vi "Data Monitor.vi"() -> ()   [LabVIEW 2018]
uses:
  Controls/Power Analyser Enum.ctl
  Controls/DUBAS FGV STATES.ctl
  Controls/DUBAS DTALOG FGV STATES.ctl
  SubVI/Hoiki/Conotrls/States.ctl
  Controls/READ CAN DATA.ctl
  Controls/Calculated Limits.ctl
  Controls/Main Tab.ctl
  <vilib>/FPGAPlugInAG/NI 9148/niLvFpga_Open_NI 9148.vi
  <vilib>/rvi/interface/common/dynamic/niFpgaDynamicAddResources.vi
  <vilib>/FPGAPlugInAG/Dynamic/niLvFpga_Reset_Dynamic.vi
  <vilib>/Utility/xml.llb/Read From XML File(string).vi
  Global/Throttle.vi
  <vilib>/Utility/file.llb/Write Delimited Spreadsheet (string).vi
  <vilib>/rvi/errors/niLvFpgaAdjustHostInterfaceError.vi
  <vilib>/FPGAPlugInAG/Dynamic/niLvFpga_Run_Dynamic.vi
  <vilib>/rvi/interface/common/niFpgaWaitOnOcc.vi
  <vilib>/Utility/file.llb/Read Delimited Spreadsheet (string).vi
  <vilib>/FPGAPlugInAG/Dynamic/niLvFpga_Close_Dynamic.vi
  <vilib>/rvi/interface/nirviOpenFPGA/nirviOpenFPGA.xnode
  FPGA Bitfiles/MAIN MEASUREMENT.lvbitx
  <vilib>/rvi/interface/nirviMethod/nirviMethod.xnode
  <vilib>/rvi/interface/nirviReadWriteControl/nirviReadWriteControl.xnode
  <vilib>/rvi/interface/nirviCloseFPGA/nirviCloseFPGA.xnode
  <vilib>/rvi/interface/Simulation/niFpgaSimulationCallBeginRW.vi
  <vilib>/rvi/errors/niLvFpgaMergeErrorWithErrorCode.vi
  <vilib>/FPGAPlugInAG/Dynamic/niLvFpga_ReadFifo_Dynamic.vi
  NiFpgaLv.dll
  <vilib>/FPGAPlugInAG/Dynamic/niLvFpga_ConfigureFifo_Dynamic.vi
  <vilib>/FPGAPlugInAG/Dynamic/niLvFpga_StopFifo_Dynamic.vi
  <vilib>/FPGAPlugInAG/Dynamic/niLvFpga_StartFifo_Dynamic.vi
  <vilib>/Utility/file.llb/Read Delimited Spreadsheet (I64).vi
panel:
  out "deleted portion 2":dbl[](array[numeric])
  out "deleted portion":dbl[](array[numeric])
  out "error out 2":errorcluster
  out "x*y":u32
  out "Array":string[](array[string])
  out "Thermocouple Spare":cluster{"String":string, "Scalar":sgl}[](array[cluster])
  out "Thermocouple":cluster{"String":string, "Scalar":sgl}[](array[cluster])
  out "9220 AI Volt Spare":cluster{"String":string, "Scalar":sgl}[](array[cluster])
  out "9208 AI Current":cluster{"String":string, "Scalar":sgl}[](array[cluster])
  out "9220 AI  Volt  Pressure":cluster{"String":string, "Scalar":sgl}[](array[cluster])
  in  "Data log":enum16{"1 Hz", "10 Hz"}(ring)
  in  "Settings Button":bool
  in  "Tab Control":T1(tab)
  out "Speed Torque":cluster{"Numeric":dbl, "Numeric":dbl}(graph)
  out "P DC(W)":dbl format="%_3g"
  out "P123(W)":dbl format="%_3g"
  out "P3(W)":dbl format="%_3g"
  out "P2(W)":dbl format="%_3g"
  out "P1(W)":dbl format="%_3g"
  out "VOLTAGE":string
  out "CURRENT":string
  out "POWER":string
  out "CONTROL SELECTION":string
  out "HVHC SELECTION":string
  out "PA Data":dbl[](array[numeric])
  in  "precision":i16
  out "Torque":string
  in  "precision":i16
  out "Power":string
  out "Intercooler_Out_T":sgl(slide) caption="T_intercooler_Out" scale=0.0..1000.0
  out "Intercooler_In_T":sgl(slide) caption="T_Oil Gallery" scale=0.0..1000.0
  out "Exhaust_T":sgl(slide) caption="T_Intercooler _In" scale=0.0..1000.0
  out "Oil_T":sgl(slide) caption="T_Coolant _OUT" scale=0.0..1000.0
  out "Coolant_Outlet_T":sgl(slide) caption="T_Coolant _IN" scale=0.0..1000.0
  out "Coolant_Inlet_T":sgl(slide) caption="T_intercooler_out" scale=0.0..1000.0
  out "Basement_T":sgl(slide) caption="T_Exhaust_Tail pipe" scale=0.0..1000.0
  out "Thermocouple Spare":string[](array[string])
  out "Thermocouple Spare":sgl[](array[numeric])
  out "Thermocouple":string[](array[string])
  out "Thermocouple":sgl[](array[numeric])
  out "9220 AI Volt Spare":string[](array[string])
  out "9220 AI Volt Spare":sgl[](array[numeric])
  out "9208 AI Current":string[](array[string])
  out "9208 AI Current":sgl[](array[numeric])
  out "9220 AI  Volt  Pressure":string[](array[string])
  out "9220 AI  Volt  \nPressure":sgl[](array[numeric])
  out "Universal AI":string[](array[string])
  out "9219 Universal AI":sgl[](array[numeric])
  in  "Column Header":string[](array[string])=["Time", "Throttle % ", "Speed Summary", "Torque Summary", "Power", "Gear Ratio", "Engine Speed", "Engine Torque", "L Speed", "R Speed", "H Speed", "L Torque ", "R Torque ", "H Torque ", "Intercooler_In_T", "Intercooler_Out_T", "Exhaust_T", "Oil_T", "Coolant_Inlet_T", "Coolant_Outlet_T", "Basement_T", "T Spare 1", "T Spare 2", "T Spare 3", "T Spare 4", "T Spare 5", "T Spare 6", "T Spare 7", "T Spare 8", "Coolant-In_P", "Coolant-Out_P", "Exhaust_P", "Oil_P", "Intercooler-In_P", "Intercooler-Out_P", "Misc_P ", "P Spare 1", "P Spare 2", "P Spare 3", "P Spare 4", "Engine RPM "]
  out "STOP BOTH APP":bool
  out "P Spare 4":sgl
  out "P Spare 3":sgl
  out "P Spare 2":sgl
  out "P Spare 1":sgl
  out "T Spare 8":sgl
  out "T Spare 7":sgl
  out "T Spare 6":sgl
  out "T Spare 5":sgl
  out "T Spare 4":sgl
  out "T Spare 3":sgl
  out "T Spare 2":sgl
  out "T Spare 1":sgl
  in  "Gear Ratio":dbl=1.0
  out "Torque":i32
  out "Speed":i32
  in  "File Tag":string
  out "speed torque power":dbl[](array[numeric])
  out "H Speed":dbl(knob) scale=0.0..7500.0
  out "Speed Summary":dbl(knob) scale=0.0..8000.0
  out "Torque Summary":dbl(knob) scale=-500.0..1000.0
  out "Power":dbl(knob) scale=0.0..300.0
  in  "Safety Limits":bool
  in  "Alarms & warning":string(combo)
  out "RAW Mean TC":sgl[](array[numeric]) format="%#.2g"
  out "RAW Mean":sgl[](array[numeric])
  out "Mean tc":sgl[](array[numeric]) format="%#.2g"
  out "Timeout Counter":u64
  out "error out":errorcluster
  out "Engine RPM":sgl caption="Gauge"
  out "Stop All":bool
  out "Mean":sgl[](array[numeric]) format="%#.2g"
  out "AI0":sgl
  out "AI1":sgl
  out "AI2":sgl
  out "Mod1/CH0":sgl
  out "Mod1/CH1":sgl
  out "Mod1/CH2":sgl
  out "Mod1/CH3":sgl
  out "Intercooler-Out_P":sgl(slide) caption="P_Exhaust_TailPipe" scale=0.0..10.0 scale format="%#1_6g"
  out "Misc_P":sgl(slide) caption="P_Before cat" scale=0.0..10.0 scale format="%#1_6g"
  out "Oil_P":sgl(slide) caption="P_Intercooler_In" scale=0.0..10.0 scale format="%#1.1g"
  out "Exhaust_P":sgl(slide) caption="P_Coolant_OUT" scale=0.0..5.0 scale format="%#1_6g"
  out "Coolant-Out_P":sgl(slide) caption="P_Oil Gallery" scale=0.0..5.0
  out "Intercooler-In_P":sgl(slide) caption="P_Intercooler_out" scale=0.0..10.0 scale format="%2d"
  out "Coolant-In_P":sgl(slide) caption="P_Coolant_IN" scale=0.0..5.0
  in  "Data_Log":bool
  out "Saftey_Lim_error":bool
  in  "Stop":bool
  # "NVH TEST DATA MONITOR"
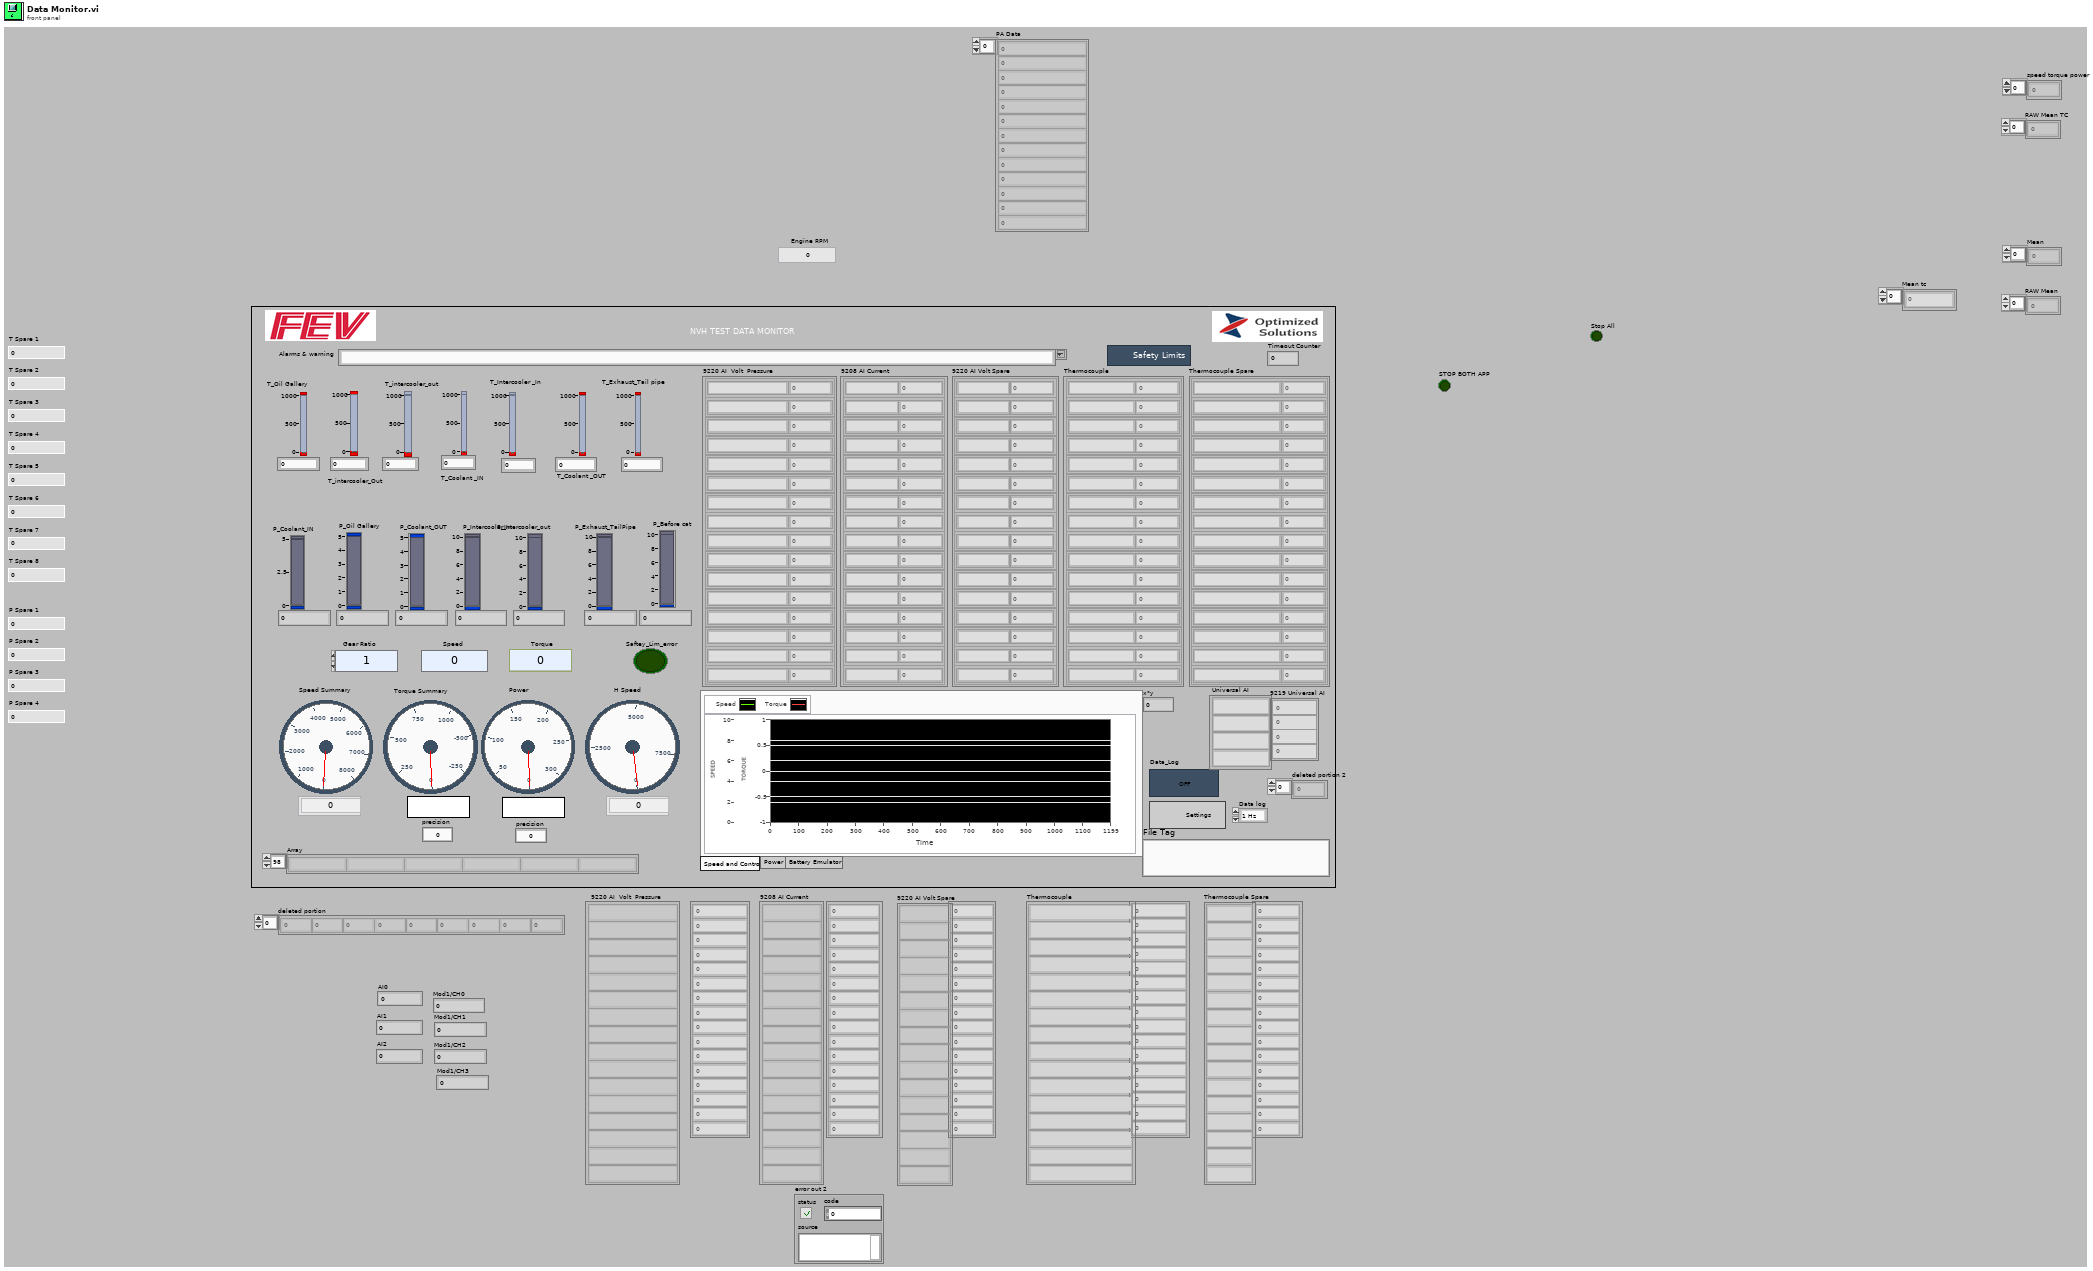
[diagram p1: front panel]
types:
  T1 = enum32{"Speed and Control", "Power", "Battery Emulator"}
  T2 = typedef "DUBAS FGV STATES.ctl" = enum16{"OPEN REF", "READ DATA", "CLOSE"}
  T3 = cluster{"Item":enum16{"Urms", "Umn", "Uac", "Udc", "Ufnd", "Upk+", "Upk-", "Uthd", "Urf", "Uunb", "Irms", "Imn", "Iac", "Idc", "Ifnd", "Ipk+", "Ipk-", "Ithd", "Irf", "Iunb", "P", "S", "Q", "PF", "DEG U", "DEG I", "DEG P", "f", "EFFI", "LOSS", "IH+", "IH-", "IH", "WP+", "WP-", "WP", "CH A", "CH B", "Pm", "Slip", "Laptime", "Laptime(ms)"}, "Ch(0:Ch1)":enum16{"1", "2", "3", "4", "12", "34", "123"}}[]
  T4 = typedef "Power Analyser Enum.ctl" = enum16{"READ", "WRITE"}
  T5 = typedef "States.ctl" = enum16{"Open Com", "Read Data", "Close Comm"}
  T6 = enum16{"Initialise", "Read Data", "Write Data", "Close"}
  T7 = enum32{"Invalid", "Standard", "Closed", "Hidden", "Minimized", "Maximized"}
  T8 = enum32{"invalid app kind", "Development System", "Run Time System", "Student Edition", "Embedded LabVIEW", "Evaluation", "Custom"}
  T9 = typedef "Calculated Limits.ctl" = cluster{"1LF":dbl, "1HW select":bool, "1LW select":bool, "1LF select":bool, "1HW":dbl, "1LW":dbl, "1HF":dbl, "1HF select":bool, "CH1":string, "1_LF_EVENT":string, "1_HF_EVENT":string}
  T10 = typedef "Limit Paths.ctl" = cluster{"Limit 1 Config Path":path, "Limit 2 Config Path ":path, "Limit 3 Config Path ":path, "Limit 4 Config Path ":path, "Limit 5 Config Path ":path, "Limit 6 Config Path ":path, "CallimitPath ":path}
  T11 = cluster{"appended path":path, "Core":cluster{"Current VI Reference":refnum<vi>, "Close Panel on Exit?":bool}, "AILimitConfig":cluster{"1LF":dbl, "1HW select":bool, "1LW select":bool, "1LF select":bool, "1HW":dbl, "1LW":dbl, "1HF":dbl, "1HF select":bool, "CH1":string, "1_LF_EVENT":string, "1_HF_EVENT":string}[], "GenHF ":string[], "GenLF ":string[], "Cal Limits":T9[], "Cal Limit Input":dbl[], "Channel Name":string[], "HF Actions":string[], "Lower Warning":string[], "Lower Fault":string[], "Higher Warning":string[], "Higher Fault":string[], "Input Values":sgl[], "Limit Path":T10, "Calculated value":sgl[], "Calculated LW ":string[], "Calculated HW ":string[], "Calculated LF ":string[], "Calculated GEN LF Events":string[], "Calculated HF ":string[], "Calculated GEN HF Events":string[], "Reset":bool}
  T12 = cluster{"1LF":dbl, "1HW select":bool, "1LW select":bool, "1LF select":bool, "1HW":dbl, "1LW":dbl, "1HF":dbl, "1HF select":bool, "CH1":string, "1_LF_EVENT":string, "1_HF_EVENT":string}[]
  T13 = cluster{"Current VI Reference":refnum<vi>, "Close Panel on Exit?":bool}
  T14 = typedef "Main Tab.ctl" = enum32{"H", "L", "R", "L-R", "H-L-R", "System"}
  T15 = typedef "DUBAS DTALOG FGV STATES.ctl" = enum16{"OPEN REF", "READ DATA", "WRITE DATA", "CLOSE"}
  T16 = enum8{"Enabled", "Disabled", "Disabled and Grayed Out"}
  T17 = typedef "READ CAN DATA.ctl" = enum16{"SET", "GET"}
  T18 = cluster{"Core":cluster{"Current VI Reference":refnum<vi>, "Close Panel on Exit?":bool}, "Intercooler_In_T":refnum<vi>, "Coolant_Inlet_T":refnum<vi>, "Coolant_Outlet_T":refnum<vi>, "Basement_T":refnum<vi>, "Exhaust_T":refnum<vi>, "Oil_T":refnum<vi>, "Intercooler_Out_T":refnum<vi>, "ExpansionChassFPGA":refnum<k20>, "Data Log":bool, "LogFile Refnum":refnum<file>, "Log Active":bool[][], "location":path}
  T19 = typedef "READ CAN CLUSTER.ctl" = cluster{"FUNCTION":string, "DATA":string}
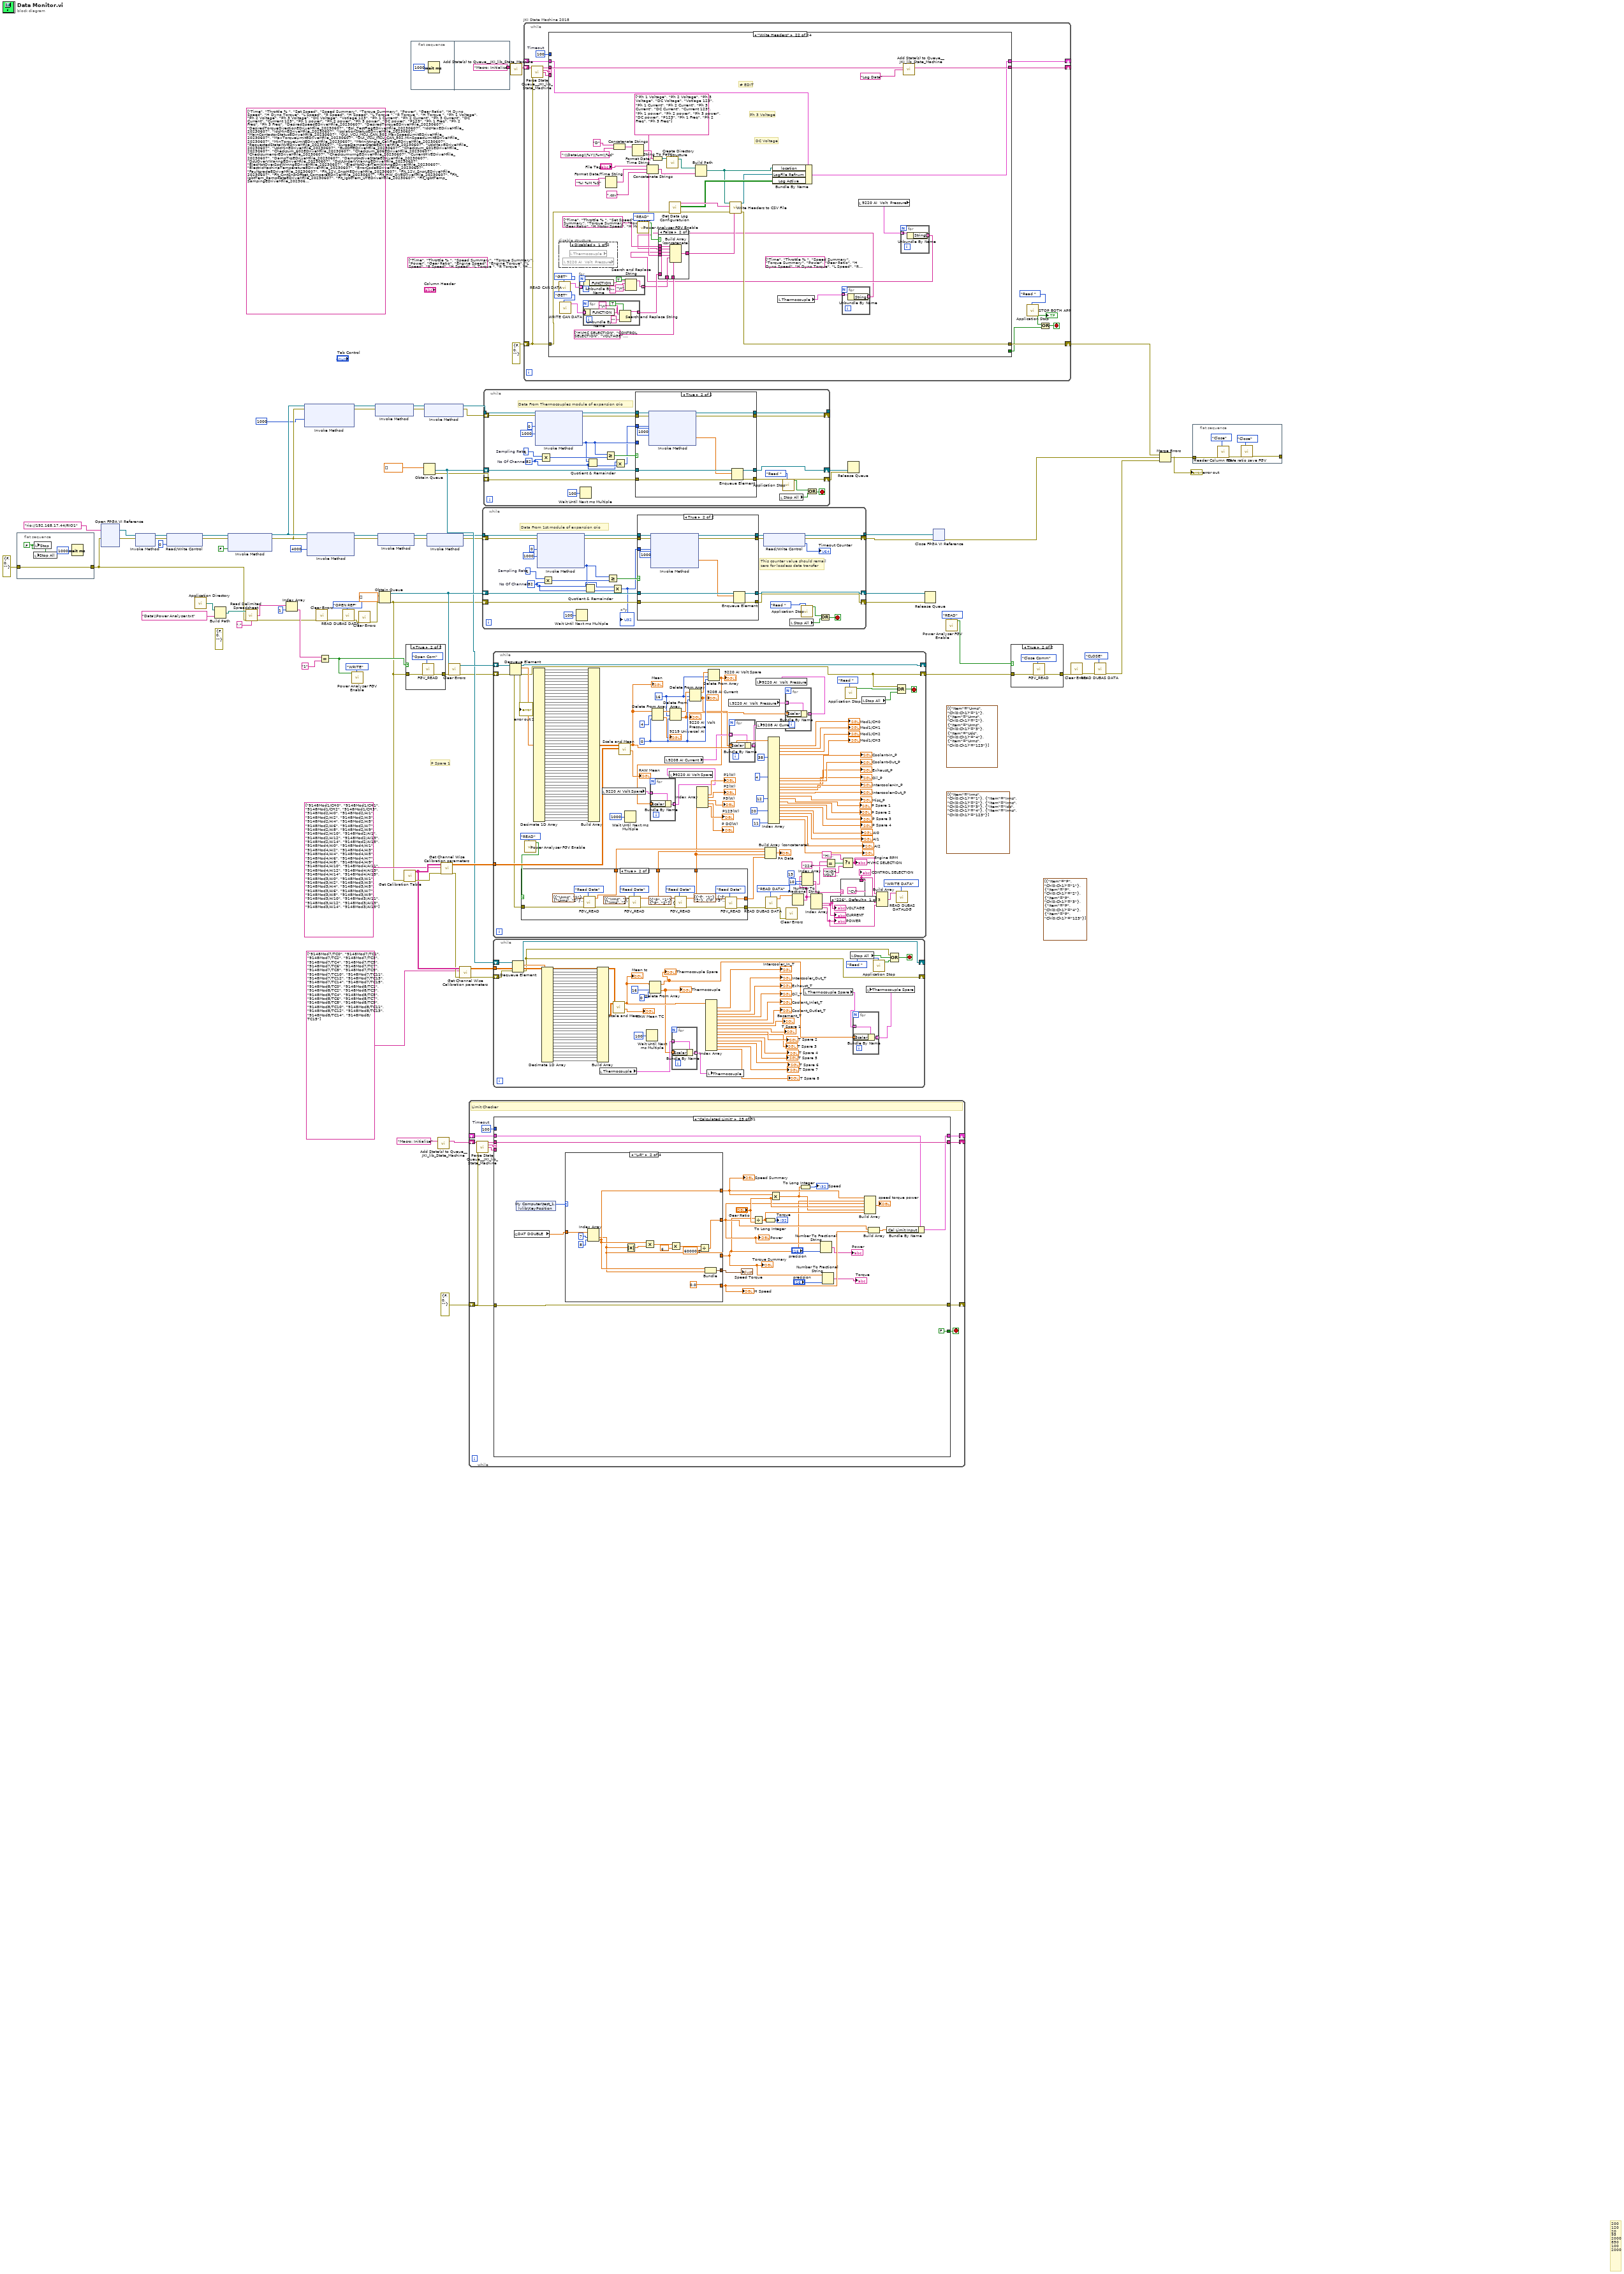
[diagram p0: block diagram]
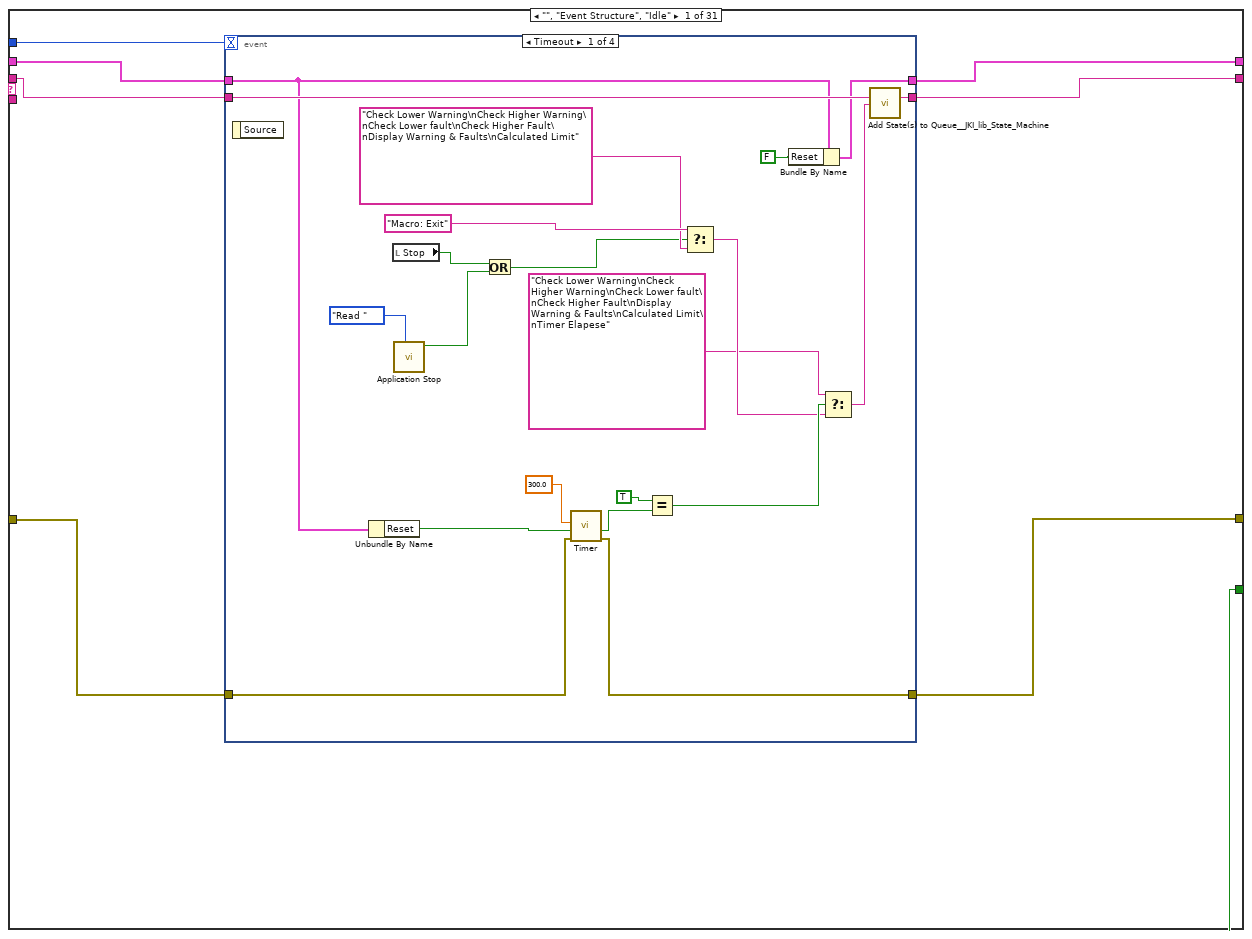
[diagram p2: hidden frame]
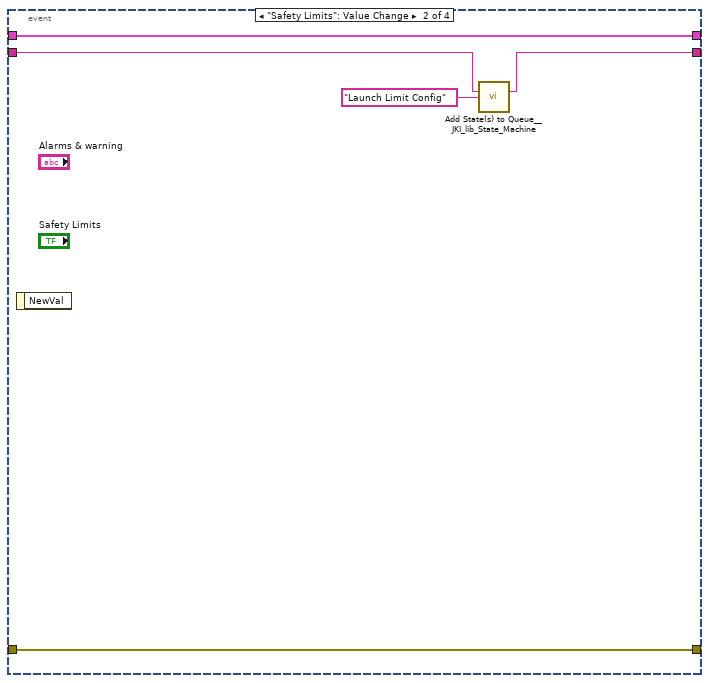
[diagram p3: hidden frame]
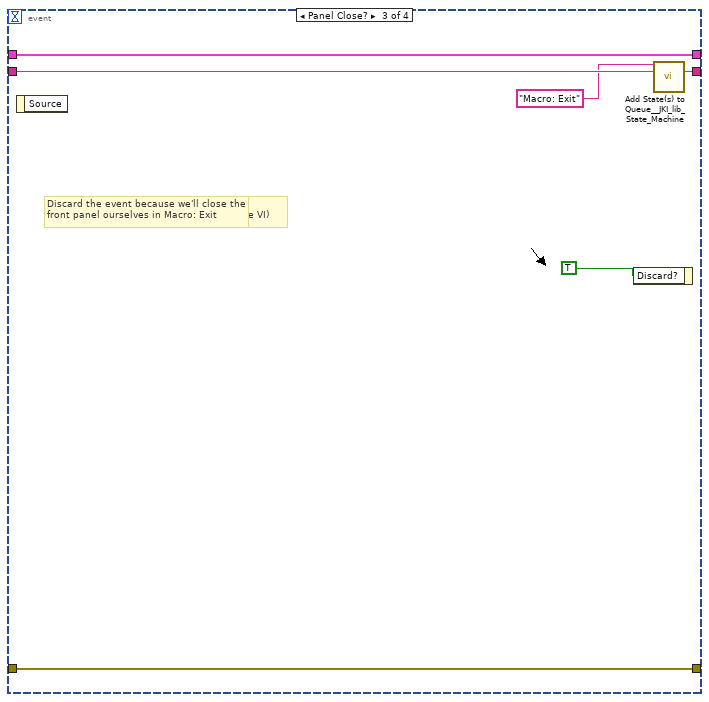
[diagram p4: hidden frame]
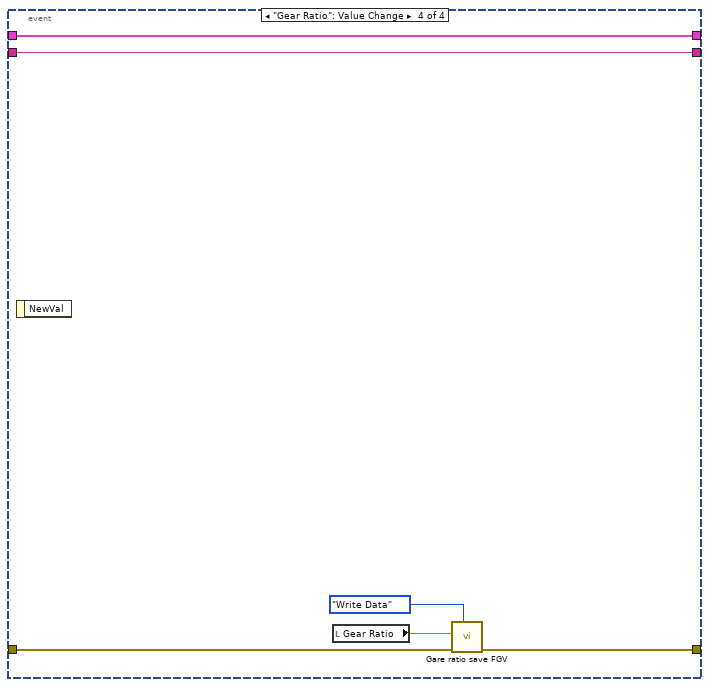
[diagram p5: hidden frame]
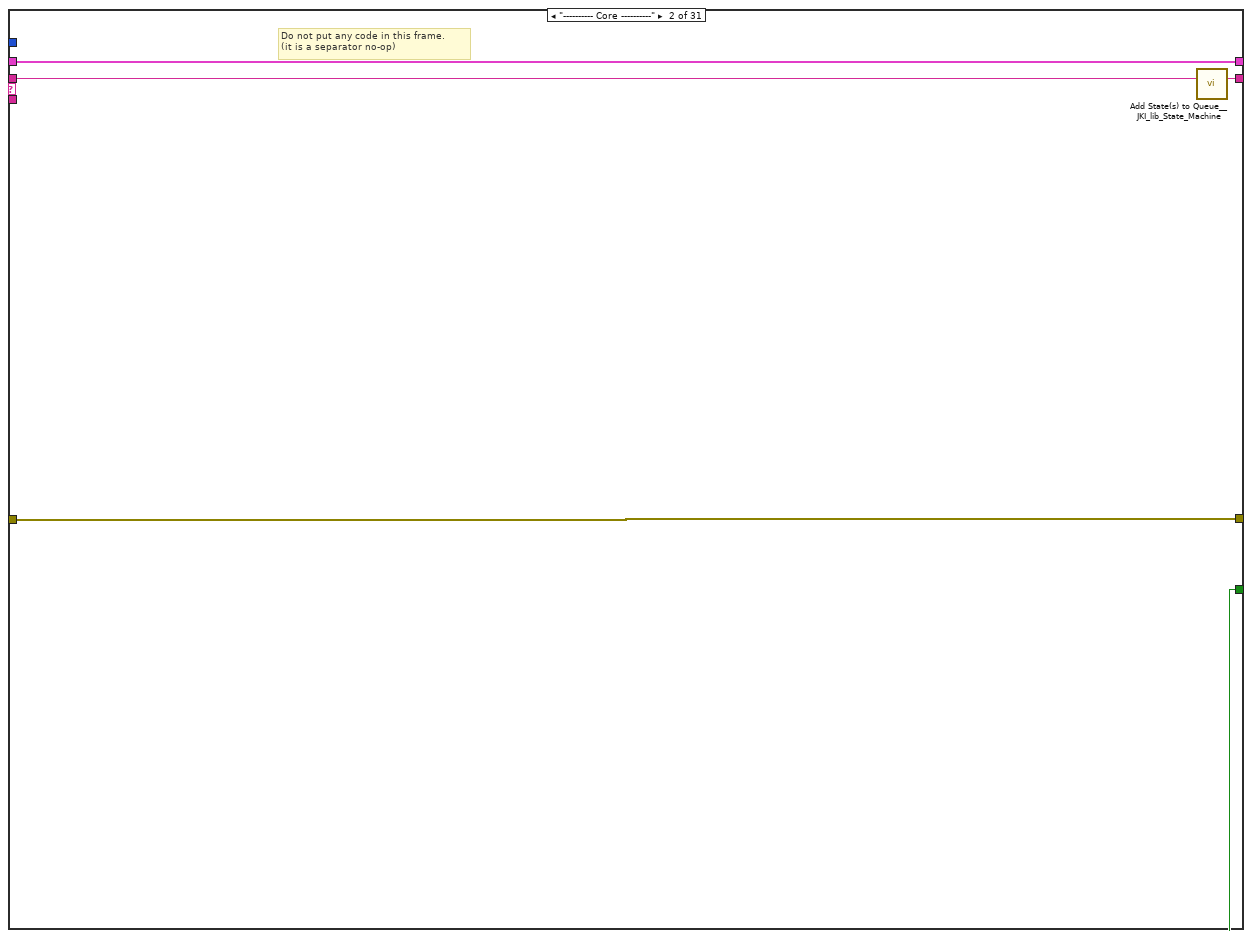
[diagram p6: hidden frame]
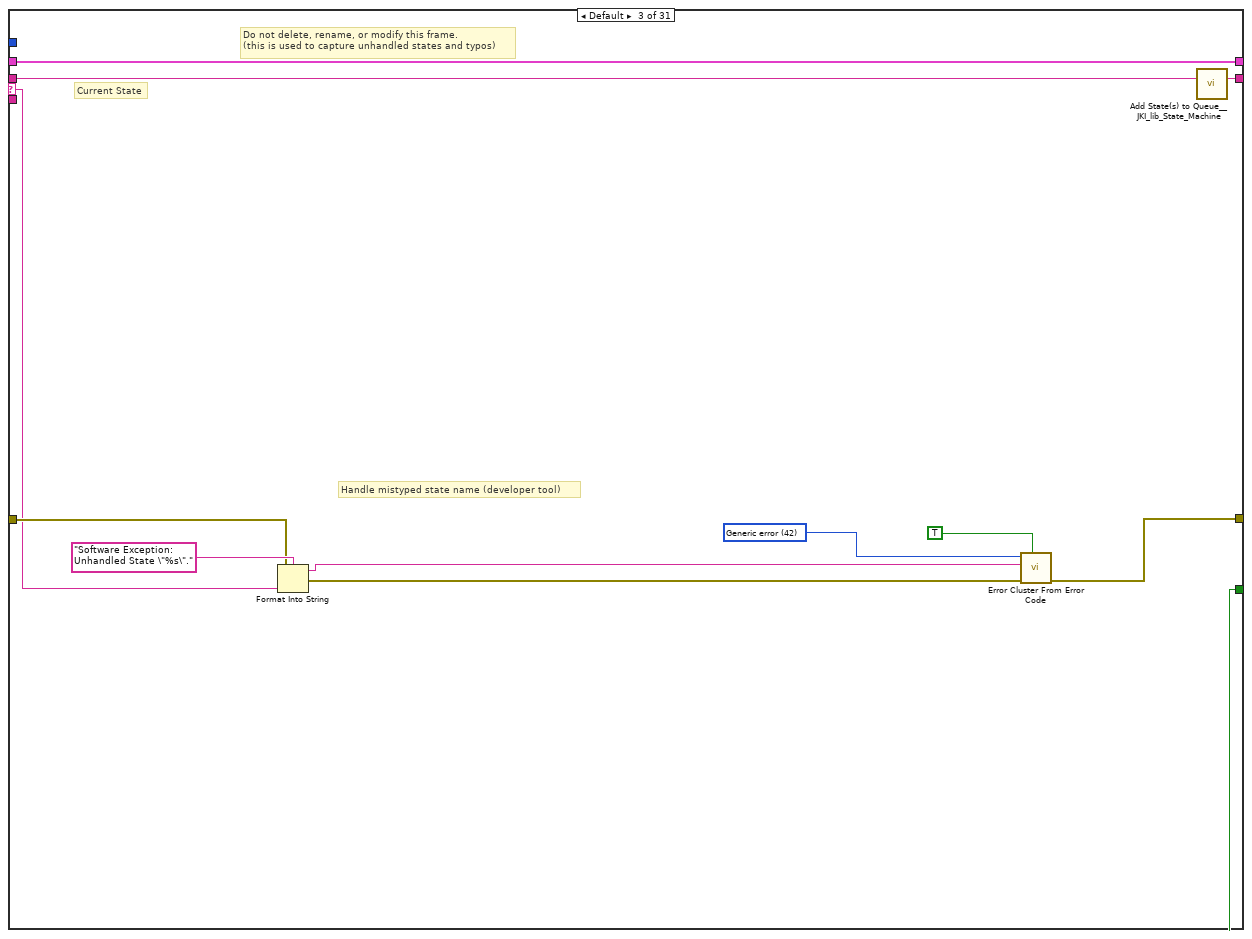
[diagram p7: hidden frame]
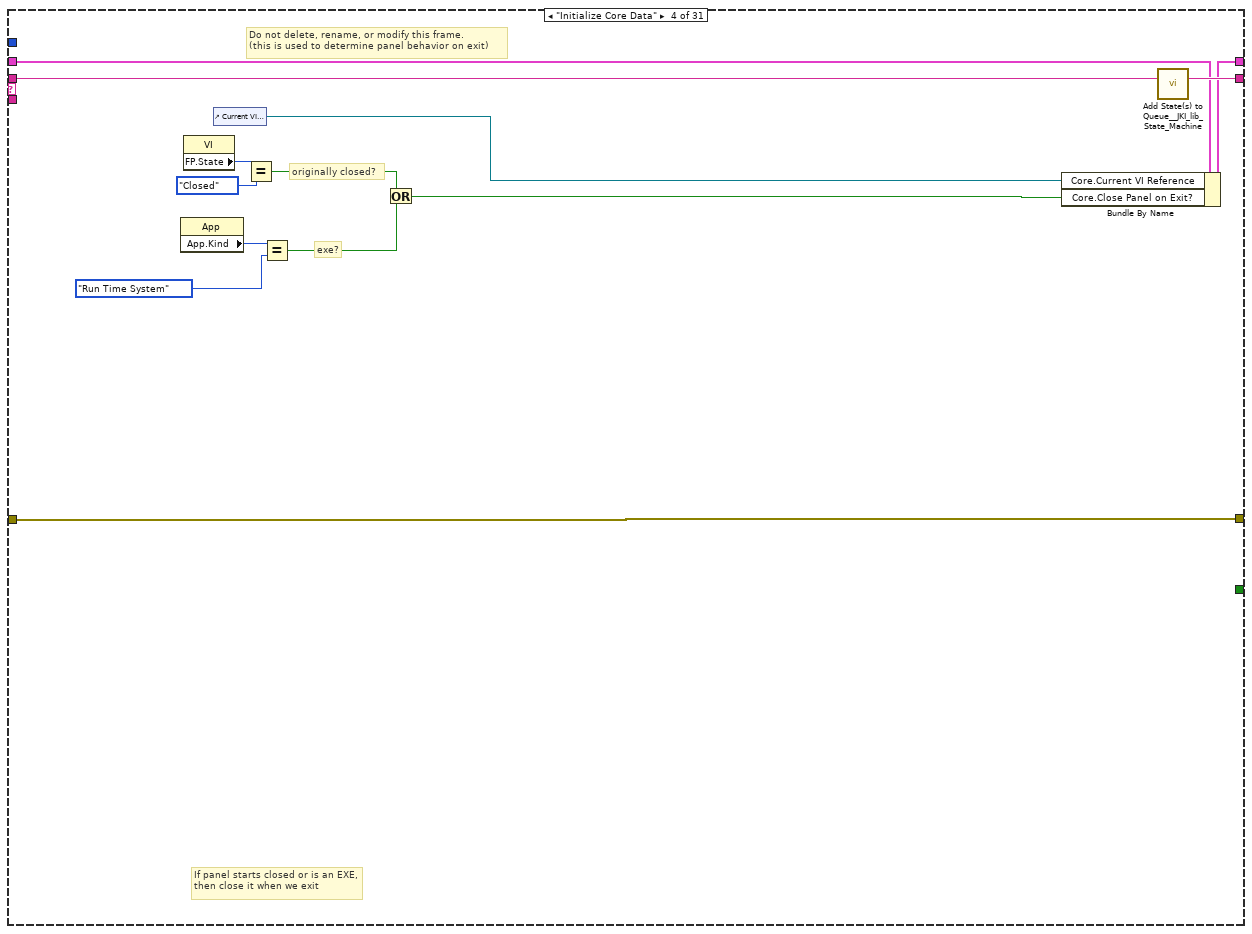
[diagram p8: hidden frame]
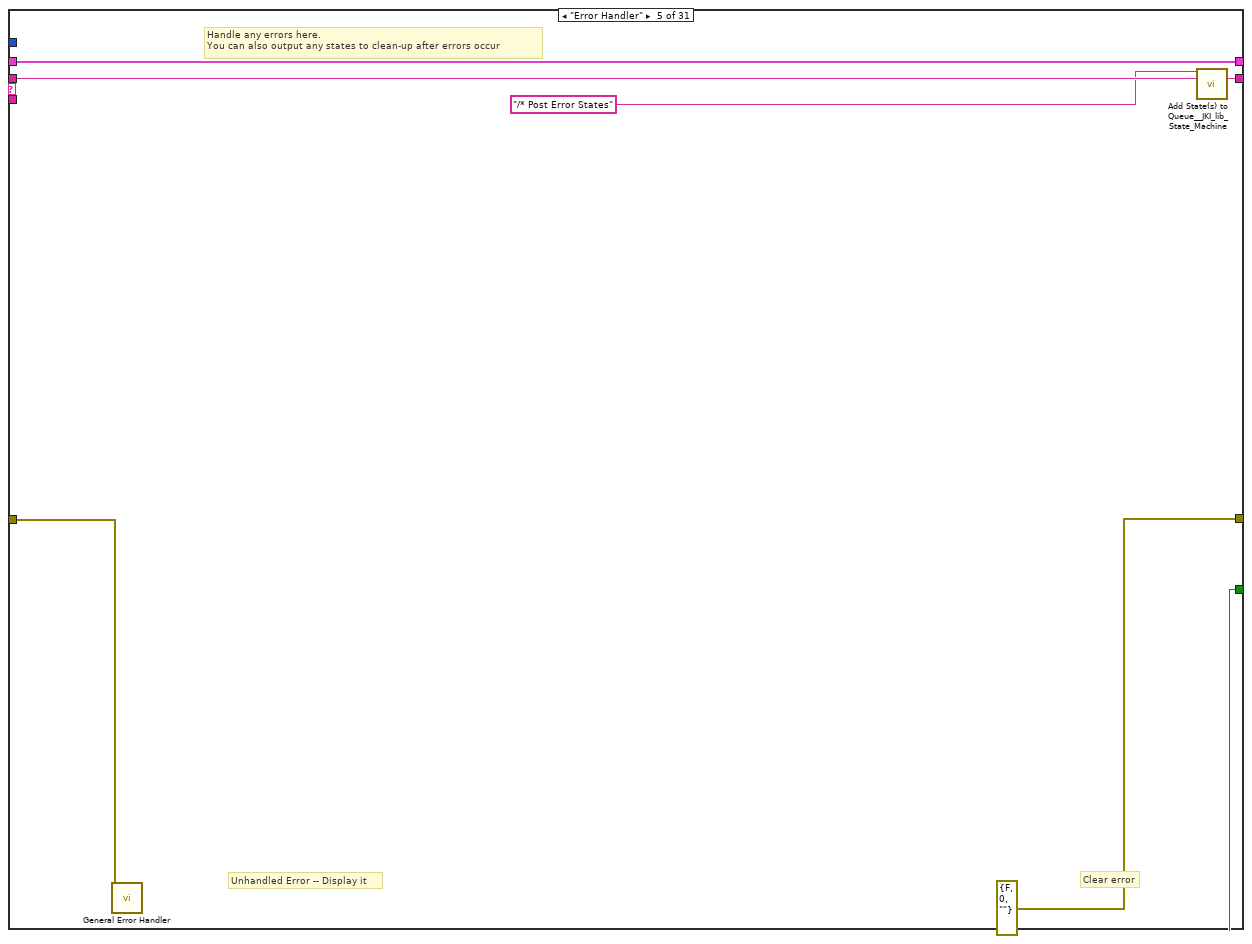
[diagram p9: hidden frame]
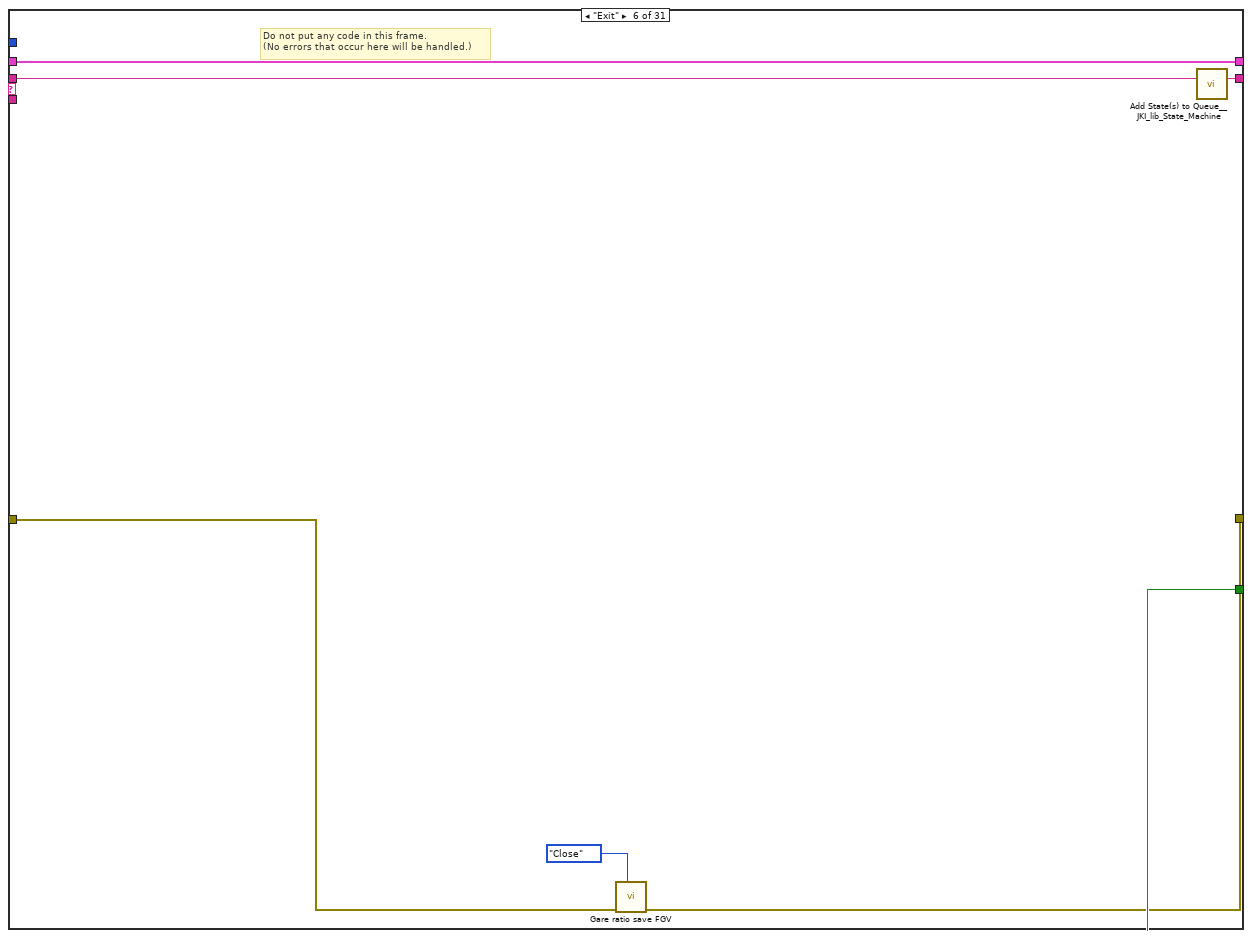
[diagram p10: hidden frame]
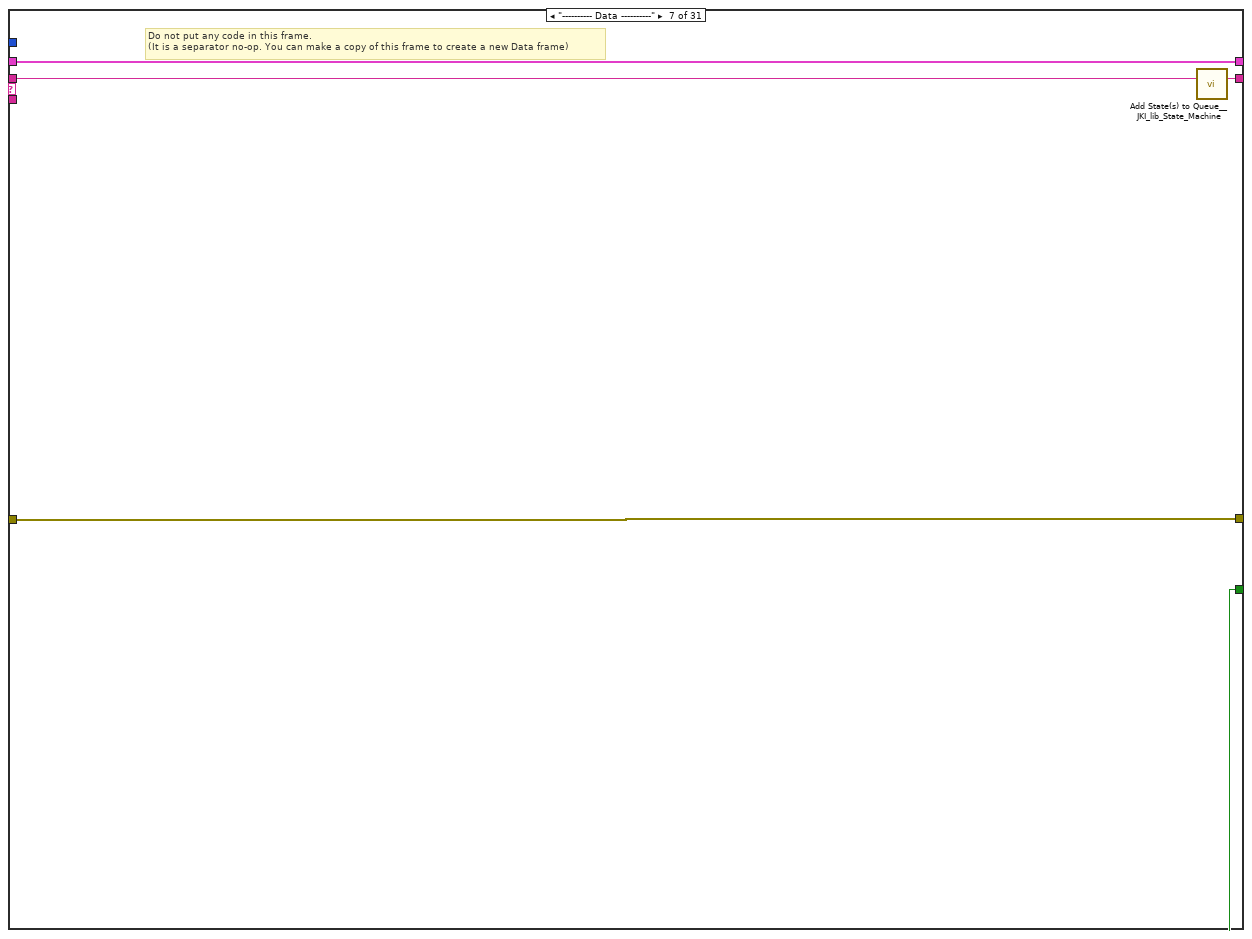
[diagram p11: hidden frame]
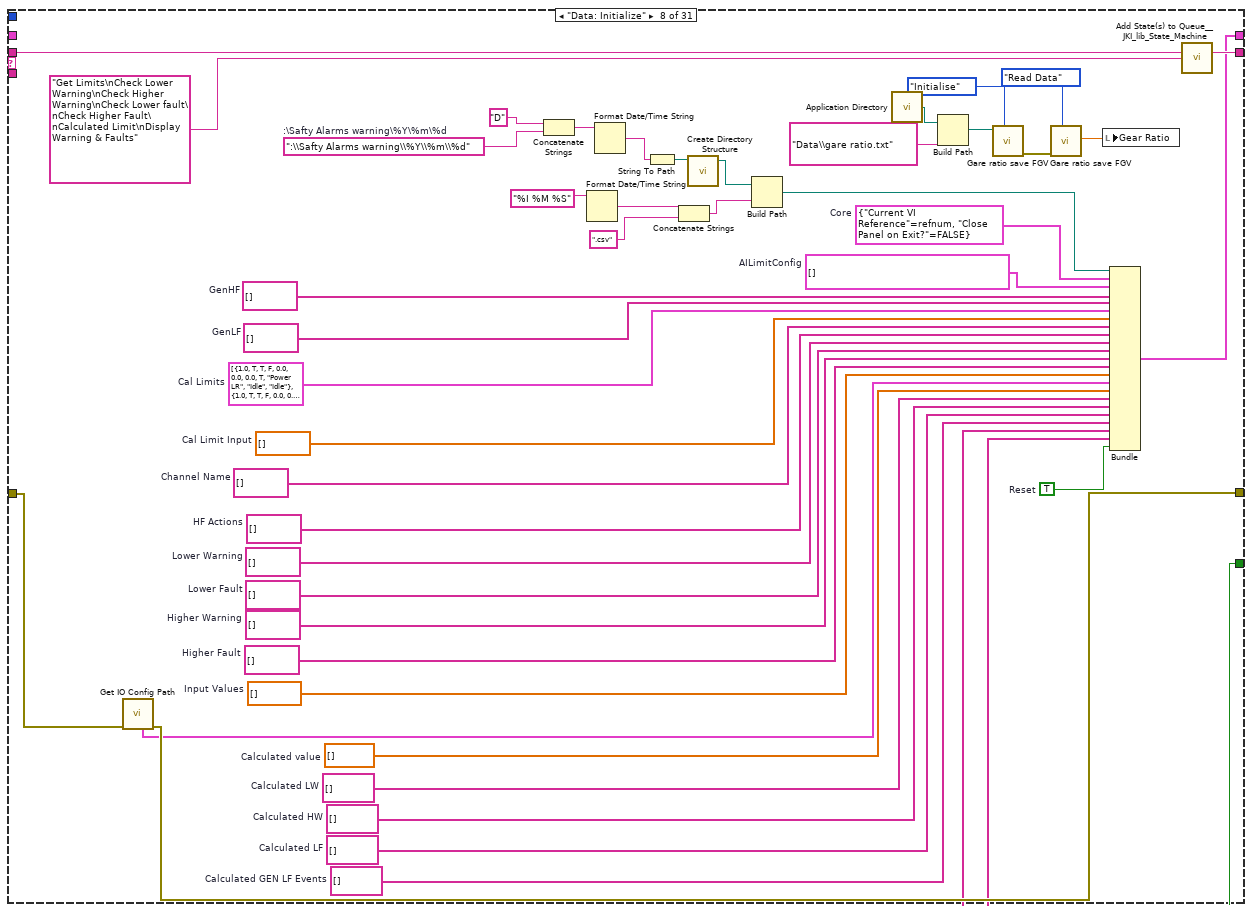
[diagram p12: hidden frame]
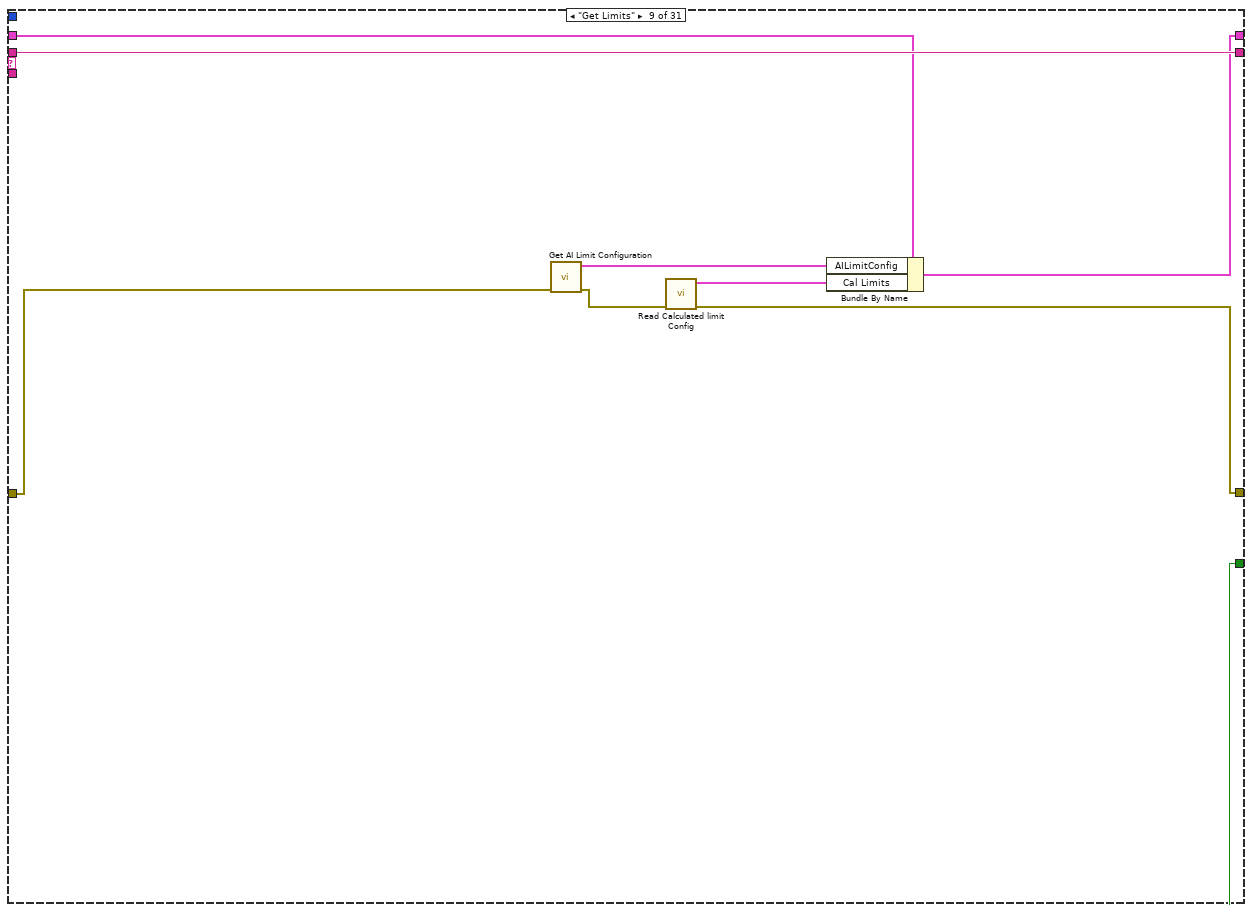
[diagram p13: hidden frame]
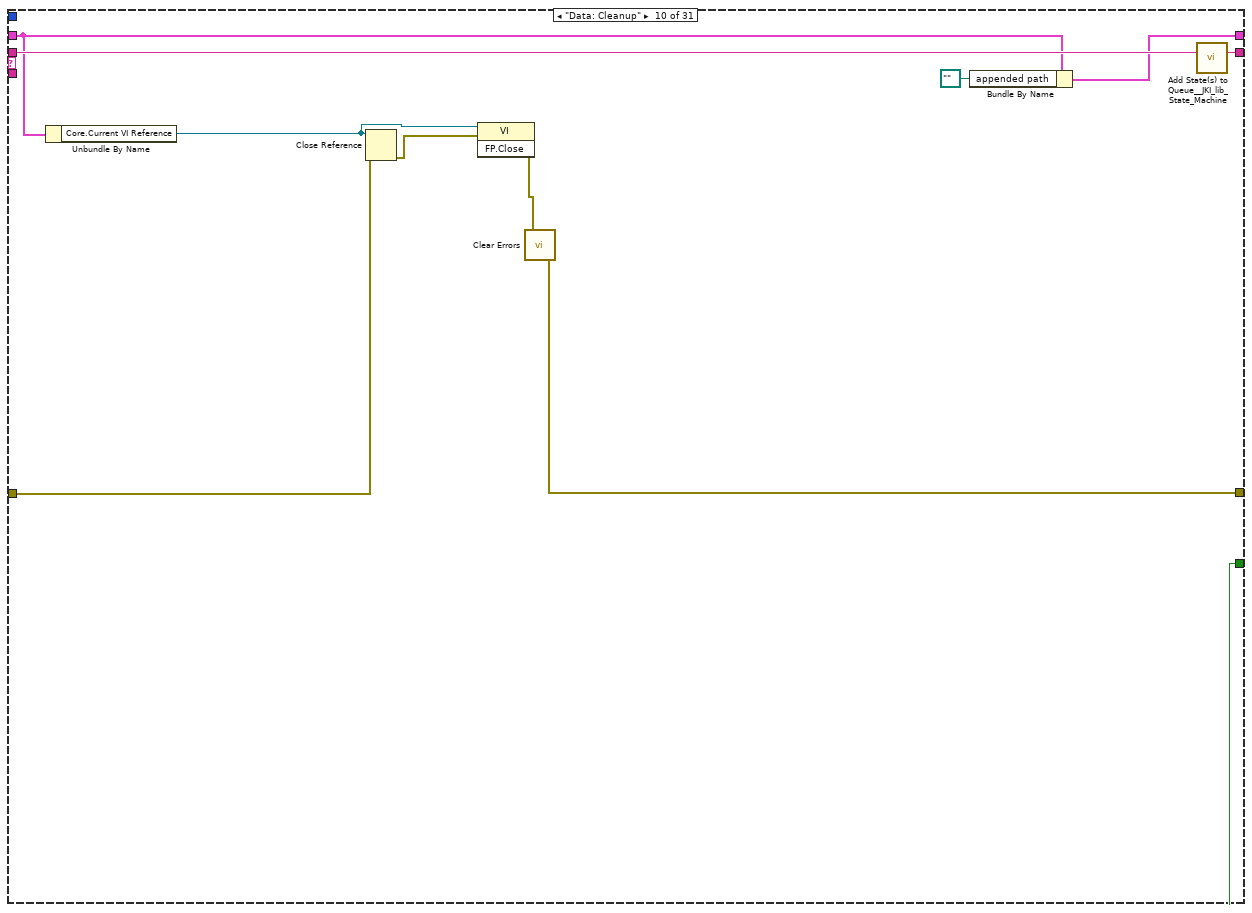
[diagram p14: hidden frame]
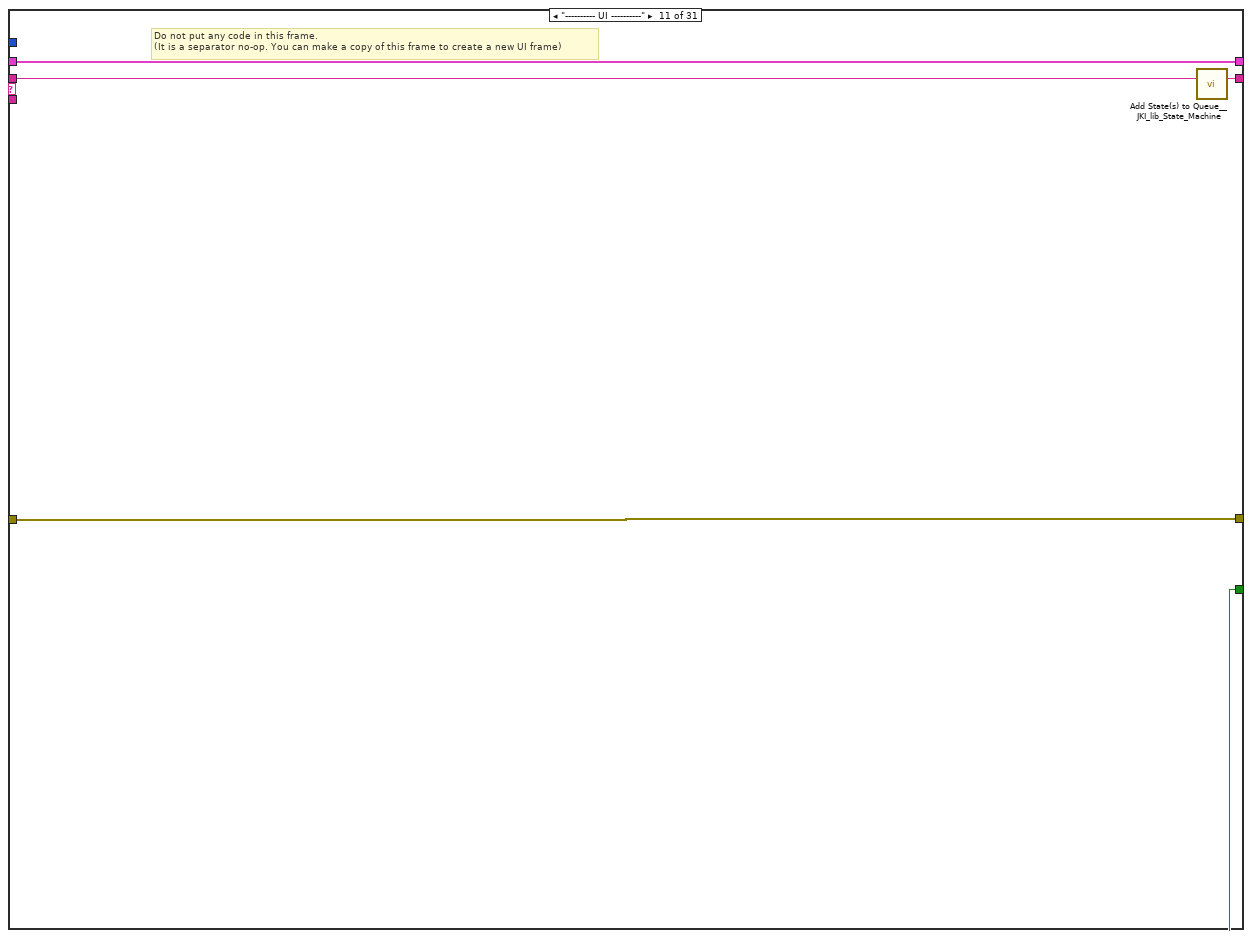
[diagram p15: hidden frame]
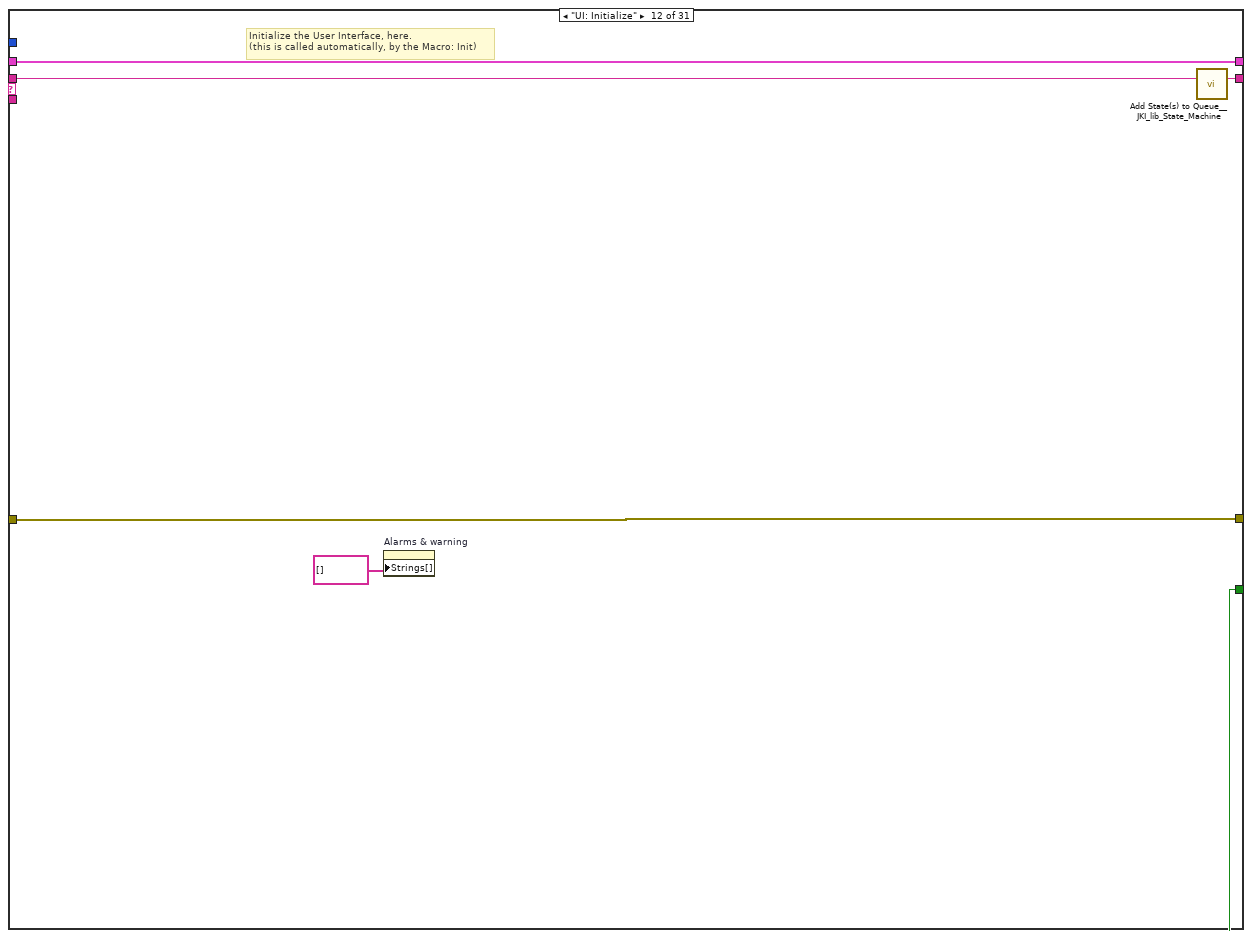
[diagram p16: hidden frame]
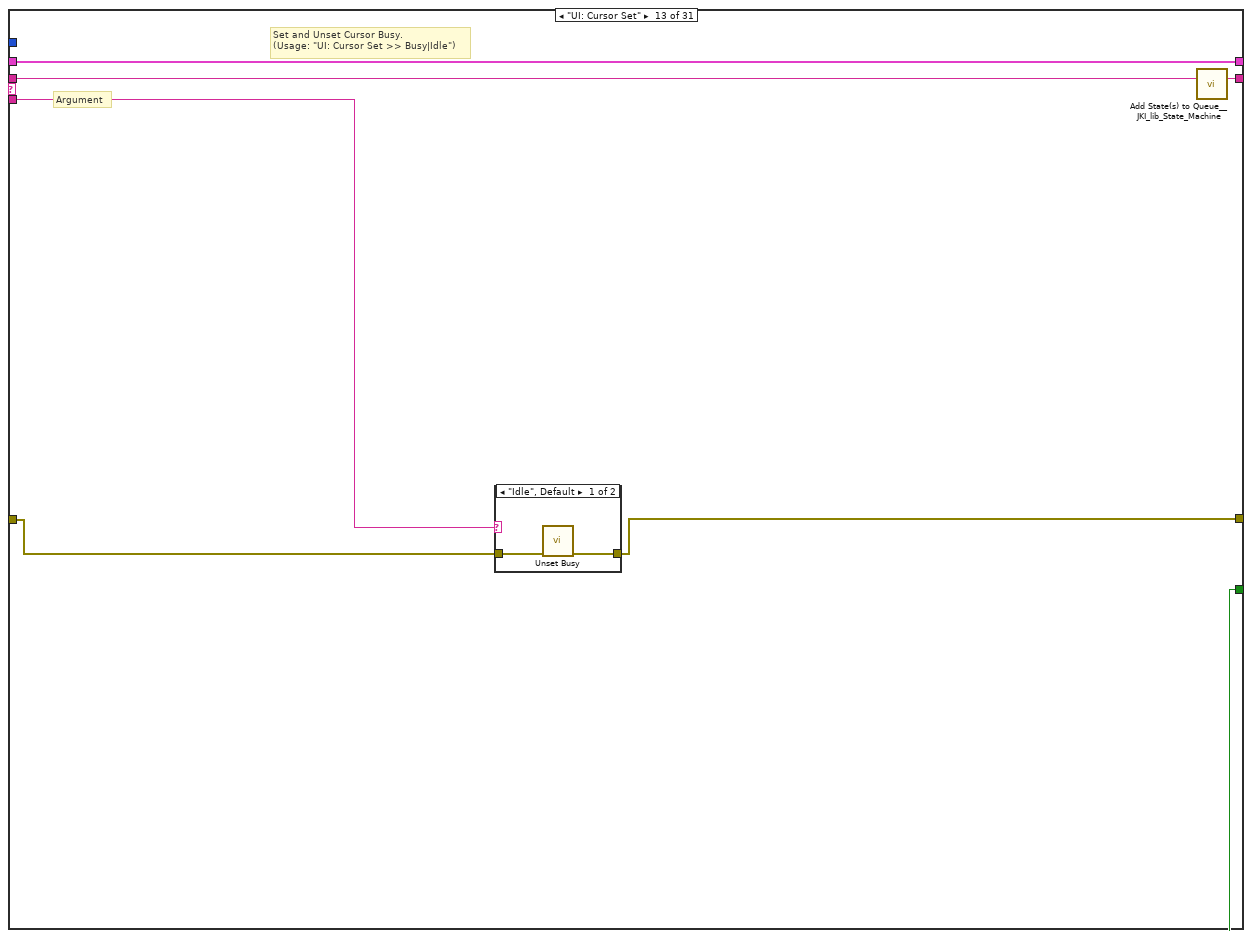
[diagram p17: hidden frame]
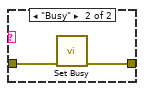
[diagram p18: hidden frame]
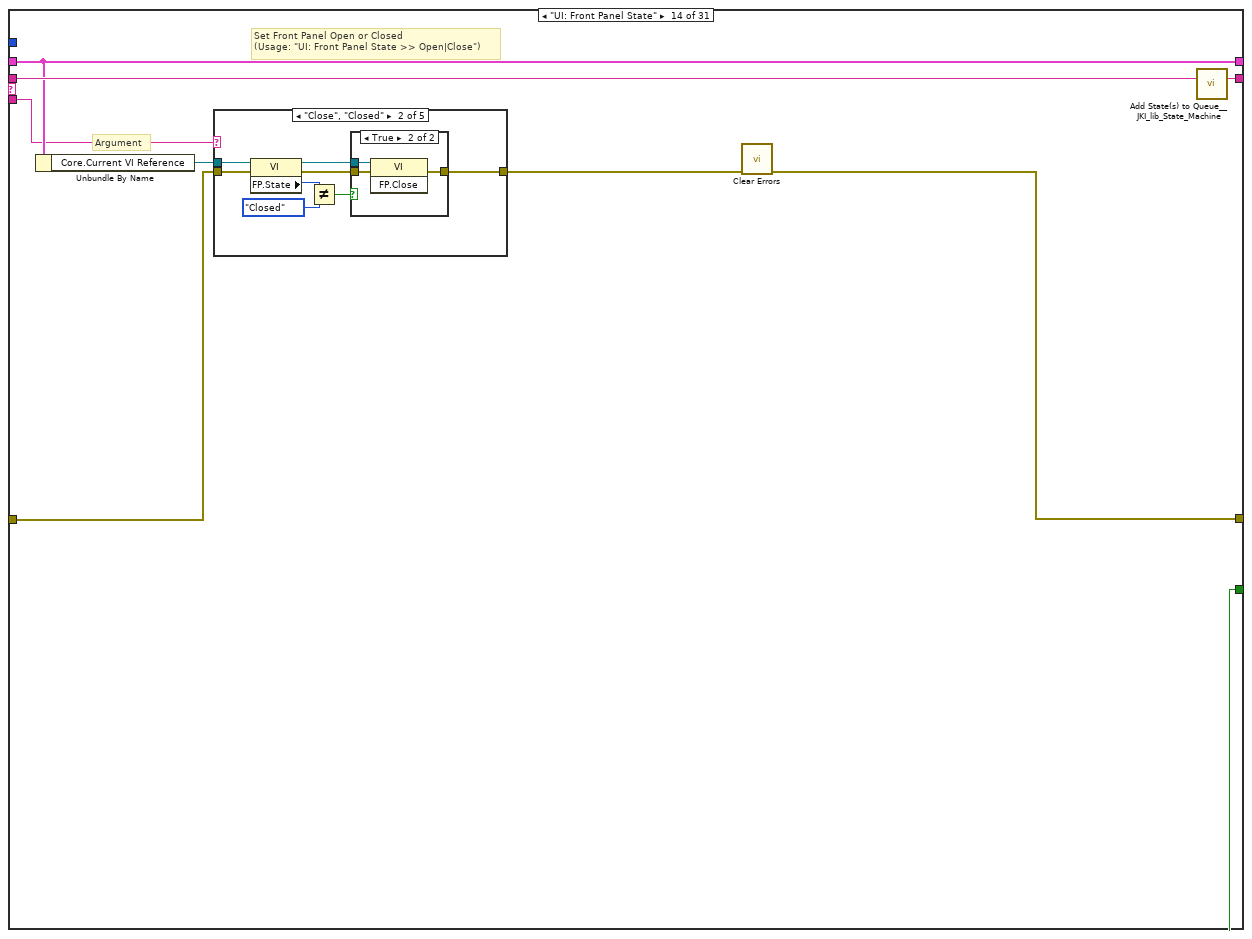
[diagram p19: hidden frame]
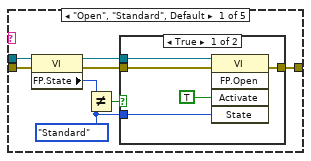
[diagram p20: hidden frame]
diagram:
  (unwired) T3 [{"Item"=enum."Urms", "Ch(0:Ch1)"=enum."1"}, {"Item"=enum."Urms", "Ch(0:Ch1)"=enum."2"}, {"Item"=enum."Urms", "Ch(0:Ch1)"=enum."3"}, {"Item"=enum."Udc", "Ch(0:Ch1)"=enum."4"}, {"Item"=enum."Urms", "Ch(0:Ch1)"=enum."123"}] ("Voltage")
  (unwired) T3 [{"Item"=enum."Irms", "Ch(0:Ch1)"=enum."1"}, {"Item"=enum."Irms", "Ch(0:Ch1)"=enum."2"}, {"Item"=enum."Irms", "Ch(0:Ch1)"=enum."3"}, {"Item"=enum."Idc", "Ch(0:Ch1)"=enum."4"}, {"Item"=enum."Irms", "Ch(0:Ch1)"=enum."123"}] ("Current")
  (unwired) errorcluster {"status"=FALSE, "code"=0, "source"=""} ("error in (no error)")
  (unwired) string[] ["Time", "Throttle % ", "Set Speed", "Speed Summary", "Torque Summary", "Power", "Gear Ratio", "H Dyno Speed", "H Dyno Torque", "L Speed", "R Speed", "H Speed", "L Torque ", "R Torque ", "H Torque ", "Ph 1 Voltage", "Ph 2 Voltage", "Ph 3 Voltage", "DC Voltage", "Votlage 123", "Ph 1 Current", "Ph 2 Current", "Ph 3 Current", "DC Current", "Currrent 123", "Ph 1 power", "Ph 2 power", "Ph 3 power", "DC power", "P123", "Ph 1 Freq", "Ph 2 Freq", "Ph 3 Freq", "DesiredSpeedEDriveMfile_20230607", "DesiredTorqueEDriveMfile_20230607", "DesiredTorqueDirectionEDriveMfile_20230607", "Eol_TestFlagEDriveMfile_20230607", "IdcMaxEDriveMfile_20230607", "IdcMinEDriveMfile_20230607", "IsolationStatusEDriveMfile_20230607", "MainContactorStatusEDriveMfile_20230607", "OUI_VCU_MCU_CAN_502.MaxSpeedLimitEDriveMfile_20230607", "MaxTorqueLimitEDriveMfile_20230607", "OUI_VCU_MCU_CAN_502.MinSpeedLimitEDriveMfile_20230607", "MinTorqueLimitEDriveMfile_20230607", "MtrInitAngle_CaliFlagEDriveMfile_20230607", "RequestedStateINVEDriveMfile_20230607", "SurgeDamperStateEDriveMfile_20230607", "UdcMaxEDriveMfile_20230607", "UdcMinEDriveMfile_20230607", "BusOffEDriveMfile_20230607", "Checksum_601EDriveMfile_20230607", "Checksum_602EDriveMfile_20230607", "Checksum_606EDriveMfile_20230607", "ChecksumerrorEDriveMfile_20230607", "ChecksumwrngEDriveMfile_20230607", "CurrentHVEDriveMfile_20230607", "DampTrqEDriveMfile_20230607", "DamptActiveStateEDriveMfile_20230607", "DcUOverVWanngEDriveMfile_20230607", "DcUUnderVWanngEDriveMfile_20230607", "ElecMotOverSpdWrnngEDriveMfile_20230607", "ElecMotOverTemWrnngEDriveMfile_20230607", "ElectricMachineTemperatureEDriveMfile_20230607", "ErrorCodeEDriveMfile_20230607", "FaultgradeEDriveMfile_20230607", "Flt_12V_SnsrHEDriveMfile_20230607", "Flt_12V_SnsrLEDriveMfile_20230607", "Flt_CrntSnsrOffset_CompareEDriveMfile_20230607", "Flt_HW_OVEDriveMfile_20230607", "Flt_IgbtTem_RampRateEDriveMfile_20230607", "Flt_IgbtTem_UTEDriveMfile_20230607", "Flt_IgbtTemp_SampingEDriveMfile_20230607", "Flt_MessageCounterEDriveMfile_20230607", "Flt_PhaseCrnt_SumEDriveMfile_20230607", "Flt_V1p3V_HEDriveMfile_20230607", "Flt_V1p3V_LEDriveMfile_20230607", "FluxWeak_FactorEDriveMfile_20230607", "IGBTOverTemWrnngEDriveMfile_20230607", "IGBTTemSnsrFltEDriveMfile_20230607", "INV12VSuppyLVEDriveMfile_20230607", "INV12VSuppyOVEDriveMfile_20230607", "INV15VSuppyLVEDriveMfile_20230607", "INV15VSuppyOVEDriveMfile_20230607", "INV5VSuppyLVEDriveMfile_20230607", "INV5VSuppyOVEDriveMfile_20230607", "INVDschrgFltEDriveMfile_20230607", "INVOverVolFltEDriveMfile_20230607", "INVPwrModuFltEDriveMfile_20230607", "INVVolSnsrFltEDriveMfile_20230607", "Id_FBEDriveMfile_20230607", "Id_RefEDriveMfile_20230607", "InitAngleOffsetEDriveMfile_20230607", "InverterTemperatureEDriveMfile_20230607", "Iq_FBEDriveMfile_20230607", "Iq_RefEDriveMfile_20230607", "LostCommWithVCUEDriveMfile_20230607", "MCU_InitialErrEDriveMfile_20230607", "MaxTorqueEDriveMfile_20230607", "MessageCounter_606EDriveMfile_20230607", "MinTorqueEDriveMfile_20230607", "MotOverCrntFltEDriveMfile_20230607", "MotOverCrntFltHardEDriveMfile_20230607", "MotOverSpdFltEDriveMfile_20230607", "MotOverTemFltEDriveMfile_20230607", "MotRotBlockFltEDriveMfile_20230607", "MotRsovrFltEDriveMfile_20230607", "MotTemSnsrFltEDriveMfile_20230607", "MtrSpdFilt_NoFiltEDriveMfile_20230607", "OutputSpeedEDriveMfile_20230607", "OutputTorqueEDriveMfile_20230607", "PhaseACrntSnsrFltEDriveMfile_20230607", "PhaseBCrntSnsrFltEDriveMfile_20230607", "PhaseCCrntSnsrFltEDriveMfile_20230607", "PowerEDriveMfile_20230607", "SW_EditionEDriveMfile_20230607", "StateEDriveMfile_20230607", "TrqRefFnlEDriveMfile_20230607", "Ud_RefEDriveMfile_20230607", "Uq_RefEDriveMfile_20230607", "VoltUsageEDriveMfile_20230607", "VoltageHVEDriveMfile_20230607", "War_IgbtTem_UTEDriveMfile_20230607", "War_MtrTem_UTEDriveMfile_20230607", "War_PhaseOverCrntEDriveMfile_20230607", "phaseA_currentEDriveMfile_20230607", "phaseB_currentEDriveMfile_20230607", "phaseC_currentEDriveMfile_20230607"] ("Headers 2")
  (unwired) T3 [{"Item"=enum."P", "Ch(0:Ch1)"=enum."1"}, {"Item"=enum."P", "Ch(0:Ch1)"=enum."2"}, {"Item"=enum."P", "Ch(0:Ch1)"=enum."3"}, {"Item"=enum."P", "Ch(0:Ch1)"=enum."4"}, {"Item"=enum."P", "Ch(0:Ch1)"=enum."123"}] ("Power")
  (unwired) string[] ["Time", "Throttle % ", "Speed Summary", "Torque Summary", "Power", "Gear Ratio", "Engine Speed", "Engine Torque", "L Speed", "R Speed", "H Speed", "L Torque ", "R Torque ", "H Torque ", "Intercooler_In_T", "Intercooler_Out_T", "Exhaust_T", "Oil_T", "Coolant_Inlet_T", "Coolant_Outlet_T", "Basement_T", "T Spare 1", "T Spare 2", "T Spare 3", "T Spare 4", "T Spare 5", "T Spare 6", "T Spare 7", "T Spare 8", "Coolant-In_P", "Coolant-Out_P", "Exhaust_P", "Oil_P", "Intercooler-In_P", "Intercooler-Out_P", "Misc_P ", "P Spare 1", "P Spare 2", "P Spare 3", "P Spare 4", "Engine RPM "] ("Column Header 2")
  # "P Spare 1"
  # "200\n120\n20\n95\n2000\n850\n100\n2000"
  n1 = flat-sequence {
    tunnel: [w81] -> w2
    tunnel: errorcluster {"status"=FALSE, "code"=0, "source"=""} ("error constant") -> [w81]
    frame #0 {
      w82 = FALSE ("Stop")
      n2 = local write "Stop All"(w82) -> ()
      n3 = local write "Stop"(w82) -> ()
      n4 = Wait (ms)(milliseconds to wait=u32 1000) -> ()  [unwired: 1 out]
    }
  }
  n5 = xnode "Open FPGA VI Reference"("error in"=w2, "resource name"=tag "rio://192.168.17.44/RIO1") -> ("FPGA VI Reference Out"=w47:refnum<k20>, "error out"=w44:errorcluster)
  n6 = xnode "Invoke Method"("FPGA VI Reference In"=w47, "error in"=w44) -> ("FPGA VI Reference Out"=w46:refnum<k20>, "error out"=w4:errorcluster)
  n7 = xnode "Read/Write Control"("FPGA VI Reference In"=w46, "Loop Rate (uS)"=u32 0) -> ("FPGA VI Reference Out"=w29:refnum<k20>)  [unwired: 1 in, 1 out]
  n8 = call <vilib>:"Application Directory.vi"() -> ("Application Directory"=w23:path)
  n9 = Build Path(base path=w23, name or relative path="Data\\Power Analyser.txt") -> (appended path=w22:path)
  n10 = xnode "Invoke Method"("FPGA VI Reference In"=w29, "error in"=w4, "Wait Until Done (F)"=FALSE) -> ("FPGA VI Reference Out"=w40:refnum<k20>, "error out"=w39:errorcluster)
  n11 = call-poly <vilib>:"Read Delimited Spreadsheet.vi"("file path (dialog if empty)"=w22, "error in (no error)"=w2, "delimiter (\\t)"="," ("delimiter (\\t)")) -> ("first row"=w20:string[], "error out"=w18:errorcluster)  [unwired: 7 in, 4 out]
  n12 = Index Array(array=w20, index=1) -> (element=w59:string)
  n13 = xnode "Invoke Method"("FPGA VI Reference In"=w40, "error in"=w39, "Requested Depth"=u32 1000) -> ("FPGA VI Reference Out"=w35:refnum<k20>, "error out"=w34:errorcluster)  [unwired: 1 out]
  n14 = xnode "Invoke Method"("FPGA VI Reference In"=w40, "error in"=w39, "Requested Depth"=u32 4000) -> ("FPGA VI Reference Out"=w51:refnum<k20>, "error out"=w50:errorcluster)  [unwired: 1 out]
  n15 = call <vilib>:"Clear Errors.vi"("error in (no error)"=w18) -> ("error out"=w10:errorcluster)  [unwired: 5 in, 1 out]
  n16 = Equal?(x=w59, y="1") -> (x = y?=w56:bool)
  n17 = call "READ DUBAS DATA.vi"("STATES"=DUBAS_FGV_STATES."OPEN REF", "error in (no error)"=w10) -> ("error out"=w9:errorcluster)  [unwired: 8 in, 1 out]
  n18 = call "Power Analyser FGV Enable.vi"("Enum"=Power_Analyser_Enum."WRITE", "Enable"=w56) -> ()  [unwired: 9 in, 1 out]
  n19 = call <vilib>:"Clear Errors.vi"("error in (no error)"=w9) -> ("error out"=w8:errorcluster)  [unwired: 5 in, 1 out]
  n20 = xnode "Invoke Method"("FPGA VI Reference In"=w35, "error in"=w34) -> ("FPGA VI Reference Out"=w36:refnum<k20>, "error out"=w37:errorcluster)
  n21 = xnode "Invoke Method"("FPGA VI Reference In"=w51, "error in"=w50) -> ("FPGA VI Reference Out"=w49:refnum<k20>, "error out"=w48:errorcluster)
  n22 = Obtain Queue(element data type=sgl[] [], error in (no error)=w8) -> (queue out=w75:refnum<queue>, error out=w3:errorcluster)  [unwired: 3 in, 1 out]
  n23 = call "Get Calibration Table.vi"("error in (no error)"=w3) -> ("error out"=w73:errorcluster, "AI Calibration Table"=w72:string[][])  [unwired: 8 in, 1 out]
  n24 = case shown="True" w56 {
    tunnel: w3 -> [w83 w85]
    tunnel: [w83 w84] -> w65
    frame False {
    }
    frame True {
      n25 = call "FGV_READ.vi"("States"=States."Open Com", "error in"=w85) -> ("error out"=w84:errorcluster)  [unwired: 8 in, 1 out]
    }
  }
  n26 = flat-sequence {
    tunnel: ["Macro: Initialize"] -> w77
    frame #0 {
      n27 = Wait (ms)(milliseconds to wait=u32 1000) -> ()  [unwired: 1 out]
    }
    frame #1 {
    }
  }
  n28 = Obtain Queue(element data type=sgl[] []) -> (queue out=w70:refnum<queue>, error out=w27:errorcluster)  [unwired: 4 in, 1 out]
  n29 = xnode "Invoke Method"("FPGA VI Reference In"=w36, "error in"=w37) -> ("FPGA VI Reference Out"=w32:refnum<k20>, "error out"=w33:errorcluster)
  n30 = xnode "Invoke Method"("FPGA VI Reference In"=w49, "error in"=w48) -> ("FPGA VI Reference Out"=w43:refnum<k20>, "error out"=w42:errorcluster)
  n31 = call <vilib>:"Add State(s) to Queue__JKI_lib_State_Machine.vi"("State(s) in (\"\")"="Macro: Initialize") -> ("States Out"=w6:string)  [unwired: 14 in]
  n32 = call "Get Channel Wise Calibration parameters.vi"("error in (no error)"=w73, "Physical Cgannel"=string[] ["9148Mod1/CH0", "9148Mod1/CH1", "9148Mod1/CH2", "9148Mod1/CH3", "9148Mod2/AI0", "9148Mod2/AI1", "9148Mod2/AI2", "9148Mod2/AI3", "9148Mod2/AI4", "9148Mod2/AI5", "9148Mod2/AI6", "9148Mod2/AI7", "9148Mod2/AI8", "9148Mod2/AI9", "9148Mod2/AI10", "9148Mod2/AI1", "9148Mod2/AI12", "9148Mod2/AI13", "9148Mod2/AI14", "9148Mod2/AI15", "9148Mod4/AI0", "9148Mod4/AI1", "9148Mod4/AI2", "9148Mod4/AI3", "9148Mod4/AI4", "9148Mod4/AI5", "9148Mod4/AI6", "9148Mod4/AI7", "9148Mod4/AI8", "9148Mod4/AI9", "9148Mod4/AI10", "9148Mod4/AI11", "9148Mod4/AI12", "9148Mod4/AI13", "9148Mod4/AI14", "9148Mod4/AI15", "9148Mod3/AI0", "9148Mod3/AI1", "9148Mod3/AI2", "9148Mod3/AI3", "9148Mod3/AI4", "9148Mod3/AI5", "9148Mod3/AI6", "9148Mod3/AI7", "9148Mod3/AI8", "9148Mod3/AI9", "9148Mod3/AI10", "9148Mod3/AI11", "9148Mod3/AI12", "9148Mod3/AI13", "9148Mod3/AI14", "9148Mod3/AI15"] ("Array"), "Calibration Table"=w72) -> ("error out"=w71:errorcluster, "Slop & Offset"=w74:sgl[][])  [unwired: 6 in, 1 out]
  n33 = call <vilib>:"Clear Errors.vi"("error in (no error)"=w65) -> ("error out"=w1:errorcluster)  [unwired: 5 in, 1 out]
  n34 = call "Get Channel Wise Calibration parameters.vi"("error in (no error)"=w71, "Physical Cgannel"=string[] ["9148Mod7/TC0", "9148Mod7/TC1", "9148Mod7/TC2", "9148Mod7/TC3", "9148Mod7/TC4", "9148Mod7/TC5", "9148Mod7/TC6", "9148Mod7/TC7", "9148Mod7/TC8", "9148Mod7/TC9", "9148Mod7/TC10", "9148Mod7/TC11", "9148Mod7/TC12", "9148Mod7/TC13", "9148Mod7/TC14", "9148Mod7/TC15", "9148Mod8/TC0", "9148Mod8/TC1", "9148Mod8/TC2", "9148Mod8/TC3", "9148Mod8/TC4", "9148Mod8/TC5", "9148Mod8/TC6", "9148Mod8/TC7", "9148Mod8/TC8", "9148Mod8/TC9", "9148Mod8/TC10", "9148Mod8/TC11", "9148Mod8/TC12", "9148Mod8/TC13", "9148Mod8/TC14", "9148Mod8/TC15"] ("Array"), "Calibration Table"=w72) -> ("error out"=w17:errorcluster, "Slop & Offset"=w16:sgl[][])  [unwired: 6 in, 1 out]
  n35 = while "JKI State Machine 2018" {
    shift-right: [w92] -> _
    shift-left: _ -> [w91]
    shift-right: [w95] -> _
    shift-left: errorcluster {"status"=FALSE, "code"=0, "source"=""} ("error IO") -> [w89]
    shift-right: [w94] -> _
    shift-left: w6 -> [w96]
    stop <- w93 stop-if-true
    w90 = 100  # Timeout
    # "Limit Checker"
    n36 = call <vilib>:"Parse State Queue__JKI_lib_State_Machine.vi"("State Queue"=w96, "Error In (no error)"=w89) -> ("Remaining States"=w98:string, "Current State"=w99:string, "Arguments"=w97:string)  [unwired: 11 in]
    n37 = case shown="\"Calculated Limit\"" w99 {
      selector: w99 -> [_ _ w152 _ _ _ _ _ _ _ _ _ _ _ _ _ _ _ _ _ _ _ _ _ _ _ _ _ _ _ _]
      tunnel: w98 -> [w107 w150 w156 w175 w182 w189 w194 w241 w250 w261 w266 w272 w279 w292 w362 w416 w457 w462 w485 w499 w515 w531 w557 w598 w624 w678 w692 w703 w714 w717 w725]
      tunnel: w97 -> [_ _ _ _ _ _ _ _ _ _ _ _ w274 w286 _ _ _ _ _ _ _ _ _ _ _ _ _ _ _ _ _]
      tunnel: w91 -> [w105 w147 w154 w168 w179 w187 w191 _ w249 w255 w263 w270 w277 w288 w359 w414 w454 w459 w478 w497 w513 w529 w536 w601 w621 w669 w683 w696 w707 w718 w724]
      tunnel: [w104 w148 w158 w172 errorcluster {"status"=FALSE, "code"=0, "source"=""} ("error out") w184 w192 w236 w245 w251 w264 w269 w275 w284 w360 w381 w455 w460 w483 w488 w505 w517 w538 w599 w613 w675 w689 w700 w711 w716 w720] -> w95
      tunnel: w89 -> [w103 w148 w157 w172 w178 w185 w192 w237 w244 w259 w264 w269 w276 w290 w360 w373 w455 w460 w483 w492 w507 w523 w568 w600 w613 w676 w690 w701 w712 w716 w721]
      tunnel: [w106 w149 w155 w174 w181 w188 w193 w240 w250 w260 w265 w271 w278 w291 w361 w415 w456 w461 w484 w498 w514 w530 w557 w597 w624 w678 w692 w703 w714 w717 w725] -> w94
      tunnel: [FALSE FALSE FALSE _ FALSE TRUE FALSE FALSE FALSE FALSE FALSE FALSE FALSE FALSE FALSE FALSE FALSE FALSE FALSE FALSE FALSE FALSE FALSE FALSE FALSE _ FALSE FALSE FALSE FALSE FALSE] -> w93
      tunnel: [w102 w147 w154 w173 w179 w187 w191 w239 w248 w253 w263 w270 w277 w288 w359 w414 w454 w459 w477 w496 w512 w528 w534 w601 w619 w666 w680 w694 w705 w718 w722] -> w92
      tunnel: w90 -> [w101 _ _ _ _ _ _ _ _ _ _ _ _ _ _ _ _ _ _ _ _ _ _ _ _ _ _ _ _ _ _]
      frame "", "Event Structure", "Idle" {
        n38 = event shown="[0] Timeout" {
          selector: _ -> [_ _ _ _]
          dyn-events: _ -> [_ _ _ _]
          timeout: w101 -> [_ _ _ _]
          tunnel: w107 -> [w128 w131 w139 w140]
          tunnel: [w127 w130 w138 w140] -> w106
          tunnel: w105 -> [w114 w132 w136 w141]
          tunnel: [w123 w133 w137 w142] -> w104
          tunnel: w103 -> [w124 w133 w137 w143]
          tunnel: [w112 w132 w136 w141] -> w102
          event Timeout {
            n39 = event-data() -> ()  [unwired: 1 in, 1 out]
            n40 = Unbundle By Name(w114) -> ("Reset"=w121:bool)
            n41 = local read "Stop"() -> (w111:bool)
            n42 = call "Application Stop.vi"("Command"=enum16{"Read ", "Write "}."Read ") -> ("STOP"=w109:bool)  [unwired: 9 in, 1 out]
            n43 = Or(x=w111, y=w109) -> (x .or. y?=w110:bool)
            n44 = call "Timer.vi"("error in (no error)"=w124, "Reset"=w121, "Target Time"=300.0) -> ("error out"=w123:errorcluster, "Elapsed?"=w120:bool)  [unwired: 6 in, 1 out]
            n45 = Equal?(x=TRUE, y=w120) -> (x = y?=w118:bool)
            n46 = Select(t="Macro: Exit", s=w110, f="Check Lower Warning\nCheck Higher Warning\nCheck Lower fault\nCheck Higher Fault\nDisplay Warning & Faults\nCalculated Limit" ("State(s) at Back (\"\")")) -> (s? t:f=w117:string)
            n47 = Bundle By Name(cluster=w114, "Reset"=FALSE) -> (w112:T11)
            n48 = Select(t="Check Lower Warning\nCheck Higher Warning\nCheck Lower fault\nCheck Higher Fault\nDisplay Warning & Faults\nCalculated Limit\nTimer Elapese" ("State(s) at Back (\"\")"), s=w118, f=w117) -> (s? t:f=w115:string)
            n49 = call <vilib>:"Add State(s) to Queue__JKI_lib_State_Machine.vi"("State(s) in (\"\")"=w128, "State(s) at Back (\"\")"=w115) -> ("States Out"=w127:string)  [unwired: 13 in]
          }
          event "Safety Limits": Value Change {
            n50 = event-data() -> ()  [unwired: 1 in, 1 out]
            n51 = call <vilib>:"Add State(s) to Queue__JKI_lib_State_Machine.vi"("State(s) in (\"\")"=w131, "State(s) at Back (\"\")"="Launch Limit Config" ("State(s) at Back (\"\")")) -> ("States Out"=w130:string)  [unwired: 13 in]
          }
          event Panel Close? {
            # "Discard the event because we'll close the front panel ourselves in Macro: Exit"
            # "Close Panel button (pressed) Event\n(this executes Macro: Exit to terminate the VI)"
            n52 = event-data() -> ()  [unwired: 1 in, 1 out]
            n53 = event-data("Discard?"=TRUE) -> ()  [unwired: 1 in, 1 out]
            n54 = call <vilib>:"Add State(s) to Queue__JKI_lib_State_Machine.vi"("State(s) in Front (\"\")"="Macro: Exit", "State(s) in (\"\")"=w139) -> ("States Out"=w138:string)  [unwired: 13 in]
          }
          event "Gear Ratio": Value Change {
            n55 = event-data() -> ()  [unwired: 1 in, 1 out]
            n56 = local read "Gear Ratio"() -> (w144:dbl)
            n57 = call "Gare ratio save FGV.vi"("Command"=T6."Write Data", "error in (no error)"=w143, "Gear Ratio"=w144) -> ("error out"=w142:errorcluster)  [unwired: 7 in, 1 out]
          }
        }
      }
      frame "---------- Core ----------" {
        # "Do not put any code in this frame.\n(it is a separator no-op)"
        n58 = call <vilib>:"Add State(s) to Queue__JKI_lib_State_Machine.vi"("State(s) in (\"\")"=w150) -> ("States Out"=w149:string)  [unwired: 14 in]
      }
      frame Default {
        w161 = 42 items=["No error", "Argument error", "Memory is full", "Out of zone", "End of file", "File already open", "Generic file I/O error", "File not found", "File permission error", "Disk is full", "Duplicate path", "Too many files open", "System feature not enabled", "Resource file not found", "Cannot add resource", "Resource not found", "Image not found", "Image memory error", "Pen does not exist", "Config type invalid", "Config token not found", "Config parse error", "Config memory error", "Bad external code format", "Bad external code offset", "External code not present", "Null window", "Destroy window error", "Null menu", "Print aborted", "Bad print record", "Print driver error", "Windows error during printing", "Memory error during printing", "Print dialog error", "Generic print error", "Invalid device refnum", "Device not found", "Device parameter error", "Device unit error", "Cannot open device", "Device call aborted", "Generic error", "Cancelled by user", "Object ID too low", "Object ID too high", "Object not in heap", "Unknown heap", "Unknown object (invalid DefProc)", "Unknown object (DefProc not in table)", "Message out of range", "Invalid (null) method", "Unknown message", "Manager call not supported", "Bad address", "Network operation in progress", "Network operation timed out", "Connection is busy", "Network attribute not supported", "Network error", "Address in use", "System out of memory", "Connection aborted", "Connection refused", "Not connected", "Already connected", "Connection closed", "Initialization error (interapplication manager)", "Bad occurrence", "Wait on unbound occurrence handler", "Occurrence queue overflow", "Datalog type conflict", "Unused", "Unrecognized type (interapplication manager)", "Memory corrupt", "Failed to make temporary DLL", "Old CIN version", "Drag socket not found", "Failed to load drop-object", "Failed to register OLE object", "Failed to release OLE object", "Format specifier type mismatch", "Unknown format specifier", "Too few format specifiers", "Too many format specifiers", "Scan failed", "Newer CIN version", "Error converting to variant", "Runtime menu error", "Password tampered", "Variant attribute not found", "Incompatible variant data type", "Event data is not available", "Event Store is not present", "Occurrence is not found", "Event Queue is not created", "Event info is not available", "Refnum passed is NULL", "Error retrieving Class GUID", "Error retrieving CoClass GUID", "Error retrieving TypeLib GUID.", "Bad built application magic bytes.", "Specific driver is different from the specific driver associated with the Logical Name.", "There is no session opened to the class driver.", "Max Error", "MAX - Error with config objects", "MAX - Error loading configuration", "MAX - Group not supported"]
        # "Current State"
        # "Do not delete, rename, or modify this frame.\n(this is used to capture unhandled states and typos)"
        # "Handle mistyped state name (developer tool)"
        n59 = Format Into String(format string="Software Exception: Unhandled State \"%s\"." ("message"), error in=w157, w152) -> (resulting string=w160:string, error out=w159:errorcluster)  [unwired: 1 in]
        n60 = call <vilib>:"Error Cluster From Error Code.vi"("show call chain? (False)"=TRUE, "error in (no error)"=w159, "error message (\"\")"=w160, "error code (0)"=w161) -> ("error out"=w158:errorcluster)  [unwired: 5 in]
        n61 = call <vilib>:"Add State(s) to Queue__JKI_lib_State_Machine.vi"("State(s) in (\"\")"=w156) -> ("States Out"=w155:string)  [unwired: 14 in]
      }
      frame "Initialize Core Data" {
        # "Do not delete, rename, or modify this frame.\n(this is used to determine panel behavior on exit)"
        # "originally closed?"
        # "exe?"
        # "If panel starts closed or is an EXE, then close it when we exit"
        n62 = property class="App"() -> ("App.Kind"=w171:T8)  [unwired: 2 in, 2 out]
        n63 = property class="VI"() -> ("FP.State"=w165:T7)  [unwired: 2 in, 2 out]
        n64 = control-ref of="Current VI Reference"() -> (w166:refnum<vi>)
        n65 = Equal?(x=w165, y=T7."Closed" ("Front Panel Window:State")) -> (x = y?=w163:bool)
        n66 = Equal?(x=w171, y=T8."Run Time System" ("Application:Kind")) -> (x = y?=w169:bool)
        n67 = Or(x=w163, y=w169) -> (x .or. y?=w167:bool)
        n68 = Bundle By Name(cluster=w168, "Core.Current VI Reference"=w166, "Core.Close Panel on Exit?"=w167) -> (w173:T11)
        n69 = call <vilib>:"Add State(s) to Queue__JKI_lib_State_Machine.vi"("State(s) in (\"\")"=w175) -> ("States Out"=w174:string)  [unwired: 14 in]
      }
      frame "Error Handler" {
        # "Unhandled Error -- Display it"
        # "Handle any errors here.\nYou can also output any states to clean-up after errors occur"
        # "Clear error"
        n70 = call <vilib>:"General Error Handler.vi"("error in (no error)"=w178) -> ()  [unwired: 10 in, 5 out]
        n71 = call <vilib>:"Add State(s) to Queue__JKI_lib_State_Machine.vi"("State(s) in Front (\"\")"="/* Post Error States", "State(s) in (\"\")"=w182) -> ("States Out"=w181:string)  [unwired: 13 in]
      }
      frame "Exit" {
        # "Do not put any code in this frame.\n(No errors that occur here will be handled.)"
        n72 = call "Gare ratio save FGV.vi"("Command"=T6."Close", "error in (no error)"=w185) -> ("error out"=w184:errorcluster)  [unwired: 8 in, 1 out]
        n73 = call <vilib>:"Add State(s) to Queue__JKI_lib_State_Machine.vi"("State(s) in (\"\")"=w189) -> ("States Out"=w188:string)  [unwired: 14 in]
      }
      frame "---------- Data ----------" {
        # "Do not put any code in this frame.\n(It is a separator no-op. You can make a copy of this frame to create a new Data frame)"
        n74 = call <vilib>:"Add State(s) to Queue__JKI_lib_State_Machine.vi"("State(s) in (\"\")"=w194) -> ("States Out"=w193:string)  [unwired: 14 in]
      }
      frame "Data: Initialize" {
        w195 = TRUE  # Reset
        w212 = ":\\Safty Alarms warning\\%Y\\%m\\%d"  # :\Safty Alarms warning\%Y\%m\%d
        w216 = string[] []  # Calculated HF
        w215 = string[] []  # Calculated GEN HF Events
        w218 = string[] []  # Calculated LF
        w217 = string[] []  # Calculated GEN LF Events
        w219 = string[] []  # Calculated HW
        w220 = string[] []  # Calculated LW
        w221 = sgl[] []  # Calculated value
        w223 = dbl[] []  # Cal Limit Input
        w224 = T9[] [{"1LF"=1.0, "1HW select"=TRUE, "1LW select"=TRUE, "1LF select"=FALSE, "1HW"=0.0, "1LW"=0.0, "1HF"=0.0, "1HF select"=TRUE, "CH1"="Power LR", "1_LF_EVENT"="Idle", "1_HF_EVENT"="Idle"}, {"1LF"=1.0, "1HW select"=TRUE, "1LW select"=TRUE, "1LF select"=FALSE, "1HW"=0.0, "1LW"=0.0, "1HF"=0.0, "1HF select"=TRUE, "CH1"="Power H", "1_LF_EVENT"="Idle", "1_HF_EVENT"="Idle"}]  # Cal Limits
        w225 = T12 []  # AILimitConfig
        w226 = string[] []  # GenHF
        w227 = string[] []  # GenLF
        w228 = sgl[] []  # Input Values
        w230 = string[] []  # Higher Warning
        w229 = string[] []  # Higher Fault
        w231 = string[] []  # Lower Fault
        w232 = string[] []  # Lower Warning
        w233 = string[] []  # HF Actions
        w234 = string[] []  # Channel Name
        w238 = T13 {"Current VI Reference"=refnum, "Close Panel on Exit?"=FALSE}  # Core
        n75 = call "Get IO Config Path.vi"("error in (no error)"=w237) -> ("error out"=w236:errorcluster, "Limit Path"=w235:T10)  [unwired: 5 in, 4 out]
        n76 = Concatenate Strings("D", w212) -> (w211:string)
        n77 = Format Date/Time String(time format string (%c)="%I %M %S") -> (date/time string=w204:string)  [unwired: 2 in]
        n78 = Format Date/Time String(time format string (%c)=w211) -> (date/time string=w210:string)  [unwired: 2 in]
        n79 = String To Path(string=w210) -> (path=w207:path)
        n80 = Concatenate Strings(w204, ".csv" ("string")) -> (w208:string)
        n81 = call "Create Directory Structure.vi"("Dir Path In"=w207) -> ("Dir Path Out"=w206:path)  [unwired: 3 in, 1 out]
        n82 = Build Path(base path=w206, name or relative path=w208) -> (appended path=w203:path)
        n83 = call <vilib>:"Application Directory.vi"() -> ("Application Directory"=w201:path)
        n84 = Build Path(base path=w201, name or relative path="Data\\gare ratio.txt") -> (appended path=w199:path)
        n85 = call "Gare ratio save FGV.vi"("Command"=T6."Initialise", "File Path"=w199) -> ("error out"=w196:errorcluster)  [unwired: 8 in, 1 out]
        n86 = call "Gare ratio save FGV.vi"("Command"=T6."Read Data", "error in (no error)"=w196) -> ("Gear Ratio"=w200:dbl)  [unwired: 8 in, 1 out]
        n87 = local write "Gear Ratio"(w200) -> ()
        n88 = Bundle("appended path"=w203, "Core"=w238, "AILimitConfig"=w225, "GenHF"=w226, "GenLF"=w227, "Cal Limits"=w224, "Cal Limit Input"=w223, "Channel Name"=w234, "HF Actions"=w233, "Lower Warning"=w232, "Lower Fault"=w231, "Higher Warning"=w230, "Higher Fault"=w229, "Input Values"=w228, "Limit Path"=w235, "Calculated value"=w221, "Calculated LW"=w220, "Calculated HW"=w219, "Calculated LF"=w218, "Calculated GEN LF Events"=w217, "Calculated HF"=w216, "Calculated GEN HF Events"=w215, "Reset"=w195) -> (w239:T11)  [unwired: 1 in]
        n89 = call <vilib>:"Add State(s) to Queue__JKI_lib_State_Machine.vi"("State(s) in (\"\")"=w241, "State(s) at Back (\"\")"="Get Limits\nCheck Lower Warning\nCheck Higher Warning\nCheck Lower fault\nCheck Higher Fault\nCalculated Limit\nDisplay Warning & Faults" ("State(s) at Back (\"\")")) -> ("States Out"=w240:string)  [unwired: 13 in]
      }
      frame "Get Limits" {
        n90 = call "Get AI Limit Configuration.vi"("error in (no error)"=w244) -> ("error out"=w243:errorcluster, "AI LIMIT out"=w247:T12)  [unwired: 9 in]
        n91 = call "Read Calculated limit Config.vi"("error in (no error)"=w243) -> ("error out"=w245:errorcluster, "Cal Limits"=w246:T9[])  [unwired: 9 in]
        n92 = Bundle By Name(cluster=w249, "AILimitConfig"=w247, "Cal Limits"=w246) -> (w248:T11)
      }
      frame "Data: Cleanup" {
        n93 = Unbundle By Name(w255) -> ("Core.Current VI Reference"=w257:refnum<vi>)
        n94 = Close Reference(reference=w257, error in (no error)=w259) -> (error out=w258:errorcluster)
        n95 = invoke class="VI" method="FP.Close"(reference=w257, error in=w258) -> (error out=w252:errorcluster)  [unwired: 1 in, 2 out]
        n96 = call <vilib>:"Clear Errors.vi"("error in (no error)"=w252) -> ("error out"=w251:errorcluster)  [unwired: 5 in, 1 out]
        n97 = Bundle By Name(cluster=w255, "appended path"=path "") -> (w253:T11)
        n98 = call <vilib>:"Add State(s) to Queue__JKI_lib_State_Machine.vi"("State(s) in (\"\")"=w261) -> ("States Out"=w260:string)  [unwired: 14 in]
      }
      frame "---------- UI ----------" {
        # "Do not put any code in this frame.\n(It is a separator no-op. You can make a copy of this frame to create a new UI frame)"
        n99 = call <vilib>:"Add State(s) to Queue__JKI_lib_State_Machine.vi"("State(s) in (\"\")"=w266) -> ("States Out"=w265:string)  [unwired: 14 in]
      }
      frame "UI: Initialize" {
        # "Initialize the User Interface, here.\n(this is called automatically, by the Macro: Init)"
        n100 = property on="Alarms & warning" class="CmbBox"("Strings[]"=string[] [] ("Strings []")) -> ()  [unwired: 2 in, 2 out]
        n101 = call <vilib>:"Add State(s) to Queue__JKI_lib_State_Machine.vi"("State(s) in (\"\")"=w272) -> ("States Out"=w271:string)  [unwired: 14 in]
      }
      frame "UI: Cursor Set" {
        # "Argument"
        # "Set and Unset Cursor Busy.\n(Usage: \"UI: Cursor Set >> Busy|Idle\")"
        n102 = case shown="\"Idle\", Default" w274 {
          tunnel: w276 -> [w281 w283]
          tunnel: [w280 w282] -> w275
          frame "Idle", Default {
            n103 = call <vilib>:"Unset Busy.vi"("error in (no error)"=w281) -> ("error out"=w280:errorcluster)  [unwired: 10 in]
          }
          frame "Busy" {
            n104 = call <vilib>:"Set Busy.vi"("error in (no error)"=w283) -> ("error out"=w282:errorcluster)  [unwired: 9 in, 1 out]
          }
        }
        n105 = call <vilib>:"Add State(s) to Queue__JKI_lib_State_Machine.vi"("State(s) in (\"\")"=w279) -> ("States Out"=w278:string)  [unwired: 14 in]
      }
      frame "UI: Front Panel State" {
        # "Argument"
        # "Set Front Panel Open or Closed\n(Usage: \"UI: Front Panel State >> Open|Close\")"
        n106 = Unbundle By Name(w288) -> ("Core.Current VI Reference"=w287:refnum<vi>)
        n107 = case shown="\"Close\", \"Closed\"" w286 {
          tunnel: w290 -> [w298 w313 w324 w337 w350]
          tunnel: [w300 w314 w326 w339 w352] -> w289
          tunnel: w287 -> [w299 w311 w325 w338 w351]
          frame "Open", "Standard", Default {
            w293 = T7."Standard" ("State")
            n108 = property class="VI"(reference=w299, error in=w298) -> (reference out=w296:refnum<vi>, error out=w297:errorcluster, "FP.State"=w295:T7)
            n109 = Not Equal?(x=w295, y=w293) -> (x != y?=w294:bool)
            n110 = case shown="True" w294 {
              tunnel: [w304 w306] -> w300
              tunnel: w297 -> [w303 w306]
              tunnel: w296 -> [w302 _]
              tunnel: w293 -> [w301 _]
              frame True {
                n111 = invoke class="VI" method="FP.Open"(reference=w302, error in=w303, "Activate"=TRUE, "State"=w301) -> (error out=w304:errorcluster)  [unwired: 1 in, 4 out]
              }
              frame False {
              }
            }
          }
          frame "Close", "Closed" {
            n112 = property class="VI"(reference=w311, error in=w313) -> (reference out=w310:refnum<vi>, error out=w312:errorcluster, "FP.State"=w308:T7)
            n113 = Not Equal?(x=w308, y=T7."Closed" ("Front Panel Window:State")) -> (x != y?=w307:bool)
            n114 = case shown="True" w307 {
              tunnel: [w315 w318] -> w314
              tunnel: w312 -> [w315 w317]
              tunnel: w310 -> [_ w316]
              frame False {
              }
              frame True {
                n115 = invoke class="VI" method="FP.Close"(reference=w316, error in=w317) -> (error out=w318:errorcluster)  [unwired: 1 in, 2 out]
              }
            }
          }
          frame "Hidden", "Hide" {
            w319 = T7."Hidden" ("State")
            n116 = property class="VI"(reference=w325, error in=w324) -> (reference out=w322:refnum<vi>, error out=w323:errorcluster, "FP.State"=w321:T7)
            n117 = Not Equal?(x=w321, y=w319) -> (x != y?=w320:bool)
            n118 = case shown="True" w320 {
              tunnel: [w330 w331] -> w326
              tunnel: w323 -> [w329 w331]
              tunnel: w322 -> [w328 _]
              tunnel: w319 -> [w327 _]
              frame True {
                n119 = invoke class="VI" method="FP.Open"(reference=w328, error in=w329, "State"=w327) -> (error out=w330:errorcluster)  [unwired: 2 in, 4 out]
              }
              frame False {
              }
            }
          }
          frame "Minimize", "Minimized" {
            w332 = T7."Minimized" ("State")
            n120 = property class="VI"(reference=w338, error in=w337) -> (reference out=w335:refnum<vi>, error out=w336:errorcluster, "FP.State"=w334:T7)
            n121 = Not Equal?(x=w334, y=w332) -> (x != y?=w333:bool)
            n122 = case shown="True" w333 {
              tunnel: [w343 w344] -> w339
              tunnel: w336 -> [w342 w344]
              tunnel: w335 -> [w341 _]
              tunnel: w332 -> [w340 _]
              frame True {
                n123 = invoke class="VI" method="FP.Open"(reference=w341, error in=w342, "State"=w340) -> (error out=w343:errorcluster)  [unwired: 2 in, 4 out]
              }
              frame False {
              }
            }
          }
          frame "Maximize", "Maximized" {
            w345 = T7."Maximized" ("State")
            n124 = property class="VI"(reference=w351, error in=w350) -> (reference out=w348:refnum<vi>, error out=w349:errorcluster, "FP.State"=w347:T7)
            n125 = Not Equal?(x=w347, y=w345) -> (x != y?=w346:bool)
            n126 = case shown="True" w346 {
              tunnel: [w356 w357] -> w352
              tunnel: w349 -> [w355 w357]
              tunnel: w348 -> [w354 _]
              tunnel: w345 -> [w353 _]
              frame True {
                n127 = invoke class="VI" method="FP.Open"(reference=w354, error in=w355, "State"=w353) -> (error out=w356:errorcluster)  [unwired: 2 in, 4 out]
              }
              frame False {
              }
            }
          }
        }
        n128 = call <vilib>:"Clear Errors.vi"("error in (no error)"=w289) -> ("error out"=w284:errorcluster)  [unwired: 5 in, 1 out]
        n129 = call <vilib>:"Add State(s) to Queue__JKI_lib_State_Machine.vi"("State(s) in (\"\")"=w292) -> ("States Out"=w291:string)  [unwired: 14 in]
      }
      frame "---------- Macro ----------" {
        # "Do not put any code in this frame.\n(It is a separator no-op. You can make a copy of this frame to create a new Macro frame)"
        n130 = call <vilib>:"Add State(s) to Queue__JKI_lib_State_Machine.vi"("State(s) in (\"\")"=w362) -> ("States Out"=w361:string)  [unwired: 14 in]
      }
      frame "Macro: Initialize" {
        w400 = 16 ("length")
        w399 = 0 ("index")
        w413 = "Data: Initialize\nInitialize Core Data\nUI: Initialize\nUI: Front Panel State >> Open"  # Data: Initialize Initialize Core Data UI: Initialize UI: Front Panel State >> Open
        n131 = call <vilib>:"Application Directory.vi"() -> ("Application Directory"=w377:path)
        n132 = Build Path(base path=w377, name or relative path="Data") -> (appended path=w375:path)
        n133 = Build Path(base path=w375, name or relative path="AI Config.xml") -> (appended path=w374:path)
        n134 = call-poly <vilib>:"Read From XML File.vi"("error in (no error)"=w373, "XML File Path"=w374) -> ("error out"=w410:errorcluster, "XML Elements"=w411:string)  [unwired: 7 in, 1 out]
        n135 = Unflatten From XML(xml string=w411, type=string[][] [], error in (no error)=w410) -> (value=w408:string[][], error out=w383:errorcluster)
        n136 = for {
          tunnel: w408 -> [w445] mode=indexing
          tunnel: [w444] -> w404 mode=indexing
          n137 = Index Array(array=w445, index=2) -> (element=w444:string)
        }
        "Array" <- w404
        n138 = Delete From Array(array=w404, length=4, index=w399) -> (deleted portion=→"Universal AI":string[], array with subset deleted=w406:string[])
        n139 = Delete From Array(array=w406, length=w400, index=w399) -> (deleted portion=w372:string[], array with subset deleted=w405:string[])
        n140 = Delete From Array(array=w405, length=w400, index=w399) -> (deleted portion=w370:string[], array with subset deleted=w402:string[])
        n141 = for {
          tunnel: w370 -> [w427] mode=indexing
          tunnel: [w426] -> w369 mode=indexing
          n142 = Bundle By Name(cluster=cluster{"String":string, "Scalar":sgl} {"String"="P_Oil Gallery", "Scalar"=-107.2287} ("Cluster 3"), "String"=w427) -> (w426:cluster{"String":string, "Scalar":sgl})
        }
        "9208 AI Current" <- w369
        n143 = Delete From Array(array=w402, length=w400, index=w399) -> (deleted portion=w368:string[], array with subset deleted=w401:string[])
        n144 = control-ref of="Coolant-Out_P"() -> (w384:refnum<vi>)
        n145 = control-ref of="Coolant-In_P"() -> (w385:refnum<vi>)
        n146 = control-ref of="Exhaust_P"() -> (w386:refnum<vi>)
        n147 = control-ref of="Oil_P"() -> (w387:refnum<vi>)
        n148 = control-ref of="Intercooler-In_P"() -> (w388:refnum<vi>)
        n149 = control-ref of="Intercooler-Out_P"() -> (w389:refnum<vi>)
        n150 = control-ref of="Misc_P"() -> (w390:refnum<vi>)
        n151 = for {
          tunnel: w372 -> [w430] mode=indexing
          tunnel: [w429] -> w371 mode=indexing
          n152 = Bundle By Name(cluster=cluster{"String":string, "Scalar":sgl} {"String"="P_Oil Gallery", "Scalar"=-107.2287} ("Cluster 3"), "String"=w430) -> (w429:cluster{"String":string, "Scalar":sgl})
        }
        "9220 AI  Volt  Pressure" <- w371
        n153 = Delete From Array(array=w401, length=w400, index=w399) -> (deleted portion=w366:string[], array with subset deleted=w398:string[])
        n154 = Delete From Array(array=w398, length=w400, index=w399) -> (array with subset deleted=w364:string[])  [unwired: 1 out]
        n155 = for {
          tunnel: w364 -> [w418] mode=indexing
          tunnel: [w417] -> w363 mode=indexing
          n156 = Bundle By Name(cluster=cluster{"String":string, "Scalar":sgl} {"String"="P_Oil Gallery", "Scalar"=-107.2287} ("Cluster 3"), "String"=w418) -> (w417:cluster{"String":string, "Scalar":sgl})
        }
        "Thermocouple Spare" <- w363
        n157 = Build Array(w384, w385, w386, w387, w388, w389, w390) -> (w380:refnum<vi>[])
        n158 = for {
          tunnel: w368 -> [w424] mode=indexing
          tunnel: [w423] -> w367 mode=indexing
          n159 = Bundle By Name(cluster=cluster{"String":string, "Scalar":sgl} {"String"="P_Oil Gallery", "Scalar"=-107.2287} ("Cluster 3"), "String"=w424) -> (w423:cluster{"String":string, "Scalar":sgl})
        }
        "9220 AI Volt Spare" <- w367
        n160 = for {
          tunnel: w366 -> [w421] mode=indexing
          tunnel: [w420] -> w365 mode=indexing
          n161 = Bundle By Name(cluster=cluster{"String":string, "Scalar":sgl} {"String"="P_Oil Gallery", "Scalar"=-107.2287} ("Cluster 3"), "String"=w421) -> (w420:cluster{"String":string, "Scalar":sgl})
        }
        "Thermocouple" <- w365
        n162 = for {
          tunnel: w380 -> [w441] mode=indexing
          tunnel: w372 -> [w440] mode=indexing
          tunnel: w383 -> [w439]
          tunnel: [w438] -> w382
          n163 = property class="Slide (strict)"(reference=w441, error in=w439, "Caption.Text"=w440, "Caption.Visible"=TRUE, "Label.Visible"=FALSE) -> (error out=w438:errorcluster)  [unwired: 1 out]
        }
        n164 = control-ref of="Intercooler_In_T"() -> (w391:refnum<vi>)
        n165 = control-ref of="Intercooler_Out_T"() -> (w392:refnum<vi>)
        n166 = control-ref of="Exhaust_T"() -> (w393:refnum<vi>)
        n167 = control-ref of="Oil_T"() -> (w394:refnum<vi>)
        n168 = control-ref of="Coolant_Inlet_T"() -> (w395:refnum<vi>)
        n169 = control-ref of="Coolant_Outlet_T"() -> (w396:refnum<vi>)
        n170 = control-ref of="Basement_T"() -> (w397:refnum<vi>)
        n171 = Build Array(w391, w392, w393, w394, w395, w396, w397) -> (w379:refnum<vi>[])
        n172 = for {
          tunnel: w379 -> [w435] mode=indexing
          tunnel: w366 -> [w434] mode=indexing
          tunnel: w382 -> [w432]
          tunnel: [w433] -> w381
          n173 = property class="Slide (strict)"(reference=w435, error in=w432, "Caption.Text"=w434, "Caption.Visible"=TRUE, "Label.Visible"=FALSE) -> (error out=w433:errorcluster)  [unwired: 1 out]
        }
        n174 = call <vilib>:"Add State(s) to Queue__JKI_lib_State_Machine.vi"("State(s) in Front (\"\")"=w413, "State(s) in (\"\")"=w416) -> ("States Out"=w415:string)  [unwired: 13 in]
      }
      frame "Macro: Exit" {
        # "Exit Macro\n(This is called once, when the VI exits)"
        n175 = Unbundle By Name(w454) -> ("Core.Close Panel on Exit?"=w453:bool)
        n176 = Select(t="UI: Front Panel State >> Close", s=w453, f="") -> (s? t:f=w450:string)
        n177 = call <vilib>:"Add State(s) to Queue__JKI_lib_State_Machine.vi"("State(s) in (\"\")"=w450, "State(s) at Back (\"\")"="Data: Cleanup\nExit") -> ("States Out"=w448:string)  [unwired: 13 in]
        n178 = call <vilib>:"Add State(s) to Queue__JKI_lib_State_Machine.vi"("State(s) in Front (\"\")"=w448, "State(s) in (\"\")"=w457) -> ("States Out"=w456:string)  [unwired: 13 in]
      }
      frame "---------- Main ----------" {
        # "Template Separator\n(You can make a copy of, or modify, this frame)"
        n179 = call <vilib>:"Add State(s) to Queue__JKI_lib_State_Machine.vi"("State(s) in (\"\")"=w462) -> ("States Out"=w461:string)  [unwired: 14 in]
      }
      frame "Check Lower Warning" {
        # "Calculated value"
        n180 = Unbundle By Name(w478) -> ("AILimitConfig"=w476:T12, "Cal Limits"=w471:T9[])
        n181 = local read "speed torque power"() -> (w470:dbl[])
        n182 = local read "Mean"() -> (w473:sgl[])
        n183 = local read "Mean tc"() -> (w472:sgl[])
        n184 = Index Array(array=w470) -> (element #1=w469:dbl, element #2=w468:dbl, element #4=w467:dbl, element #5=w466:dbl)  [unwired: 5 in, 1 out]
        n185 = Build Array(w469, w468, w467, w466) -> (w465:dbl[])
        n186 = Array Subset(array=w472, index=0, length=7) -> ()  [unwired: 1 out]
        n187 = Array Subset(array=w473, index=4, length=7) -> ()  [unwired: 1 out]
        n188 = Build Array (concatenate)(w473, w472) -> (w475:sgl[])
        n189 = call "Check Lower Warning.vi"("Input Values"=w475, "AILimitConfig"=w476) -> ("LW Channel"=w474:string[])  [unwired: 8 in, 1 out]
        n190 = call "calculated Lower Warning.vi"("Input Values"=w465, "Cal LimitConfig"=w471) -> ("LW Channel"=w464:string[])  [unwired: 8 in, 1 out]
        n191 = Bundle By Name(cluster=w478, "Lower Warning"=w474, "Input Values"=w475, "Calculated LW"=w464, "Calculated value"=w465) -> (w477:T11)
        n192 = call <vilib>:"Add State(s) to Queue__JKI_lib_State_Machine.vi"("State(s) in (\"\")"=w485) -> ("States Out"=w484:string)  [unwired: 14 in]
      }
      frame "Check Higher Warning" {
        n193 = Unbundle By Name(w497) -> ("AILimitConfig"=w495:T12, "Input Values"=w493:sgl[], "Cal Limits"=w489:T9[], "Calculated value"=w490:sgl[])
        n194 = call "Check Higher Warning.vi"("error in (no error)"=w492, "Input Values"=w493, "AILimitConfig"=w495) -> ("error out"=w491:errorcluster, "HW Channel"=w494:string[])  [unwired: 7 in]
        n195 = call "calculated Higher Warning.vi"("error in (no error)"=w491, "Input Values"=w490, "Calc LimitConfig"=w489) -> ("error out"=w488:errorcluster, "HW Channel"=w487:string[])  [unwired: 7 in]
        n196 = Bundle By Name(cluster=w497, "Higher Warning"=w494, "Calculated HW"=w487) -> (w496:T11)
        n197 = call <vilib>:"Add State(s) to Queue__JKI_lib_State_Machine.vi"("State(s) in (\"\")"=w499) -> ("States Out"=w498:string)  [unwired: 14 in]
      }
      frame "Check Lower fault" {
        n198 = Unbundle By Name(w513) -> ("AILimitConfig"=w511:T12, "Input Values"=w508:sgl[], "Cal Limits"=w503:T9[], "Calculated value"=w504:sgl[])
        n199 = call "Check Lower Fault.vi"("error in (no error)"=w507, "Input Values"=w508, "AILimitConfig"=w511) -> ("error out"=w506:errorcluster, "LF Events"=w509:string[], "LF Channel"=w510:string[])  [unwired: 6 in]
        n200 = call "calculated Lower Fault.vi"("error in (no error)"=w506, "Input Values"=w504, "AILimitConfig"=w503) -> ("error out"=w505:errorcluster, "LF Events"=w501:string[], "LF Channel"=w502:string[])  [unwired: 6 in]
        n201 = Bundle By Name(cluster=w513, "Lower Fault"=w510, "GenLF"=w509, "Calculated LF"=w502, "Calculated GEN LF Events"=w501) -> (w512:T11)
        n202 = call <vilib>:"Add State(s) to Queue__JKI_lib_State_Machine.vi"("State(s) in (\"\")"=w515) -> ("States Out"=w514:string)  [unwired: 14 in]
      }
      frame "Check Higher Fault" {
        n203 = Unbundle By Name(w529) -> ("AILimitConfig"=w526:T12, "Input Values"=w525:sgl[], "Cal Limits"=w521:T9[], "Calculated value"=w520:sgl[])
        n204 = call "Check Higher Fault.vi"("error in (no error)"=w523, "Input Values"=w525, "AILimitConfig"=w526) -> ("error out"=w522:errorcluster, "HF Events"=w524:string[], "HF Channel"=w527:string[])  [unwired: 6 in]
        n205 = call "Calculated Higher Fault.vi"("error in (no error)"=w522, "Input Values"=w520, "Cal LimitConfig"=w521) -> ("error out"=w517:errorcluster, "HF Events"=w518:string[], "HF Channel"=w519:string[])  [unwired: 6 in]
        n206 = Bundle By Name(cluster=w529, "Higher Fault"=w527, "GenHF"=w524, "Calculated HF"=w519, "Calculated GEN HF Events"=w518) -> (w528:T11)
        n207 = call <vilib>:"Add State(s) to Queue__JKI_lib_State_Machine.vi"("State(s) in (\"\")"=w531) -> ("States Out"=w530:string)  [unwired: 14 in]
      }
      frame "Display Warning & Faults" {
        n208 = Unbundle By Name(w536) -> ("Lower Warning"=w570:string[], "Lower Fault"=w567:string[], "Higher Warning"=w569:string[], "Higher Fault"=w566:string[], "Calculated LW"=w543:string[], "Calculated LF"=w542:string[], "Calculated HW"=w541:string[], "Calculated HF"=w540:string[], "GenHF"=w560:string[], "GenLF"=w559:string[], "Calculated GEN HF Events"=w552:string[], "Calculated GEN LF Events"=w551:string[])
        n209 = Build Array (concatenate)(w560, w559, w552, w551) -> (w558:string[])
        n210 = Build Array (concatenate)(w570, w567, w569, w566, w543, w542, w541, w540) -> (w533:string[])
        n211 = for {
          tunnel: string[] ["Fast Stop", "Engine Stop", "Idle", "Warning"] ("1_HF_EVENT") -> [w590] mode=indexing
          tunnel: w558 -> [w592]
          tunnel: [w590] -> w556
          tunnel: [w589] -> w555
          stop <- w589 stop-if-true
          n212 = Search 1D Array(1D array=w592, element=w590) -> (index of element=w591:i32)  [unwired: 1 in]
          n213 = Greater Or Equal To 0?(x=w591) -> (x >= 0?=w589:bool)
        }
        n214 = Empty Array?(array=w566) -> (empty?=w564:bool)
        n215 = Empty Array?(array=w567) -> (empty?=w565:bool)
        n216 = Empty Array?(array=w542) -> (empty?=w550:bool)
        n217 = Empty Array?(array=w540) -> (empty?=w546:bool)
        n218 = Index Array(array=w533) -> (element=w553:string)  [unwired: 1 in]
        n219 = Not(x=w564) -> (.not. x?=w548:bool)
        n220 = Not(x=w550) -> (.not. x?=w547:bool)
        n221 = Not(x=w546) -> (.not. x?=w545:bool)
        n222 = Not(x=w565) -> (.not. x?=w549:bool)
        n223 = Empty Array?(array=w533) -> (empty?=w562:bool)
        n224 = property on="Alarms & warning" class="CmbBox"(error in=w568, "Strings[]"=w533, "Value"=w553) -> (error out=w563:errorcluster)  [unwired: 1 in, 1 out]
        n225 = Compound Arithmetic op=OR(w549, w548, w547, w545) -> (w544:bool)
        "Saftey_Lim_error" <- w544
        n226 = Not(x=w562) -> (.not. x?=w537:bool)
        n227 = Build Array(w544) -> (w532:bool[])
        n228 = global write "Throttle.vi" "dATA_BOOL"(w532) -> ()
        n229 = case shown="False" w555 {
          tunnel: w556 -> [_ w588]
          tunnel: ["No Alarm" ("1_HF_EVENT") w588] -> w554
          frame False {
          }
          frame True {
          }
        }
        n230 = property on="Alarms & warning" class="CmbBox"(error in=w563, "Blinking"=w537) -> (error out=w535:errorcluster)  [unwired: 1 in, 1 out]
        n231 = case shown="True" w537 {
          tunnel: [w573 w582] -> w538
          tunnel: w536 -> [w574 w580]
          tunnel: w535 -> [w573 w583]
          tunnel: [w574 w579] -> w534
          tunnel: w533 -> [_ w576]
          frame False {
          }
          frame True {
            n232 = Unbundle By Name(w580) -> ("appended path"=w586:path)
            n233 = Format Date/Time String(time format string (%c)="%I: %M: %S:") -> (date/time string=w577:string)  [unwired: 2 in]
            n234 = Build Array (concatenate)(w577, w576) -> (w575:string[])
            n235 = call-poly <vilib>:"Write Delimited Spreadsheet.vi"("file path (dialog if empty)"=w586, "1D data"=w575, "append to file? (new file:F)"=TRUE, "error in (no error)"=w583, "delimiter (\\t)"="," ("delimiter (\\t)")) -> ("new file path (Not A Path if cancelled)"=w581:path, "error out"=w582:errorcluster)  [unwired: 9 in]
            n236 = Bundle By Name(cluster=w580, "appended path"=w581) -> (w579:T11)
          }
        }
        n237 = disable-structure shown="Enabled" {
          disable-tunnel: w554 -> [w571 w572]
          frame Disabled {
            n238 = shared-variable "My Computer\\test_1.lvlib\\Alarm Action"(w571) -> ()  [unwired: 1 in, 1 out]
          }
          frame Enabled {
            n239 = global write "Throttle.vi" "Alarm Action"(w572) -> ()
          }
        }
      }
      frame "Launch Limit Config" {
        n240 = call <vilib>:"Clear Errors.vi"("error in (no error)"=w600) -> ("error out"=w596:errorcluster)  [unwired: 5 in, 1 out]
        n241 = call "Limit Config.vi"("error out 2"=w596, "Run AS Subvi"=TRUE) -> ("error out"=w599:errorcluster)  [unwired: 9 in]
        n242 = call <vilib>:"Add State(s) to Queue__JKI_lib_State_Machine.vi"("State(s) in (\"\")"=w598, "State(s) at Back (\"\")"="Get Limits\nCheck Lower Warning\nCheck Higher Warning\nCheck Lower fault\nCheck Higher Fault\nCalculated Limit\nDisplay Warning & Faults" ("State(s) at Back (\"\")")) -> ("States Out"=w597:string)  [unwired: 13 in]
      }
      frame "Calculated Limit" {
        n243 = global read "Throttle.vi" "DAT DOUBLE"() -> (w614:dbl[])
        n244 = shared-variable "My Computer\\test_1.lvlib\\KeyPosition"() -> (w623:T14)  [unwired: 1 in, 1 out]
        n245 = case shown="\"L-R\"" w623 {
          tunnel: [w626 w637 w656 w664] -> w604
          tunnel: [w630 w640 w654 w664] -> w608
          tunnel: [w629 w638 w653 w664] -> w617
          tunnel: w614 -> [w628 w648 w652 _]
          tunnel: [w625 w639 w655 cluster{"Numeric":dbl, "Numeric":dbl} {"Numeric"=0.0, "Numeric"=0.0}] -> w602
          tunnel: [0.0 0.0 w649 w664] -> w622
          frame "H" {
            # "4,2"
            n246 = Index Array(array=w628) -> (element #3=w626:dbl, element #5=w629:dbl)  [unwired: 9 in, 7 out]
            n247 = Absolute Value(x=w626) -> (abs(x)=w635:dbl)
            n248 = Multiply(x=w629, y=w635) -> (x*y=w634:dbl)
            n249 = Bundle("Numeric"=w629, "Numeric"=w626) -> (w625:cluster{"Numeric":dbl, "Numeric":dbl})  [unwired: 1 in]
            n250 = Multiply(x=w634, y=6.283185307179586) -> (x*y=w633:dbl)
            n251 = Divide(x=w633, y=60000.0) -> (x/y=w630:dbl)
          }
          frame "L-R" {
            n252 = Index Array(array=w648, index #1=7 ("index"), index #2=8 ("index")) -> (element #1=w637:dbl, element #2=w638:dbl)
            n253 = Absolute Value(x=w637) -> (abs(x)=w645:dbl)
            n254 = Multiply(x=w638, y=w645) -> (x*y=w644:dbl)
            n255 = Multiply(x=w644, y=6.283185307179586) -> (x*y=w643:dbl)
            n256 = Divide(x=w643, y=60000.0) -> (x/y=w640:dbl)
            n257 = Bundle("Numeric"=w638, "Numeric"=w637) -> (w639:cluster{"Numeric":dbl, "Numeric":dbl})  [unwired: 1 in]
          }
          frame "H-L-R" {
            n258 = Index Array(array=w652, index #1=7 ("index"), index #2=8 ("index"), index #3=2 ("index"), index #4=4 ("index")) -> (element #1=w656:dbl, element #2=w653:dbl, element #4=w649:dbl)  [unwired: 1 in, 2 out]
            n259 = Absolute Value(x=w656) -> (abs(x)=w661:dbl)
            n260 = Multiply(x=w653, y=w661) -> (x*y=w660:dbl)
            n261 = Multiply(x=w660, y=6.283185307179586) -> (x*y=w659:dbl)
            n262 = Bundle("Numeric"=w653, "Numeric"=w656) -> (w655:cluster{"Numeric":dbl, "Numeric":dbl})  [unwired: 1 in]
            n263 = Divide(x=w659, y=60000.0) -> (x/y=w654:dbl)
          }
          frame "System", Default {
            w664 = 0.0
          }
        }
        "Torque Summary" <- w604
        "Power" <- w608
        "Speed Summary" <- w617
        "Speed Torque" <- w602
        "H Speed" <- w622
        n264 = Divide(x=w604, y="Gear Ratio") -> (x/y=w612:dbl)
        n265 = To Long Integer(number=w612) -> (32bit integer=→"Torque":i32)
        n266 = Multiply(x=w617, y="Gear Ratio") -> (x*y=w609:dbl)
        n267 = To Long Integer(number=w609) -> (32bit integer=→"Speed":i32)
        n268 = Number To Fractional String(number=w608, precision (6)="precision") -> (F-format string=→"Power":string)  [unwired: 2 in]
        n269 = Number To Fractional String(number=w604, precision (6)="precision") -> (F-format string=→"Torque":string)  [unwired: 2 in]
        n270 = Build Array(w617, w604, w608, "Gear Ratio", w609, w612) -> (→"speed torque power":dbl[])
        n271 = Build Array(w608, w622) -> (w620:dbl[])
        n272 = Bundle By Name(cluster=w621, "Cal Limit Input"=w620) -> (w619:T11)
      }
      frame "Check Calculated Limits LF" {
        # "Calculated Limits:\nCheck Lower faults"
        n273 = Unbundle By Name(w669) -> ("GenLF"=w671:string[], "Lower Fault"=w673:string[], "Cal Limits"=w677:T9[], "Cal Limit Input"=w674:dbl[])
        n274 = call "Check Lower Fault.vi"("error in (no error)"=w676, "Input Values"=w674, "AILimitConfig"=w677) -> ("error out"=w675:errorcluster, "LF Events"=w670:string[], "LF Channel"=w672:string[])  [unwired: 6 in]
        n275 = Build Array (concatenate)(w671, w670) -> (w668:string[])
        n276 = Build Array (concatenate)(w673, w672) -> (w667:string[])
        n277 = Bundle By Name(cluster=w669, "Lower Fault"=w667, "GenLF"=w668) -> (w666:T11)
      }
      frame "Check Calculated Limits HF" {
        # "Calculated Limits:\nCheck for Higher faults"
        n278 = Unbundle By Name(w683) -> ("GenHF"=w685:string[], "Higher Fault"=w687:string[], "Cal Limits"=w691:T9[], "Cal Limit Input"=w688:dbl[])
        n279 = call "Check Higher Fault.vi"("error in (no error)"=w690, "Input Values"=w688, "AILimitConfig"=w691) -> ("error out"=w689:errorcluster, "HF Events"=w684:string[], "HF Channel"=w686:string[])  [unwired: 6 in]
        n280 = Build Array (concatenate)(w685, w684) -> (w682:string[])
        n281 = Build Array (concatenate)(w687, w686) -> (w681:string[])
        n282 = Bundle By Name(cluster=w683, "Higher Fault"=w681, "GenHF"=w682) -> (w680:T11)
      }
      frame "Check Calculated Limits LW" {
        # "Calculated Limits:\nCheck Lower Warnings"
        n283 = Unbundle By Name(w696) -> ("Lower Warning"=w698:string[], "Cal Limits"=w702:T9[], "Cal Limit Input"=w699:dbl[])
        n284 = call "Check Lower Warning.vi"("error in (no error)"=w701, "Input Values"=w699, "AILimitConfig"=w702) -> ("error out"=w700:errorcluster, "LW Channel"=w697:string[])  [unwired: 7 in]
        n285 = Build Array (concatenate)(w698, w697) -> (w695:string[])
        n286 = Bundle By Name(cluster=w696, "Lower Warning"=w695) -> (w694:T11)
      }
      frame "Check Calculated Limits HW" {
        # "Calculated Limits:\nCheck for Higher Warning"
        n287 = Unbundle By Name(w707) -> ("Higher Warning"=w709:string[], "Cal Limits"=w713:T9[], "Cal Limit Input"=w710:dbl[])
        n288 = call "Check Higher Warning.vi"("error in (no error)"=w712, "Input Values"=w710, "AILimitConfig"=w713) -> ("error out"=w711:errorcluster, "HW Channel"=w708:string[])  [unwired: 7 in]
        n289 = Build Array (concatenate)(w709, w708) -> (w706:string[])
        n290 = Bundle By Name(cluster=w707, "Higher Warning"=w706) -> (w705:T11)
      }
      frame ".............................extra cases......................" {
      }
      frame "Timer Elapese" {
        n291 = flat-sequence {
          tunnel: w721 -> [w727]
          tunnel: [w727] -> w720
          frame #0 {
            n292 = property on="Speed Torque" class="WFChart (strict)"("History Data"=cluster{"Numeric":dbl, "Numeric":dbl}[] []) -> ()  [unwired: 2 in, 2 out]
          }
        }
        n293 = Bundle By Name(cluster=w724, "Reset"=TRUE) -> (w722:T11)
      }
    }
  }
  n294 = while {
    tunnel: w43 -> [w754]
    shift-right: [w752] -> w60
    shift-left: w42 -> [w753]
    shift-right: [w740] -> w61
    shift-left: w75 -> [w743]
    shift-right: [w741] -> w62
    shift-left: w3 -> [w742]
    tunnel: [w739] -> w63
    stop <- w736 stop-if-true
    w729 = u32 52  # No Of Channels
    w746 = u32 1  # Sampling Rate
    # "Data From 1st module of expansion crio"
    # "This counter value should remail\nzero for lossless data transfer"
    n295 = xnode "Invoke Method"("FPGA VI Reference In"=w754, "error in"=w753, "Number of Elements"=u32 0, "Timeout (ms)"=1000) -> ("FPGA VI Reference Out"=w748:refnum<k20>, "error out"=w751:errorcluster, "Elements Remaining"=w730:u32)  [unwired: 1 out]
    n296 = Multiply(x=w746, y=w729) -> (x*y=w745:u32)
    n297 = Wait Until Next ms Multiple(millisecond multiple=u32 100) -> ()  [unwired: 1 out]
    n298 = Quotient & Remainder(x=w730, y=w729) -> (floor(x/y)=w731:u32)  [unwired: 1 out]
    n299 = Greater Or Equal?(x=w730, y=w745) -> (x >= y?=w744:bool)
    n300 = Multiply(x=w729, y=w731) -> (x*y=w728:u32)
    "x*y" <- w728
    n301 = case shown="True" w744 {
      tunnel: w751 -> [w757 w769]
      tunnel: [w757 w768] -> w750
      tunnel: w748 -> [w758 w767]
      tunnel: [w758 w766] -> w747
      tunnel: w728 -> [_ w765]
      tunnel: w743 -> [w755 w764]
      tunnel: w742 -> [w756 w762]
      tunnel: [w756 w761] -> w741
      tunnel: [w755 w760] -> w740
      frame False {
      }
      frame True {
        n302 = xnode "Invoke Method"("FPGA VI Reference In"=w767, "error in"=w769, "Number of Elements"=w765, "Timeout (ms)"=1000) -> ("FPGA VI Reference Out"=w766:refnum<k20>, "error out"=w768:errorcluster, "Data"=w763:sgl[])  [unwired: 1 out]
        n303 = Enqueue Element(queue=w764, element=w763, error in (no error)=w762) -> (queue out=w760:refnum<queue>, error out=w761:errorcluster)  [unwired: 1 in, 1 out]
      }
    }
    n304 = xnode "Read/Write Control"("FPGA VI Reference In"=w747, "error in"=w750) -> ("FPGA VI Reference Out"=w739:refnum<k20>, "error out"=w752:errorcluster, "Timeout Counter"=→"Timeout Counter":u64)
    n305 = local read "Stop All"() -> (w737:bool)
    n306 = call "Application Stop.vi"("Command"=enum16{"Read ", "Write "}."Read ") -> ("STOP"=w735:bool)  [unwired: 9 in, 1 out]
    n307 = Or(x=w735, y=w737) -> (x .or. y?=w736:bool)
  }
  n308 = while {
    tunnel: w32 -> [w793]
    shift-right: [w790] -> _
    shift-left: w33 -> [w792]
    shift-right: [w780] -> w26
    shift-left: w70 -> [w783]
    shift-right: [w781] -> w25
    shift-left: w27 -> [w782]
    tunnel: [w787] -> _
    stop <- w778 stop-if-true
    w771 = u32 32  # No Of Channels
    w786 = u32 1  # Sampling Rate
    # "Data From Thermocouples module of expansion crio"
    n309 = xnode "Invoke Method"("FPGA VI Reference In"=w793, "error in"=w792, "Number of Elements"=u32 0, "Timeout (ms)"=1000) -> ("FPGA VI Reference Out"=w788:refnum<k20>, "error out"=w791:errorcluster, "Elements Remaining"=w773:u32)  [unwired: 1 out]
    n310 = Multiply(x=w786, y=w771) -> (x*y=w785:u32)
    n311 = Wait Until Next ms Multiple(millisecond multiple=u32 100) -> ()  [unwired: 1 out]
    n312 = Quotient & Remainder(x=w773, y=w771) -> (floor(x/y)=w772:u32)  [unwired: 1 out]
    n313 = Greater Or Equal?(x=w773, y=w785) -> (x >= y?=w784:bool)
    n314 = Multiply(x=w771, y=w772) -> (x*y=w770:u32)
    n315 = case shown="True" w784 {
      tunnel: w791 -> [w796 w808]
      tunnel: [w796 w807] -> w790
      tunnel: w788 -> [w797 w806]
      tunnel: [w797 w805] -> w787
      tunnel: w770 -> [_ w804]
      tunnel: w783 -> [w794 w803]
      tunnel: w782 -> [w795 w801]
      tunnel: [w795 w800] -> w781
      tunnel: [w794 w799] -> w780
      tunnel: w773 -> [_ _]
      frame False {
      }
      frame True {
        n316 = xnode "Invoke Method"("FPGA VI Reference In"=w806, "error in"=w808, "Number of Elements"=w804, "Timeout (ms)"=1000) -> ("FPGA VI Reference Out"=w805:refnum<k20>, "error out"=w807:errorcluster, "Data"=w802:sgl[])  [unwired: 1 out]
        n317 = Enqueue Element(queue=w803, element=w802, error in (no error)=w801) -> (queue out=w799:refnum<queue>, error out=w800:errorcluster)  [unwired: 1 in, 1 out]
      }
    }
    n318 = local read "Stop All"() -> (w779:bool)
    n319 = call "Application Stop.vi"("Command"=enum16{"Read ", "Write "}."Read ") -> ("STOP"=w777:bool)  [unwired: 9 in, 1 out]
    n320 = Or(x=w777, y=w779) -> (x .or. y?=w778:bool)
  }
  n321 = while {
    shift-right: [w946] -> _
    shift-left: w75 -> [w936]
    shift-right: [w865] -> w64
    shift-left: w1 -> [w851]
    tunnel: w74 -> [w935]
    stop <- w863 stop-if-true
    w854 = 16 ("length")
    w855 = 0 ("index")
    n322 = Dequeue Element(queue=w936, error in (no error)=w851) -> (queue out=w946:refnum<queue>, element=w877:sgl[], error out=w865:errorcluster)  [unwired: 1 in, 1 out]
    "error out 2" <- w865
    n323 = call "Power Analyser FGV Enable.vi"("Enum"=Power_Analyser_Enum."READ") -> ("Enable Out"=w839:bool)  [unwired: 10 in]
    n324 = case shown="True" w839 {
      tunnel: w851 -> [w959 w979]
      tunnel: [dbl[] [] ("Data out") w968] -> w850
      tunnel: [dbl[] [] ("Data out") w967] -> w849
      tunnel: [dbl[] [] ("Data out") w966] -> w848
      tunnel: [dbl[] [] ("Data out") w965] -> w846
      tunnel: [w959 w964] -> w838
      frame False {
      }
      frame True {
        n325 = call "FGV_READ.vi"("States"=States."Read Data", "error in"=w979, "Item"=T3 [{"Item"=enum."Urms", "Ch(0:Ch1)"=enum."1"}, {"Item"=enum."Urms", "Ch(0:Ch1)"=enum."2"}, {"Item"=enum."Urms", "Ch(0:Ch1)"=enum."3"}, {"Item"=enum."Udc", "Ch(0:Ch1)"=enum."4"}, {"Item"=enum."Urms", "Ch(0:Ch1)"=enum."123"}] ("Voltage")) -> ("error out"=w976:errorcluster, "Data out"=w968:dbl[])  [unwired: 7 in]
        n326 = call "FGV_READ.vi"("States"=States."Read Data", "error in"=w976, "Item"=T3 [{"Item"=enum."Irms", "Ch(0:Ch1)"=enum."1"}, {"Item"=enum."Irms", "Ch(0:Ch1)"=enum."2"}, {"Item"=enum."Irms", "Ch(0:Ch1)"=enum."3"}, {"Item"=enum."Idc", "Ch(0:Ch1)"=enum."4"}, {"Item"=enum."Irms", "Ch(0:Ch1)"=enum."123"}] ("Current")) -> ("error out"=w972:errorcluster, "Data out"=w967:dbl[])  [unwired: 7 in]
        n327 = call "FGV_READ.vi"("States"=States."Read Data", "error in"=w972, "Item"=T3 [{"Item"=enum."P", "Ch(0:Ch1)"=enum."1"}, {"Item"=enum."P", "Ch(0:Ch1)"=enum."2"}, {"Item"=enum."P", "Ch(0:Ch1)"=enum."3"}, {"Item"=enum."P", "Ch(0:Ch1)"=enum."4"}, {"Item"=enum."P", "Ch(0:Ch1)"=enum."123"}] ("Power")) -> ("error out"=w970:errorcluster, "Data out"=w965:dbl[])  [unwired: 7 in]
        n328 = call "FGV_READ.vi"("States"=States."Read Data", "error in"=w970, "Item"=T3 [{"Item"=enum."f", "Ch(0:Ch1)"=enum."1"}, {"Item"=enum."f", "Ch(0:Ch1)"=enum."2"}, {"Item"=enum."f", "Ch(0:Ch1)"=enum."3"}, {"Item"=enum."f", "Ch(0:Ch1)"=enum."4"}] ("Freq")) -> ("error out"=w964:errorcluster, "Data out"=w966:dbl[])  [unwired: 7 in]
      }
    }
    n329 = Decimate 1D Array(w877) -> (w929:sgl[], w928:sgl[], w927:sgl[], w926:sgl[], w925:sgl[], w924:sgl[], w923:sgl[], w922:sgl[], w921:sgl[], w920:sgl[], w919:sgl[], w918:sgl[], w917:sgl[], w916:sgl[], w915:sgl[], w914:sgl[], w913:sgl[], w912:sgl[], w911:sgl[], w910:sgl[], w909:sgl[], w908:sgl[], w907:sgl[], w906:sgl[], w905:sgl[], w904:sgl[], w903:sgl[], w902:sgl[], w901:sgl[], w900:sgl[], w899:sgl[], w898:sgl[], w897:sgl[], w896:sgl[], w895:sgl[], w894:sgl[], w893:sgl[], w892:sgl[], w891:sgl[], w890:sgl[], w889:sgl[], w888:sgl[], w887:sgl[], w886:sgl[], w885:sgl[], w884:sgl[], w883:sgl[], w882:sgl[], w881:sgl[], w880:sgl[], w879:sgl[], w878:sgl[])
    n330 = Build Array(w929, w928, w927, w926, w925, w924, w923, w922, w921, w920, w919, w918, w917, w916, w915, w914, w913, w912, w911, w910, w909, w908, w907, w906, w905, w904, w903, w902, w901, w900, w899, w898, w897, w896, w895, w894, w893, w892, w891, w890, w889, w888, w887, w886, w885, w884, w883, w882, w881, w880, w879, w878) -> (w876:sgl[][])
    n331 = local read "9220 AI Volt Spare"() -> (w812:cluster{"String":string, "Scalar":sgl}[])
    n332 = call "Scale and Mean.vi"("Slope & Offset"=w935, "Raw In"=w876) -> ("RAW Mean"=→"RAW Mean":sgl[], "Scaled Mean"=w852:sgl[])  [unwired: 7 in, 1 out]
    "Mean" <- w852
    n333 = Wait Until Next ms Multiple(millisecond multiple=u32 1000) -> ()  [unwired: 1 out]
    n334 = Delete From Array(array=w852, length=4, index=w855) -> (deleted portion=→"9219 Universal AI":sgl[], array with subset deleted=w858:sgl[])
    n335 = local read "9208 AI Current"() -> (w814:cluster{"String":string, "Scalar":sgl}[])
    n336 = Delete From Array(array=w858, length=w854, index=w855) -> (deleted portion=w809:sgl[], array with subset deleted=w856:sgl[])
    "9220 AI  Volt  \nPressure" <- w809
    n337 = Delete From Array(array=w856, length=w854, index=w855) -> (deleted portion=w815:sgl[], array with subset deleted=w857:sgl[])
    "9208 AI Current" <- w815
    n338 = Index Array(array=w846) -> (element #1=→"P1(W)":dbl, element #2=→"P2(W)":dbl, element #3=→"P3(W)":dbl, element #4=→"P DC(W)":dbl, element #5=→"P123(W)":dbl)  [unwired: 5 in]
    n339 = Delete From Array(array=w857, length=w854, index=w855) -> (deleted portion=w810:sgl[])  [unwired: 1 out]
    "9220 AI Volt Spare" <- w810
    n340 = for {
      tunnel: w812 -> [w947] mode=indexing
      tunnel: w810 -> [w949] mode=indexing
      tunnel: [w948] -> w811 mode=indexing
      n341 = Bundle By Name(cluster=w947, "Scalar"=w949) -> (w948:cluster{"String":string, "Scalar":sgl})
    }
    n342 = local write "9220 AI Volt Spare"(w811) -> ()
    n343 = local read "9220 AI  Volt  Pressure"() -> (w817:cluster{"String":string, "Scalar":sgl}[])
    n344 = for {
      tunnel: w814 -> [w952] mode=indexing
      tunnel: w815 -> [w951] mode=indexing
      tunnel: [w950] -> w813 mode=indexing
      n345 = Bundle By Name(cluster=w952, "Scalar"=w951) -> (w950:cluster{"String":string, "Scalar":sgl})
    }
    n346 = local write "9208 AI Current"(w813) -> ()
    n347 = Build Array (concatenate)(w850, w849, w846, w848) -> (→"PA Data":dbl[])
    n348 = call "READ DUBAS DATA.vi"("STATES"=DUBAS_FGV_STATES."READ DATA", "error in (no error)"=w838) -> ("error out"=w819:errorcluster, "BUBAS DATA"=w836:dbl[])  [unwired: 8 in]
    n349 = Index Array(array=w852, index #5=38 ("index (row)"), index #12=4 ("index"), index #19=12 ("index"), index #23=20 ("index"), index #27=11 ("index")) -> (element #1=→"Mod1/CH0":sgl, element #2=→"Mod1/CH1":sgl, element #3=→"Mod1/CH2":sgl, element #4=→"Mod1/CH3":sgl, element #12=→"Coolant-In_P":sgl, element #13=→"Coolant-Out_P":sgl, element #14=→"Exhaust_P":sgl, element #15=→"Oil_P":sgl, element #16=→"Intercooler-In_P":sgl, element #17=→"Intercooler-Out_P":sgl, element #18=→"Misc_P":sgl, element #19=→"P Spare 1":sgl, element #20=→"P Spare 2":sgl, element #21=→"P Spare 3":sgl, element #22=→"P Spare 4":sgl, element #23=→"AI0":sgl, element #24=→"AI1":sgl, element #25=→"AI2":sgl, element #26=→"Engine RPM":sgl)  [unwired: 22 in, 8 out]
    n350 = for {
      tunnel: w817 -> [w955] mode=indexing
      tunnel: w809 -> [w954] mode=indexing
      tunnel: [w953] -> w816 mode=indexing
      n351 = Bundle By Name(cluster=w955, "Scalar"=w954) -> (w953:cluster{"String":string, "Scalar":sgl})
    }
    n352 = local write "9220 AI  Volt  Pressure"(w816) -> ()
    n353 = call <vilib>:"Clear Errors.vi"("error in (no error)"=w819) -> ()  [unwired: 5 in, 2 out]
    n354 = Number To Fractional String(number=w836) -> (F-format string=w828:string[])  [unwired: 3 in]
    n355 = Index Array(array=w828, index #1=13 ("index"), index #2=10 ("index")) -> (element #1=w835:string, element #2=w826:string)
    n356 = Index Array(array=w828) -> (element #1=w823:string, element #2=w822:string, element #3=w821:string)  [unwired: 3 in]
    "POWER" <- w821
    "CURRENT" <- w822
    "VOLTAGE" <- w823
    n357 = Equal?(x=w826, y="224") -> (x = y?=w834:bool)
    n358 = case shown="\"226\", Default" w835 {
      tunnel: ["CV" "CI" "CP"] -> w824
      frame "226", Default {
      }
      frame "227" {
      }
      frame "228" {
      }
    }
    "CONTROL SELECTION" <- w824
    n359 = Select(t="HIGH CURRENT", s=w834, f="HIGH VOLTAGE") -> (s? t:f=w825:string)
    "HVHC SELECTION" <- w825
    n360 = call "Application Stop.vi"("Command"=enum16{"Read ", "Write "}."Read ") -> ("STOP"=w862:bool)  [unwired: 9 in, 1 out]
    n361 = local read "Stop All"() -> (w864:bool)
    n362 = Build Array(w825, w824, w823, w822, w821) -> (w820:string[])
    n363 = call "READ DUBAS DATALOG.vi"("STATES"=DUBAS_DTALOG_FGV_STATES."WRITE DATA", "DUBAS DATA IN"=w820) -> ()  [unwired: 8 in, 2 out]
    n364 = Compound Arithmetic op=OR(w865, w862, w864) -> (w863:bool)
  }
  n365 = while {
    shift-right: [w1005] -> _
    shift-left: w70 -> [w1049]
    shift-right: [w995] -> _
    shift-left: w17 -> [w1048]
    tunnel: w16 -> [w1013]
    stop <- w994 stop-if-true
    n366 = Dequeue Element(queue=w1049, error in (no error)=w1048) -> (queue out=w1005:refnum<queue>, element=w1015:sgl[], error out=w995:errorcluster)  [unwired: 1 in, 1 out]
    n367 = Decimate 1D Array(w1015) -> (w1016:sgl[], w1017:sgl[], w1018:sgl[], w1019:sgl[], w1020:sgl[], w1021:sgl[], w1022:sgl[], w1023:sgl[], w1024:sgl[], w1025:sgl[], w1026:sgl[], w1027:sgl[], w1028:sgl[], w1029:sgl[], w1030:sgl[], w1031:sgl[], w1032:sgl[], w1033:sgl[], w1034:sgl[], w1035:sgl[], w1036:sgl[], w1037:sgl[], w1038:sgl[], w1039:sgl[], w1040:sgl[], w1041:sgl[], w1042:sgl[], w1043:sgl[], w1044:sgl[], w1045:sgl[], w1046:sgl[], w1047:sgl[])
    n368 = Build Array(w1016, w1017, w1018, w1019, w1020, w1021, w1022, w1023, w1024, w1025, w1026, w1027, w1028, w1029, w1030, w1031, w1032, w1033, w1034, w1035, w1036, w1037, w1038, w1039, w1040, w1041, w1042, w1043, w1044, w1045, w1046, w1047) -> (w1014:sgl[][])
    n369 = local read "Thermocouple"() -> (w985:cluster{"String":string, "Scalar":sgl}[])
    n370 = call "Scale and Mean.vi"("Slope & Offset"=w1013, "Raw In"=w1014) -> ("RAW Mean"=→"RAW Mean TC":sgl[], "Scaled Mean"=w988:sgl[])  [unwired: 7 in, 1 out]
    "Mean tc" <- w988
    n371 = Wait Until Next ms Multiple(millisecond multiple=u32 100) -> ()  [unwired: 1 out]
    n372 = Delete From Array(array=w988, length=16, index=0) -> (deleted portion=w982:sgl[], array with subset deleted=w981:sgl[])
    "Thermocouple" <- w982
    "Thermocouple Spare" <- w981
    n373 = for {
      tunnel: w985 -> [w1055] mode=indexing
      tunnel: w982 -> [w1054] mode=indexing
      tunnel: [w1053] -> w986 mode=indexing
      n374 = Bundle By Name(cluster=w1055, "Scalar"=w1054) -> (w1053:cluster{"String":string, "Scalar":sgl})
    }
    n375 = Index Array(array=w988) -> (element #1=→"Intercooler_In_T":sgl, element #2=→"Intercooler_Out_T":sgl, element #3=→"Exhaust_T":sgl, element #4=→"Oil_T":sgl, element #5=→"Coolant_Inlet_T":sgl, element #6=→"Coolant_Outlet_T":sgl, element #7=→"Basement_T":sgl, element #8=→"T Spare 1":sgl, element #9=→"T Spare 2":sgl, element #10=→"T Spare 3":sgl, element #11=→"T Spare 4":sgl, element #12=→"T Spare 5":sgl, element #13=→"T Spare 6":sgl, element #14=→"T Spare 7":sgl, element #15=→"T Spare 8":sgl)  [unwired: 15 in]
    n376 = local write "Thermocouple"(w986) -> ()
    n377 = local read "Thermocouple Spare"() -> (w984:cluster{"String":string, "Scalar":sgl}[])
    n378 = local read "Stop All"() -> (w993:bool)
    n379 = for {
      tunnel: w984 -> [w1052] mode=indexing
      tunnel: w981 -> [w1051] mode=indexing
      tunnel: [w1050] -> w983 mode=indexing
      n380 = Bundle By Name(cluster=w1052, "Scalar"=w1051) -> (w1050:cluster{"String":string, "Scalar":sgl})
    }
    n381 = local write "Thermocouple Spare"(w983) -> ()
    n382 = call "Application Stop.vi"("Command"=enum16{"Read ", "Write "}."Read ") -> ("STOP"=w992:bool)  [unwired: 9 in, 1 out]
    n383 = Compound Arithmetic op=OR(w995, w993, w992) -> (w994:bool)
  }
  n384 = call <vilib>:"Add State(s) to Queue__JKI_lib_State_Machine.vi"("State(s) in (\"\")"=w77) -> ("States Out"=w78:string)  [unwired: 14 in]
  n385 = while "JKI State Machine 2018" {
    shift-right: [w1063] -> _
    shift-left: _ -> [w1062]
    shift-right: [w1065] -> w79
    shift-left: errorcluster {"status"=FALSE, "code"=0, "source"=""} ("error out") -> [w1060]
    shift-right: [w1064] -> _
    shift-left: w78 -> [w1066]
    stop <- w1058 stop-if-true
    w1061 = 100  # Timeout
    n386 = call <vilib>:"Parse State Queue__JKI_lib_State_Machine.vi"("State Queue"=w1066, "Error In (no error)"=w1060) -> ("Remaining States"=w1068:string, "Current State"=w1069:string, "Arguments"=w1067:string)  [unwired: 11 in]
    n387 = case shown="\"Write Headers\"" w1069 {
      selector: w1069 -> [_ _ w1136 _ _ _ _ _ _ _ _ _ _ _ _ _ _ _ _ _ _ _ _ _]
      tunnel: w1068 -> [w1076 w1135 w1140 w1159 w1165 w1170 w1174 w1191 w1197 w1201 w1212 w1217 w1297 w1308 w1377 w1396 w1412 w1416 w1418 w1423 w1428 w1486 w1602 w1639]
      tunnel: w1067 -> [_ _ _ _ _ _ _ _ _ _ _ _ w1292 w1302 _ _ _ _ _ _ _ _ _ _]
      tunnel: w1062 -> [w1074 w1132 w1138 w1152 w1162 w1168 w1171 _ w1192 w1198 w1209 w1215 w1295 w1304 w1374 w1394 w1410 w1413 w1419 w1420 w1426 w1480 w1598 w1635]
      tunnel: [w1073 w1133 w1142 w1156 errorcluster {"status"=FALSE, "code"=0, "source"=""} ("error out") w1167 w1172 w1188 w1193 w1199 w1204 w1213 w1293 w1305 w1375 w1384 w1401 w1414 w1417 w1421 w1424 w1482 w1599 w1631] -> w1065
      tunnel: w1060 -> [w1072 w1133 w1141 w1156 w1161 w1167 w1172 w1188 w1194 w1199 w1206 w1214 w1294 w1306 w1375 w1385 w1402 w1414 w1417 w1421 w1425 w1484 w1600 w1637]
      tunnel: [w1075 w1134 w1139 w1158 w1164 w1169 w1173 w1190 w1196 w1200 w1211 w1216 w1296 w1307 w1376 w1395 w1411 w1415 w1418 w1422 w1427 w1487 w1603 w1640] -> w1064
      tunnel: [_ _ _ _ _ TRUE _ _ _ _ _ _ _ _ _ _ _ _ _ _ _ _ _ _] -> w1059
      tunnel: [w1071 w1132 w1138 w1157 w1162 w1168 w1171 w1189 w1192 w1198 w1209 w1215 w1295 w1304 w1374 w1394 w1410 w1413 w1419 w1420 w1426 w1479 w1596 w1635] -> w1063
      tunnel: w1061 -> [w1070 _ _ _ _ _ _ _ _ _ _ _ _ _ _ _ _ _ _ _ _ _ _ _]
      frame "", "Event Structure", "Idle" {
        # "executes when the state queue is empty"
        n388 = event shown="[3] \"Settings Button\": Value Change" {
          selector: _ -> [_ _ _ _ _ _]
          dyn-events: _ -> [_ _ _ _ _ _]
          timeout: w1070 -> [_ _ _ _ _ _]
          tunnel: w1076 -> [w1084 w1090 w1102 w1112 w1120 w1131]
          tunnel: [w1083 w1089 w1103 w1112 w1120 w1130] -> w1075
          tunnel: w1074 -> [w1081 w1087 w1105 w1113 w1121 w1128]
          tunnel: [w1082 w1088 w1106 w1111 w1124 w1129] -> w1073
          tunnel: w1072 -> [w1082 w1088 w1106 w1111 w1125 w1129]
          tunnel: [w1081 w1087 w1104 w1113 w1121 w1128] -> w1071
          event Timeout {
            n389 = event-data() -> ()  [unwired: 1 in, 1 out]
            n390 = Unbundle By Name(w1081) -> ("Data Log"=w1080:bool)
            n391 = Select(t="Log Data", s=w1080, f="") -> (s? t:f=w1078:string)
            n392 = call <vilib>:"Add State(s) to Queue__JKI_lib_State_Machine.vi"("State(s) in (\"\")"=w1084, "State(s) at Back (\"\")"=w1078) -> ("States Out"=w1083:string)  [unwired: 13 in]
          }
          event "Stop": Value Change {
            # "Exit Button Value Change (pressed) Event\n(this executes Macro: Exit to terminate the VI)"
            n393 = event-data() -> ()  [unwired: 1 in, 6 out]
            n394 = call <vilib>:"Add State(s) to Queue__JKI_lib_State_Machine.vi"("State(s) in Front (\"\")"="Macro: Exit", "State(s) in (\"\")"=w1090) -> ("States Out"=w1089:string)  [unwired: 13 in]
            "Stop All" <- TRUE
          }
          event "Data_Log": Value Change {
            n395 = event-data() -> ("NewVal"=w1091:bool)  [unwired: 1 in]
            n396 = disable-structure shown="Disabled" {
              frame Disabled {
                n397 = call <vilib>:"Application Directory.vi"() -> ("Application Directory"=w1110:path)
                n398 = Build Path(base path=w1110, name or relative path="data\\enable.csv") -> (appended path=w1108:path)
                n399 = call-poly <vilib>:"Read Delimited Spreadsheet.vi"("file path (dialog if empty)"=w1108) -> ("all rows"=w1107:i64[][])  [unwired: 9 in, 5 out]
                n400 = Index Array(array=w1107) -> ()  [unwired: 2 in, 1 out]
              }
              frame Enabled {
              }
            }
            n401 = call "Power Analyser FGV Enable.vi"("Enum"=Power_Analyser_Enum."WRITE", "Enable"=w1091) -> ()  [unwired: 9 in, 1 out]
            n402 = Select(t=States."Open Com" ("States"), s=w1091, f=States."Close Comm") -> (s? t:f=w1095:T5)
            n403 = Select(t=T16."Disabled and Grayed Out" ("Disabled"), s=w1091, f=T16."Enabled" ("Disabled")) -> (s? t:f=w1092:T16)
            n404 = Bundle By Name(cluster=w1105, "Data Log"=w1091) -> (w1104:T18)
            n405 = call "FGV_READ.vi"("States"=w1095) -> ()  [unwired: 9 in, 2 out]
            n406 = Select(t="Write Headers", s=w1091, f="Stop Logging") -> (s? t:f=w1100:string)
            n407 = call <vilib>:"Add State(s) to Queue__JKI_lib_State_Machine.vi"("State(s) in (\"\")"=w1102, "State(s) at Back (\"\")"=w1100) -> ("States Out"=w1103:string)  [unwired: 13 in]
            n408 = property on="Settings Button" class="Bool"("DisabledEnum"=w1092) -> ()  [unwired: 2 in, 2 out]
          }
          event "Settings Button": Value Change {
            n409 = event-data() -> ()  [unwired: 1 in, 6 out]
            n410 = disable-structure shown="Disabled" {
              frame Disabled {
                n411 = flat-sequence {
                  tunnel: [w1114] -> _
                  frame #0 {
                    n412 = call "enable disable channel for saving.vi"() -> ()  [unwired: 12 in]
                  }
                  frame #1 {
                    n413 = call <vilib>:"Application Directory.vi"() -> ("Application Directory"=w1119:path)
                    n414 = Build Path(base path=w1119, name or relative path="data\\enable.csv") -> (appended path=w1118:path)
                    n415 = call-poly <vilib>:"Read Delimited Spreadsheet.vi"("file path (dialog if empty)"=w1118) -> ("all rows"=w1117:i64[][])  [unwired: 9 in, 5 out]
                    n416 = Index Array(array=w1117) -> (element=w1116:i64[])  [unwired: 2 in]
                    n417 = Not Equal To 0?(x=w1116) -> (x != 0?=w1114:bool[])
                  }
                }
              }
              frame Enabled {
              }
            }
          }
          event "Column Header": Value Change {
            n418 = event-data() -> ()  [unwired: 1 in, 6 out]
            n419 = local read "Column Header"() -> (w1122:string[])
            n420 = call "Header Column FGV.vi"("Command"=T6."Write Data", "error in (no error)"=w1125, "Column Header"=w1122) -> ("error out"=w1124:errorcluster)  [unwired: 7 in, 1 out]
          }
          event Panel Close? {
            # "Discard the event because we'll close the front panel ourselves in Macro: Exit"
            # "Close Panel button (pressed) Event\n(this executes Macro: Exit to terminate the VI)"
            n421 = event-data() -> ()  [unwired: 1 in, 1 out]
            n422 = call <vilib>:"Add State(s) to Queue__JKI_lib_State_Machine.vi"("State(s) in Front (\"\")"="Macro: Exit", "State(s) in (\"\")"=w1131) -> ("States Out"=w1130:string)  [unwired: 13 in]
            n423 = event-data("Discard?"=TRUE) -> ()  [unwired: 1 in, 1 out]
          }
        }
      }
      frame "---------- Core ----------" {
        # "Do not put any code in this frame.\n(it is a separator no-op)"
        n424 = call <vilib>:"Add State(s) to Queue__JKI_lib_State_Machine.vi"("State(s) in (\"\")"=w1135) -> ("States Out"=w1134:string)  [unwired: 14 in]
      }
      frame Default {
        w1145 = 42 items=["No error", "Argument error", "Memory is full", "Out of zone", "End of file", "File already open", "Generic file I/O error", "File not found", "File permission error", "Disk is full", "Duplicate path", "Too many files open", "System feature not enabled", "Resource file not found", "Cannot add resource", "Resource not found", "Image not found", "Image memory error", "Pen does not exist", "Config type invalid", "Config token not found", "Config parse error", "Config memory error", "Bad external code format", "Bad external code offset", "External code not present", "Null window", "Destroy window error", "Null menu", "Print aborted", "Bad print record", "Print driver error", "Windows error during printing", "Memory error during printing", "Print dialog error", "Generic print error", "Invalid device refnum", "Device not found", "Device parameter error", "Device unit error", "Cannot open device", "Device call aborted", "Generic error", "Cancelled by user", "Object ID too low", "Object ID too high", "Object not in heap", "Unknown heap", "Unknown object (invalid DefProc)", "Unknown object (DefProc not in table)", "Message out of range", "Invalid (null) method", "Unknown message", "Manager call not supported", "Bad address", "Network operation in progress", "Network operation timed out", "Connection is busy", "Network attribute not supported", "Network error", "Address in use", "System out of memory", "Connection aborted", "Connection refused", "Not connected", "Already connected", "Connection closed", "Initialization error (interapplication manager)", "Bad occurrence", "Wait on unbound occurrence handler", "Occurrence queue overflow", "Datalog type conflict", "Unused", "Unrecognized type (interapplication manager)", "Memory corrupt", "Failed to make temporary DLL", "Old CIN version", "Drag socket not found", "Failed to load drop-object", "Failed to register OLE object", "Failed to release OLE object", "Format specifier type mismatch", "Unknown format specifier", "Too few format specifiers", "Too many format specifiers", "Scan failed", "Newer CIN version", "Error converting to variant", "Runtime menu error", "Password tampered", "Variant attribute not found", "Incompatible variant data type", "Event data is not available", "Event Store is not present", "Occurrence is not found", "Event Queue is not created", "Event info is not available", "Refnum passed is NULL", "Error retrieving Class GUID", "Error retrieving CoClass GUID", "Error retrieving TypeLib GUID.", "Bad built application magic bytes.", "Specific driver is different from the specific driver associated with the Logical Name.", "There is no session opened to the class driver.", "Max Error", "MAX - Error with config objects", "MAX - Error loading configuration", "MAX - Group not supported"]
        # "Current State"
        # "Do not delete, rename, or modify this frame.\n(this is used to capture unhandled states and typos)"
        # "Handle mistyped state name (developer tool)"
        n425 = Format Into String(format string="Software Exception: Unhandled State \"%s\"." ("message"), error in=w1141, w1136) -> (resulting string=w1144:string, error out=w1143:errorcluster)  [unwired: 1 in]
        n426 = call <vilib>:"Error Cluster From Error Code.vi"("show call chain? (False)"=TRUE, "error in (no error)"=w1143, "error message (\"\")"=w1144, "error code (0)"=w1145) -> ("error out"=w1142:errorcluster)  [unwired: 5 in]
        n427 = call <vilib>:"Add State(s) to Queue__JKI_lib_State_Machine.vi"("State(s) in (\"\")"=w1140) -> ("States Out"=w1139:string)  [unwired: 14 in]
      }
      frame "Initialize Core Data" {
        # "Do not delete, rename, or modify this frame.\n(this is used to determine panel behavior on exit)"
        # "originally closed?"
        # "exe?"
        # "If panel starts closed or is an EXE, then close it when we exit"
        n428 = property class="VI"() -> ("FP.State"=w1149:T7)  [unwired: 2 in, 2 out]
        n429 = property class="App"() -> ("App.Kind"=w1155:T8)  [unwired: 2 in, 2 out]
        n430 = control-ref of="Current VI Reference"() -> (w1150:refnum<vi>)
        n431 = Equal?(x=w1149, y=T7."Closed" ("Front Panel Window:State")) -> (x = y?=w1147:bool)
        n432 = Equal?(x=w1155, y=T8."Run Time System" ("Application:Kind")) -> (x = y?=w1153:bool)
        n433 = Or(x=w1147, y=w1153) -> (x .or. y?=w1151:bool)
        n434 = Bundle By Name(cluster=w1152, "Core.Current VI Reference"=w1150, "Core.Close Panel on Exit?"=w1151) -> (w1157:T18)
        n435 = call <vilib>:"Add State(s) to Queue__JKI_lib_State_Machine.vi"("State(s) in (\"\")"=w1159) -> ("States Out"=w1158:string)  [unwired: 14 in]
      }
      frame "Error Handler" {
        # "Unhandled Error -- Display it"
        # "Handle any errors here.\nYou can also output any states to clean-up after errors occur"
        # "Clear error"
        n436 = call <vilib>:"General Error Handler.vi"("error in (no error)"=w1161) -> ()  [unwired: 10 in, 5 out]
        n437 = call <vilib>:"Add State(s) to Queue__JKI_lib_State_Machine.vi"("State(s) in Front (\"\")"="/* Post Error States", "State(s) in (\"\")"=w1165) -> ("States Out"=w1164:string)  [unwired: 13 in]
      }
      frame "Exit" {
        # "Do not put any code in this frame.\n(No errors that occur here will be handled.)"
        n438 = call <vilib>:"Add State(s) to Queue__JKI_lib_State_Machine.vi"("State(s) in (\"\")"=w1170) -> ("States Out"=w1169:string)  [unwired: 14 in]
      }
      frame "---------- Data ----------" {
        # "Do not put any code in this frame.\n(It is a separator no-op. You can make a copy of this frame to create a new Data frame)"
        n439 = call <vilib>:"Add State(s) to Queue__JKI_lib_State_Machine.vi"("State(s) in (\"\")"=w1174) -> ("States Out"=w1173:string)  [unwired: 14 in]
      }
      frame "Data: Initialize" {
        w1175 = path ""  # location
        w1176 = bool[][] []  # Log Active
        w1178 = FALSE  # Data Log
        w1179 = refnum<k20> refnum  # ExpansionChassFPGA
        w1187 = T13 {"Current VI Reference"=refnum, "Close Panel on Exit?"=FALSE}  # Core
        # "Initialize the shift-register data, here.\n(data names are defined by what you wire into the bundle function)"
        n440 = control-ref of="Intercooler_In_T"() -> (w1186:refnum<vi>)
        n441 = control-ref of="Coolant_Inlet_T"() -> (w1185:refnum<vi>)
        n442 = control-ref of="Coolant_Outlet_T"() -> (w1184:refnum<vi>)
        n443 = control-ref of="Basement_T"() -> (w1183:refnum<vi>)
        n444 = control-ref of="Exhaust_T"() -> (w1182:refnum<vi>)
        n445 = control-ref of="Oil_T"() -> (w1181:refnum<vi>)
        n446 = control-ref of="Intercooler_Out_T"() -> (w1180:refnum<vi>)
        n447 = Bundle("Core"=w1187, "Intercooler_In_T"=w1186, "Coolant_Inlet_T"=w1185, "Coolant_Outlet_T"=w1184, "Basement_T"=w1183, "Exhaust_T"=w1182, "Oil_T"=w1181, "Intercooler_Out_T"=w1180, "ExpansionChassFPGA"=w1179, "Data Log"=w1178, "LogFile Refnum"=refnum<file> refnum, "Log Active"=w1176, "location"=w1175) -> (w1189:T18)  [unwired: 1 in]
        n448 = call <vilib>:"Add State(s) to Queue__JKI_lib_State_Machine.vi"("State(s) in (\"\")"=w1191) -> ("States Out"=w1190:string)  [unwired: 14 in]
      }
      frame "Data: Cleanup" {
        # "Cleanup any data and references, here.\n(this is called automatically, by the Macro: Exit)"
        n449 = Unbundle By Name(w1192) -> ("Core.Current VI Reference"=w1195:refnum<vi>)
        n450 = Close Reference(reference=w1195, error in (no error)=w1194) -> (error out=w1193:errorcluster)
        n451 = call <vilib>:"Add State(s) to Queue__JKI_lib_State_Machine.vi"("State(s) in (\"\")"=w1197) -> ("States Out"=w1196:string)  [unwired: 14 in]
      }
      frame "---------- UI ----------" {
        # "Do not put any code in this frame.\n(It is a separator no-op. You can make a copy of this frame to create a new UI frame)"
        n452 = call <vilib>:"Add State(s) to Queue__JKI_lib_State_Machine.vi"("State(s) in (\"\")"=w1201) -> ("States Out"=w1200:string)  [unwired: 14 in]
      }
      frame "UI: Initialize" {
        w1203 = FALSE
        # "Initialize the User Interface, here.\n(this is called automatically, by the Macro: Init)"
        n453 = Unbundle By Name(w1209) -> ("Core.Current VI Reference"=w1208:refnum<vi>)
        n454 = property class="VI"(reference=w1208, error in=w1206, "FP.Monitor"=u16 2 ("Front Panel Window:Monitor")) -> (error out=w1205:errorcluster)  [unwired: 1 out]
        n455 = call <vilib>:"Clear Errors.vi"("error in (no error)"=w1205) -> ("error out"=w1204:errorcluster)  [unwired: 5 in, 1 out]
        n456 = local write "Data_Log"(w1203) -> ()
        n457 = local write "Stop All"(w1203) -> ()
        n458 = property on="Settings Button" class="Bool"("DisabledEnum"=T16."Enabled" ("Disabled")) -> ()  [unwired: 2 in, 2 out]
        n459 = call <vilib>:"Add State(s) to Queue__JKI_lib_State_Machine.vi"("State(s) in (\"\")"=w1212, "State(s) at Back (\"\")"="Set Scale.Marker" ("State(s) at Back (\"\")")) -> ("States Out"=w1211:string)  [unwired: 13 in]
      }
      frame "Set Scale.Marker" {
        n460 = disable-structure shown="Enabled" {
          frame Disabled {
            n461 = Bundle(60.0, u32 16776002) -> (w1290:cluster{dbl, u32})  [unwired: 1 in]
            n462 = Bundle(70.0, u32 16711680) -> (w1289:cluster{dbl, u32})  [unwired: 1 in]
            n463 = Bundle(100.0, u32 0) -> (w1288:cluster{dbl, u32})  [unwired: 1 in]
            n464 = Bundle(40.0, u32 16776002) -> (w1262:cluster{dbl, u32})  [unwired: 1 in]
            n465 = Bundle(50.0, u32 16711680) -> (w1263:cluster{dbl, u32})  [unwired: 1 in]
            n466 = Bundle(60.0, u32 0) -> (w1264:cluster{dbl, u32})  [unwired: 1 in]
            n467 = Bundle(70.0, u32 2027264) -> (w1279:cluster{dbl, u32})  [unwired: 1 in]
            n468 = Bundle(90.0, u32 16776002) -> (w1278:cluster{dbl, u32})  [unwired: 1 in]
            n469 = Bundle(100.0, u32 16711680) -> (w1277:cluster{dbl, u32})  [unwired: 1 in]
            n470 = Bundle(120.0, u32 0) -> (w1276:cluster{dbl, u32})  [unwired: 1 in]
            n471 = Bundle(0.0, u32 2027264) -> (w1291:cluster{dbl, u32})  [unwired: 1 in]
            n472 = Bundle(0.0, u32 2027264) -> (w1261:cluster{dbl, u32})  [unwired: 1 in]
            n473 = Bundle(0.0, u32 16776002) -> (w1275:cluster{dbl, u32})  [unwired: 1 in]
            n474 = Build Array(w1291, w1290, w1289, w1288) -> (w1222:cluster{dbl, u32}[])
            n475 = Build Array(w1261, w1262, w1263, w1264) -> (w1220:cluster{dbl, u32}[])
            n476 = Build Array(w1275, w1279, w1278, w1277, w1276) -> (w1221:cluster{dbl, u32}[])
            n477 = property on="Intercooler_Out_T" class="Slide (strict)"("Scale.MarkerVals[]"=w1222) -> ()  [unwired: 2 in, 2 out]
            n478 = property on="Intercooler_In_T" class="Slide (strict)"("Scale.MarkerVals[]"=w1222) -> ()  [unwired: 2 in, 2 out]
            n479 = property on="Coolant_Inlet_T" class="Slide (strict)"("Scale.MarkerVals[]"=w1221) -> ()  [unwired: 2 in, 2 out]
            n480 = property on="Coolant_Outlet_T" class="Slide (strict)"("Scale.MarkerVals[]"=w1221) -> ()  [unwired: 2 in, 2 out]
            n481 = property on="Basement_T" class="Slide (strict)"("Scale.MarkerVals[]"=w1220) -> ()  [unwired: 2 in, 2 out]
            n482 = Bundle(800.0, u32 16776002) -> (w1250:cluster{dbl, u32})  [unwired: 1 in]
            n483 = Bundle(900.0, u32 16711680) -> (w1251:cluster{dbl, u32})  [unwired: 1 in]
            n484 = Bundle(1000.0, u32 0) -> (w1252:cluster{dbl, u32})  [unwired: 1 in]
            n485 = Bundle(40.0, u32 16776002) -> (w1239:cluster{dbl, u32})  [unwired: 1 in]
            n486 = Bundle(70.0, u32 6618880) -> (w1238:cluster{dbl, u32})  [unwired: 1 in]
            n487 = Bundle(110.0, u32 16776002) -> (w1237:cluster{dbl, u32})  [unwired: 1 in]
            n488 = Bundle(120.0, u32 16713728) -> (w1236:cluster{dbl, u32})  [unwired: 1 in]
            n489 = Bundle(140.0, u32 0) -> (w1235:cluster{dbl, u32})  [unwired: 1 in]
            n490 = Bundle(0.0, u32 2027264) -> (w1249:cluster{dbl, u32})  [unwired: 1 in]
            n491 = Bundle(0.0, u32 16713728) -> (w1240:cluster{dbl, u32})  [unwired: 1 in]
            n492 = Build Array(w1249, w1250, w1251, w1252) -> (w1219:cluster{dbl, u32}[])
            n493 = Build Array(w1240, w1239, w1238, w1237, w1236, w1235) -> (w1218:cluster{dbl, u32}[])
            n494 = property on="Exhaust_T" class="Slide (strict)"("Scale.MarkerVals[]"=w1219) -> ()  [unwired: 2 in, 2 out]
            n495 = property on="Oil_T" class="Slide (strict)"("Scale.MarkerVals[]"=w1218) -> ()  [unwired: 2 in, 2 out]
          }
          frame Enabled {
          }
        }
        n496 = call <vilib>:"Clear Errors.vi"("error in (no error)"=w1214) -> ("error out"=w1213:errorcluster)  [unwired: 5 in, 1 out]
        n497 = call <vilib>:"Add State(s) to Queue__JKI_lib_State_Machine.vi"("State(s) in (\"\")"=w1217) -> ("States Out"=w1216:string)  [unwired: 14 in]
      }
      frame "UI: Cursor Set" {
        # "Argument"
        # "Set and Unset Cursor Busy.\n(Usage: \"UI: Cursor Set >> Busy|Idle\")"
        n498 = case shown="\"Idle\", Default" w1292 {
          tunnel: w1294 -> [w1299 w1301]
          tunnel: [w1298 w1300] -> w1293
          frame "Idle", Default {
            n499 = call <vilib>:"Unset Busy.vi"("error in (no error)"=w1299) -> ("error out"=w1298:errorcluster)  [unwired: 10 in]
          }
          frame "Busy" {
            n500 = call <vilib>:"Set Busy.vi"("error in (no error)"=w1301) -> ("error out"=w1300:errorcluster)  [unwired: 9 in, 1 out]
          }
        }
        n501 = call <vilib>:"Add State(s) to Queue__JKI_lib_State_Machine.vi"("State(s) in (\"\")"=w1297) -> ("States Out"=w1296:string)  [unwired: 14 in]
      }
      frame "UI: Front Panel State" {
        # "Argument"
        # "Set Front Panel Open or Closed\n(Usage: \"UI: Front Panel State >> Open|Close\")"
        n502 = Unbundle By Name(w1304) -> ("Core.Current VI Reference"=w1303:refnum<vi>)
        n503 = case shown="\"Minimize\", \"Minimized\"" w1302 {
          tunnel: w1306 -> [w1314 w1329 w1340 w1353 w1366]
          tunnel: [w1316 w1330 w1342 w1355 w1368] -> w1305
          tunnel: w1303 -> [w1315 w1327 w1341 w1354 w1367]
          frame "Open", "Standard", Default {
            w1309 = T7."Standard" ("State")
            n504 = property class="VI"(reference=w1315, error in=w1314) -> (reference out=w1312:refnum<vi>, error out=w1313:errorcluster, "FP.State"=w1311:T7)
            n505 = Not Equal?(x=w1311, y=w1309) -> (x != y?=w1310:bool)
            n506 = case shown="True" w1310 {
              tunnel: [w1320 w1322] -> w1316
              tunnel: w1313 -> [w1319 w1322]
              tunnel: w1312 -> [w1318 _]
              tunnel: w1309 -> [w1317 _]
              frame True {
                n507 = invoke class="VI" method="FP.Open"(reference=w1318, error in=w1319, "Activate"=TRUE, "State"=w1317) -> (error out=w1320:errorcluster)  [unwired: 1 in, 4 out]
              }
              frame False {
              }
            }
          }
          frame "Close", "Closed" {
            n508 = property class="VI"(reference=w1327, error in=w1329) -> (reference out=w1326:refnum<vi>, error out=w1328:errorcluster, "FP.State"=w1324:T7)
            n509 = Not Equal?(x=w1324, y=T7."Closed" ("Front Panel Window:State")) -> (x != y?=w1323:bool)
            n510 = case shown="True" w1323 {
              tunnel: [w1331 w1334] -> w1330
              tunnel: w1328 -> [w1331 w1333]
              tunnel: w1326 -> [_ w1332]
              frame False {
              }
              frame True {
                n511 = invoke class="VI" method="FP.Close"(reference=w1332, error in=w1333) -> (error out=w1334:errorcluster)  [unwired: 1 in, 2 out]
              }
            }
          }
          frame "Hidden", "Hide" {
            w1335 = T7."Hidden" ("State")
            n512 = property class="VI"(reference=w1341, error in=w1340) -> (reference out=w1338:refnum<vi>, error out=w1339:errorcluster, "FP.State"=w1337:T7)
            n513 = Not Equal?(x=w1337, y=w1335) -> (x != y?=w1336:bool)
            n514 = case shown="True" w1336 {
              tunnel: [w1346 w1347] -> w1342
              tunnel: w1339 -> [w1345 w1347]
              tunnel: w1338 -> [w1344 _]
              tunnel: w1335 -> [w1343 _]
              frame True {
                n515 = invoke class="VI" method="FP.Open"(reference=w1344, error in=w1345, "State"=w1343) -> (error out=w1346:errorcluster)  [unwired: 2 in, 4 out]
              }
              frame False {
              }
            }
          }
          frame "Minimize", "Minimized" {
            w1348 = T7."Minimized" ("State")
            n516 = property class="VI"(reference=w1354, error in=w1353) -> (reference out=w1351:refnum<vi>, error out=w1352:errorcluster, "FP.State"=w1350:T7)
            n517 = Not Equal?(x=w1350, y=w1348) -> (x != y?=w1349:bool)
            n518 = case shown="False" w1349 {
              tunnel: [w1359 w1360] -> w1355
              tunnel: w1352 -> [w1358 w1360]
              tunnel: w1351 -> [w1357 _]
              tunnel: w1348 -> [w1356 _]
              frame True {
                n519 = invoke class="VI" method="FP.Open"(reference=w1357, error in=w1358, "State"=w1356) -> (error out=w1359:errorcluster)  [unwired: 2 in, 4 out]
              }
              frame False {
              }
            }
          }
          frame "Maximize", "Maximized" {
            w1361 = T7."Maximized" ("State")
            n520 = property class="VI"(reference=w1367, error in=w1366) -> (reference out=w1364:refnum<vi>, error out=w1365:errorcluster, "FP.State"=w1363:T7)
            n521 = Not Equal?(x=w1363, y=w1361) -> (x != y?=w1362:bool)
            n522 = case shown="True" w1362 {
              tunnel: [w1372 w1373] -> w1368
              tunnel: w1365 -> [w1371 w1373]
              tunnel: w1364 -> [w1370 _]
              tunnel: w1361 -> [w1369 _]
              frame True {
                n523 = invoke class="VI" method="FP.Open"(reference=w1370, error in=w1371, "State"=w1369) -> (error out=w1372:errorcluster)  [unwired: 2 in, 4 out]
              }
              frame False {
              }
            }
          }
        }
        n524 = call <vilib>:"Add State(s) to Queue__JKI_lib_State_Machine.vi"("State(s) in (\"\")"=w1308) -> ("States Out"=w1307:string)  [unwired: 14 in]
      }
      frame "---------- Macro ----------" {
        # "Do not put any code in this frame.\n(It is a separator no-op. You can make a copy of this frame to create a new Macro frame)"
        n525 = call <vilib>:"Add State(s) to Queue__JKI_lib_State_Machine.vi"("State(s) in (\"\")"=w1377) -> ("States Out"=w1376:string)  [unwired: 14 in]
      }
      frame "Macro: Initialize" {
        w1393 = "Data: Initialize\nInitialize Core Data\nUI: Initialize\nUI: Front Panel State >> Open"  # Data: Initialize Initialize Core Data UI: Initialize UI: Front Panel State >> Open
        # "Initialization Macro\n(This is called once, when the VI starts)"
        n526 = local read "Thermocouple"() -> (w1379:cluster{"String":string, "Scalar":sgl}[])
        n527 = disable-structure shown="Disabled" {
          frame Disabled {
            n528 = local read "9220 AI  Volt  Pressure"() -> ()  [unwired: 1 out]
            n529 = local read "Thermocouple"() -> ()  [unwired: 1 out]
          }
          frame Enabled {
          }
        }
        n530 = local read "9220 AI  Volt  Pressure"() -> (w1381:cluster{"String":string, "Scalar":sgl}[])
        n531 = for {
          tunnel: w1379 -> [w1398] mode=indexing
          tunnel: [w1397] -> w1378 mode=indexing
          n532 = Unbundle By Name(w1398) -> ("String"=w1397:string)
        }
        n533 = for {
          tunnel: w1381 -> [w1400] mode=indexing
          tunnel: [w1399] -> w1380 mode=indexing
          n534 = Unbundle By Name(w1400) -> ("String"=w1399:string)
        }
        n535 = Build Array (concatenate)(string[] ["Time", "Throttle % ", "Speed Summary", "Torque Summary", "Power", "Gear Ratio", "Engine Speed", "Engine Torque", "L Speed", "R Speed", "H Speed", "L Torque ", "R Torque ", "H Torque "] ("array w/ subset deleted 2"), w1378, w1380) -> (w1382:string[])
        n536 = call <vilib>:"Application Directory.vi"() -> ("Application Directory"=w1391:path)
        n537 = Build Path(base path=w1391, name or relative path="Data\\Header column.txt") -> (appended path=w1389:path)
        n538 = call "Header Column FGV.vi"("Column initilization"=w1382, "Command"=T6."Initialise", "error in (no error)"=w1385, "File Path"=w1389) -> ("error out"=w1387:errorcluster)  [unwired: 6 in, 1 out]
        n539 = call "Header Column FGV.vi"("Command"=T6."Read Data", "error in (no error)"=w1387) -> ("error out"=w1384:errorcluster, "Column Header"=w1386:string[])  [unwired: 8 in]
        n540 = local write "Column Header"(w1386) -> ()
        n541 = call <vilib>:"Add State(s) to Queue__JKI_lib_State_Machine.vi"("State(s) in Front (\"\")"=w1393, "State(s) in (\"\")"=w1396) -> ("States Out"=w1395:string)  [unwired: 13 in]
      }
      frame "Macro: Exit" {
        # "Exit Macro\n(This is called once, when the VI exits)"
        n542 = Unbundle By Name(w1410) -> ("Core.Close Panel on Exit?"=w1409:bool)
        n543 = Select(t="UI: Front Panel State >> Close", s=w1409, f="") -> (s? t:f=w1406:string)
        n544 = call <vilib>:"Add State(s) to Queue__JKI_lib_State_Machine.vi"("State(s) in (\"\")"=w1406, "State(s) at Back (\"\")"="Data: Cleanup\nExit") -> ("States Out"=w1404:string)  [unwired: 13 in]
        n545 = call "Header Column FGV.vi"("Command"=T6."Close", "error in (no error)"=w1402) -> ("error out"=w1401:errorcluster)  [unwired: 8 in, 1 out]
        n546 = call <vilib>:"Add State(s) to Queue__JKI_lib_State_Machine.vi"("State(s) in Front (\"\")"=w1404, "State(s) in (\"\")"=w1412) -> ("States Out"=w1411:string)  [unwired: 13 in]
      }
      frame "---------- New Category ----------" {
        # "Template Separator\n(You can make a copy of, or modify, this frame)"
        n547 = call <vilib>:"Add State(s) to Queue__JKI_lib_State_Machine.vi"("State(s) in (\"\")"=w1416) -> ("States Out"=w1415:string)  [unwired: 14 in]
      }
      frame "Monitor Data" {
      }
      frame "Check Limits" {
        n548 = call <vilib>:"Add State(s) to Queue__JKI_lib_State_Machine.vi"("State(s) in (\"\")"=w1423) -> ("States Out"=w1422:string)  [unwired: 14 in]
      }
      frame "Update  Limit Status" {
        n549 = disable-structure shown="Enabled" {
          disable-tunnel: w1426 -> [w1440 _]
          disable-tunnel: w1425 -> [w1431 w1448]
          disable-tunnel: [w1430 w1448] -> w1424
          frame Disabled {
            w1429 = bool[] []  # In Range
            n550 = Unbundle By Name(w1440) -> ("Intercooler_In_T"=w1439:refnum<vi>, "Coolant_Inlet_T"=w1438:refnum<vi>, "Coolant_Outlet_T"=w1437:refnum<vi>, "Basement_T"=w1436:refnum<vi>, "Exhaust_T"=w1435:refnum<vi>, "Oil_T"=w1434:refnum<vi>, "Intercooler_Out_T"=w1433:refnum<vi>)
            n551 = Build Array(w1439, w1438, w1437, w1436, w1435, w1434, w1433) -> (w1432:refnum<vi>[])
            n552 = for {
              tunnel: w1432 -> [w1447] mode=indexing
              shift-right: [w1445] -> w1430
              shift-left: w1431 -> [w1446]
              tunnel: w1429 -> [w1444] mode=indexing
              n553 = Select(t=u32 6618880, s=w1444, f=u32 13117952) -> (s? t:f=w1443:u32)
              n554 = property class="Slide (strict)"(reference=w1447, error in=w1446, "BGColor"=w1443) -> (error out=w1445:errorcluster)  [unwired: 1 out]
            }
          }
          frame Enabled {
          }
        }
        n555 = call <vilib>:"Add State(s) to Queue__JKI_lib_State_Machine.vi"("State(s) in (\"\")"=w1428) -> ("States Out"=w1427:string)  [unwired: 14 in]
      }
      frame "Write Headers" {
        (unwired) string[] ["Time", "Throttle % ", "Speed Summary", "Torque Summary", "Power", "Gear Ratio", "H Dyno Speed", "H Dyno Torque", "L Speed", "R Speed", "H Speed", "L Torque ", "R Torque ", "H Torque "] ("array w/ subset deleted 2")
        # "DC Voltage"
        # "Ph 3 Voltage"
        # "# EDIT"
        n556 = disable-structure shown="Disabled" {
          frame Disabled {
            n557 = local read "9220 AI  Volt  Pressure"() -> ()  [unwired: 1 out]
            n558 = local read "Thermocouple"() -> ()  [unwired: 1 out]
          }
          frame Enabled {
          }
        }
        n559 = call "READ CAN DATA.vi"("Enum"=READ_CAN_DATA."GET") -> ("READ DATA OUT"=w1463:T19[])  [unwired: 9 in, 1 out]
        n560 = call "WRITE CAN DATA.vi"("Enum"=READ_CAN_DATA."GET") -> ("READ DATA OUT"=w1462:T19[])  [unwired: 10 in]
        n561 = for {
          tunnel: w1463 -> [w1518] mode=indexing
          tunnel: [w1513] -> w1458 mode=indexing
          n562 = Unbundle By Name(w1518) -> ("FUNCTION"=w1516:string)
          n563 = Search and Replace String(replace all?=TRUE ("replace all? (F)"), input string=w1516, search string="\n", replace string="" ("replace string (\"\")")) -> (result string=w1513:string)  [unwired: 4 in, 3 out]
        }
        n564 = for {
          tunnel: w1462 -> [w1512] mode=indexing
          tunnel: [w1508] -> w1459 mode=indexing
          n565 = Unbundle By Name(w1512) -> ("FUNCTION"=w1510:string)
          n566 = Search and Replace String(replace all?=TRUE ("replace all? (F)"), input string=w1510, search string="\n", replace string="" ("replace string (\"\")")) -> (result string=w1508:string)  [unwired: 4 in, 3 out]
        }
        n567 = Format Date/Time String(time format string (%c)="%I %M %S") -> (date/time string=w1466:string)  [unwired: 2 in]
        n568 = Concatenate Strings("D", ":\\DataLog\\%Y\\%m\\%d") -> (w1475:string)
        n569 = Format Date/Time String(time format string (%c)=w1475) -> (date/time string=w1474:string)  [unwired: 2 in]
        n570 = call "Power Analyser FGV Enable.vi"("Enum"=Power_Analyser_Enum."READ") -> ("Enable Out"=w1456:bool)  [unwired: 10 in]
        n571 = Concatenate Strings("File Tag", w1466, ".csv" ("string")) -> (w1472:string)
        n572 = String To Path(string=w1474) -> (path=w1471:path)
        n573 = call "Create Directory Structure.vi"("Dir Path In"=w1471) -> ("Dir Path Out"=w1470:path)  [unwired: 3 in, 1 out]
        n574 = call "Get Data Log Configuratuion.vi"("error in (no error)"=w1484) -> ("error out"=w1483:errorcluster, "Log Active"=w1478:bool[][], "Log Headers"=w1481:string[])  [unwired: 8 in]
        n575 = Build Path(base path=w1470, name or relative path=w1472) -> (appended path=w1454:path)
        n576 = local read "Thermocouple"() -> (w1450:cluster{"String":string, "Scalar":sgl}[])
        n577 = for {
          tunnel: w1450 -> [w1489] mode=indexing
          tunnel: [w1488] -> w1449 mode=indexing
          n578 = Unbundle By Name(w1489) -> ("String"=w1488:string)
        }
        n579 = local read "9220 AI  Volt  Pressure"() -> (w1452:cluster{"String":string, "Scalar":sgl}[])
        n580 = for {
          tunnel: w1452 -> [w1491] mode=indexing
          tunnel: [w1490] -> w1451 mode=indexing
          n581 = Unbundle By Name(w1491) -> ("String"=w1490:string)
        }
        n582 = case shown="False" w1456 {
          tunnel: w1449 -> [w1499 w1506]
          tunnel: w1451 -> [w1498 w1505]
          tunnel: string[] ["Time", "Throttle % ", "Set Speed", "Speed Summary", "Torque Summary", "Power", "Gear Ratio", "H Motor Speed", "H Motor Torque", "L Speed", "R Speed", "H Speed", "L Torque ", "R Torque ", "H Torque "] ("array w/ subset deleted 2") -> [w1497 w1504]
          tunnel: string[] ["Ph 1 Voltage", "Ph 2 Voltage", "Ph 3 Voltage", "DC Voltage", "Votlage 123", "Ph 1 Current", "Ph 2 Current", "Ph 3 Current", "DC Current", "Currrent 123", "Ph 1 power", "Ph 2 power", "Ph 3 power", "DC power", "P123", "Ph 1 Freq", "Ph 2 Freq", "Ph 3 Freq"] -> [w1496 _]
          tunnel: [w1495 w1503] -> w1453
          tunnel: w1459 -> [w1494 w1502]
          tunnel: w1458 -> [w1493 w1501]
          tunnel: string[] ["HVHC SELECTION", "CONTROL SELECTION", "VOLTAGE", "CURRENT", "POWER"] -> [w1492 w1500]
          frame True {
            n583 = Build Array (concatenate)(w1497, w1499, w1498, w1496, w1494, w1493, w1492) -> (w1495:string[])
          }
          frame False {
            n584 = Build Array (concatenate)(w1504, w1506, w1505, w1502, w1501, w1500) -> (w1503:string[])
          }
        }
        n585 = call "Write Headers to CSV File.vi"("Array"=w1453, "error in (no error)"=w1483, "Headers"=w1481, "file path"=w1454) -> ("error out"=w1482:errorcluster, "LogFile Refnum"=w1469:refnum<file>)  [unwired: 6 in]
        n586 = Bundle By Name(cluster=w1480, "location"=w1454, "LogFile Refnum"=w1469, "Log Active"=w1478) -> (w1479:T18)
        n587 = call <vilib>:"Add State(s) to Queue__JKI_lib_State_Machine.vi"("State(s) in (\"\")"=w1486, "State(s) at Back (\"\")"="Log Data" ("State(s) at Back (\"\")")) -> ("States Out"=w1487:string)  [unwired: 13 in]
      }
      frame "Log Data" {
        n588 = local read "Mean"() -> (w1568:sgl[])
        n589 = call "Power Analyser FGV Enable.vi"("Enum"=Power_Analyser_Enum."READ") -> ("Enable Out"=w1528:bool)  [unwired: 10 in]
        n590 = local read "PA Data"() -> (w1541:dbl[])
        n591 = local read "Mean tc"() -> (w1577:sgl[])
        n592 = Unbundle By Name(w1598) -> ("LogFile Refnum"=w1601:refnum<file>, "Log Active"=w1586:bool[][])
        n593 = global read "Throttle.vi" "DAT DOUBLE"() -> (w1544:dbl[])
        n594 = global read "Throttle.vi" "Throttle %"() -> (w1546:fxp<+/-,34,12>)
        n595 = local read "speed torque power"() -> (w1564:dbl[])
        n596 = global read "Throttle.vi" "rpm torque"() -> (w1545:dbl[])
        n597 = Index Array(array=w1568, index #1=4 ("index")) -> (element #1=w1569:sgl, element #2=w1570:sgl, element #3=w1571:sgl, element #4=w1572:sgl, element #5=w1573:sgl, element #6=w1574:sgl, element #7=w1575:sgl, element #8=w1576:sgl, element #9=w1563:sgl, element #10=w1562:sgl, element #11=w1561:sgl, element #12=w1552:sgl, element #13=w1550:sgl, element #14=w1549:sgl, element #15=w1548:sgl, element #16=w1547:sgl)  [unwired: 15 in]
        n598 = Index Array(array=w1577) -> (element #1=w1578:sgl, element #2=w1579:sgl, element #3=w1580:sgl, element #4=w1581:sgl, element #5=w1582:sgl, element #6=w1583:sgl, element #7=w1584:sgl, element #8=w1560:sgl, element #9=w1559:sgl, element #10=w1558:sgl, element #11=w1557:sgl, element #12=w1556:sgl, element #13=w1555:sgl, element #14=w1554:sgl, element #15=w1553:sgl, element #16=w1551:sgl)  [unwired: 16 in]
        n599 = Delete From Array(array=w1541, length=18 ("index"), index=0 ("length")) -> (deleted portion=w1527:dbl[])  [unwired: 1 out]
        "deleted portion" <- w1527
        n600 = To Double Precision Float(number=w1546) -> (double precision float=w1566:dbl)
        n601 = Build Array(w1578, w1579, w1580, w1581, w1582, w1583, w1584, w1560, w1559, w1558, w1557, w1556, w1555, w1554, w1553, w1551) -> (w1565:sgl[])
        n602 = Build Array(w1569, w1570, w1571, w1572, w1573, w1574, w1575, w1576, w1563, w1562, w1561, w1552, w1550, w1549, w1548, w1547) -> (w1532:sgl[])
        n603 = Index Array(array=w1544, index=6) -> (element=w1542:dbl)
        n604 = disable-structure "old logic" shown="Disabled" {
          disable-tunnel: w1586 -> [w1621 _]
          frame Disabled {
            n605 = shared-variable "My Computer\\test_1.lvlib\\Data_Double"() -> (w1623:dbl[])  [unwired: 1 in, 1 out]
            n606 = local read "RAW Mean TC"() -> (w1625:sgl[])
            n607 = local read "RAW Mean"() -> (w1626:sgl[])
            n608 = local read "Mean"() -> (w1629:sgl[])
            n609 = local read "Mean tc"() -> (w1628:sgl[])
            n610 = To Single Precision Float(number=w1623) -> (single precision float=w1622:sgl[])
            n611 = Build Array (concatenate)(w1626, w1625) -> (w1624:sgl[])
            n612 = Build Array (concatenate)(w1629, w1628, w1622) -> (w1627:sgl[])
            n613 = call "Select Log Data.vi"("Log Active"=w1621, "Scaled"=w1627, "Raw"=w1624) -> ()  [unwired: 7 in, 2 out]
          }
          frame Enabled {
          }
        }
        n614 = case shown="True" w1528 {
          tunnel: [w1611 w1618] -> w1585
          tunnel: w1566 -> [w1610 w1617]
          tunnel: w1565 -> [w1609 w1616]
          tunnel: w1564 -> [w1608 w1615]
          tunnel: w1545 -> [w1607 w1614]
          tunnel: w1542 -> [w1606 w1613]
          tunnel: w1527 -> [w1605 _]
          tunnel: w1532 -> [w1604 w1612]
          frame True {
            n615 = Build Array (concatenate)(w1610, w1606, w1608, w1607, w1609, w1604, w1605) -> (w1611:dbl[])
          }
          frame False {
            n616 = Build Array (concatenate)(w1617, w1613, w1615, w1614, w1616, w1612) -> (w1618:dbl[])
          }
        }
        n617 = call "READ CAN DATA.vi"("Enum"=READ_CAN_DATA."GET") -> ("READ DATA OUT"=w1539:T19[])  [unwired: 9 in, 1 out]
        n618 = call "WRITE CAN DATA DBL.vi"("Enum"=READ_CAN_DATA."GET") -> ("CAN DATA OUT"=w1522:dbl[])  [unwired: 9 in, 1 out]
        n619 = for {
          tunnel: w1539 -> [w1620] mode=indexing
          tunnel: [w1619] -> w1536 mode=indexing
          n620 = Unbundle By Name(w1620) -> ("DATA"=w1619:string)
        }
        n621 = call "READ DUBAS DATALOG.vi"("STATES"=DUBAS_DTALOG_FGV_STATES."READ DATA") -> ("DUBAS DATA OUT"=w1525:string[])  [unwired: 9 in, 1 out]
        n622 = Number To Fractional String(number=w1585, precision (6)=i16 6) -> (F-format string=w1537:string[])  [unwired: 2 in]
        n623 = Format Date/Time String(time format string (%c)="%Y%m%d_%H%M%S") -> (date/time string=w1594:string)  [unwired: 2 in]
        n624 = Delete From Array(array=w1522, length=2) -> (deleted portion=→"deleted portion 2":dbl[], array with subset deleted=w1521:dbl[])  [unwired: 1 in]
        n625 = Number To Fractional String(number=w1521, precision (6)=i16 2) -> (F-format string=w1533:string[])  [unwired: 2 in]
        n626 = Build Array (concatenate)(w1537, w1533, w1536, w1525) -> (w1538:string[])
        n627 = Build Array (concatenate)(w1594, w1538) -> (w1523:string[])
        n628 = Build Array(w1523) -> (w1524:string[][])
        n629 = Array To Spreadsheet String(delimiter (Tab)=",", array=w1524, 3:"%s" ("format string")) -> (spreadsheet string=w1588:string)
        n630 = Write to Text File(file (use dialog)=w1601, text=w1588, error in=w1600) -> (refnum out=w1593:refnum<file>, error out=w1592:errorcluster)  [unwired: 1 in, 1 out]
        n631 = Set File Position(refnum=w1593, from (0:start)=enum16{"start", "end", "current"}."end", error in=w1592) -> (refnum out=w1597:refnum<file>, error out=w1599:errorcluster)  [unwired: 1 in]
        n632 = Bundle By Name(cluster=w1598, "LogFile Refnum"=w1597) -> (w1596:T18)
        n633 = call <vilib>:"Add State(s) to Queue__JKI_lib_State_Machine.vi"("State(s) in (\"\")"=w1602) -> ("States Out"=w1603:string)  [unwired: 14 in]
      }
      frame "Stop Logging" {
        n634 = Unbundle By Name(w1635) -> ("location"=w1633:path, "LogFile Refnum"=w1638:refnum<file>)
        n635 = disable-structure shown="Enabled" {
          disable-tunnel: w1638 -> [w1644 w1646]
          disable-tunnel: w1637 -> [w1643 w1645]
          disable-tunnel: [w1642 w1645] -> w1636
          disable-tunnel: [w1641 w1646] -> w1634
          frame Disabled {
            n636 = Write to Text File(file (use dialog)=w1644, error in=w1643) -> (refnum out=w1641:refnum<file>, error out=w1642:errorcluster)  [unwired: 2 in, 1 out]
          }
          frame Enabled {
          }
        }
        n637 = Close File(refnum=w1634, error in=w1636) -> (error out=w1632:errorcluster)  [unwired: 1 out]
        n638 = call "Down Sample Data.vi"("Data log"="Data log", "error in (no error)"=w1632, "location"=w1633) -> ("error out"=w1631:errorcluster)  [unwired: 8 in]
        n639 = call <vilib>:"Add State(s) to Queue__JKI_lib_State_Machine.vi"("State(s) in (\"\")"=w1639) -> ("States Out"=w1640:string)  [unwired: 14 in]
      }
    }
    n640 = call "Application Stop.vi"("Command"=enum16{"Read ", "Write "}."Read ") -> ("STOP"=w1057:bool)  [unwired: 9 in, 1 out]
    "STOP BOTH APP" <- w1057
    n641 = Or(x=w1057, y=w1059) -> (x .or. y?=w1058:bool)
  }
  n642 = Release Queue(queue=w26, error in (no error)=w25) -> ()  [unwired: 1 in, 3 out]
  n643 = Release Queue(queue=w61, error in (no error)=w62) -> ()  [unwired: 1 in, 3 out]
  n644 = xnode "Close FPGA VI Reference"("FPGA VI Reference In"=w63, "error in"=w60) -> ("error out"=w67:errorcluster)
  n645 = call "Power Analyser FGV Enable.vi"("Enum"=Power_Analyser_Enum."READ") -> ("Enable Out"=w54:bool)  [unwired: 10 in]
  n646 = case shown="True" w54 {
    tunnel: w64 -> [w1647 w1649]
    tunnel: [w1647 w1648] -> w14
    frame False {
    }
    frame True {
      n647 = call "FGV_READ.vi"("States"=States."Close Comm", "error in"=w1649) -> ("error out"=w1648:errorcluster)  [unwired: 8 in, 1 out]
    }
  }
  n648 = call <vilib>:"Clear Errors.vi"("error in (no error)"=w14) -> ("error out"=w13:errorcluster)  [unwired: 5 in, 1 out]
  n649 = call "READ DUBAS DATA.vi"("STATES"=DUBAS_FGV_STATES."CLOSE", "error in (no error)"=w13) -> ("error out"=w12:errorcluster)  [unwired: 8 in, 1 out]
  n650 = Merge Errors(w79, w67, w12) -> (w66:errorcluster)
  "error out" <- w66
  n651 = flat-sequence {
    tunnel: w66 -> [w1653]
    tunnel: [w1651] -> _
    frame #0 {
      n652 = call "Header Column FGV.vi"("Command"=T6."Close", "error in (no error)"=w1653) -> ("error out"=w1652:errorcluster)  [unwired: 8 in, 1 out]
      n653 = call "Gare ratio save FGV.vi"("Command"=T6."Close", "error in (no error)"=w1652) -> ("error out"=w1651:errorcluster)  [unwired: 8 in, 1 out]
    }
  }
